vi "BRig_RT_start_v1,14.vi"() -> ()   [LabVIEW 2014]
uses:
  <vilib>/Platform/TimedLoop/XDataNode/XDataNode.xnode
  <vilib>/Platform/TimedLoop/XDataNode/nitl_modes.ctl
  <vilib>/Platform/TimedLoop/XDataNode/XDNodeRunTimeDep.lvlib
  <vilib>/Platform/TimedLoop/XDataNode/wakeup.ctl
  <vilib>/Platform/TimedLoop/XDataNode/timing_clust.ctl
  <vilib>/rvi/interface/nirviReadWriteControl/nirviReadWriteControl.xnode
  <vilib>/rvi/interface/Simulation/niFpgaSimulationCallBeginRW.vi
  <vilib>/rvi/errors/niLvFpgaAdjustHostInterfaceError.vi
  <vilib>/rvi/interface/nirviCloseFPGA/nirviCloseFPGA.xnode
  <vilib>/myRIO/Instrument Drivers/Utilities/Utilities.lvlib
  <vilib>/rvi/interface/nirviOpenFPGA/nirviOpenFPGA.xnode
  myRIO_BRig_RT__Case_Exp_stateList.ctl
  myRIO_BRig_RT__Case_NonExp_stateList.ctl
  NiFpgaLv.dll
  <vilib>/Utility/error.llb/Error Cluster From Error Code.vi
  <vilib>/WebDAVClient/Advanced/SessionHandle.ctl
  <vilib>/WebDAVClient/NI_WebDAV.lvlib
  <vilib>/Utility/file.llb/Read From Spreadsheet File (I64).vi
  <vilib>/Utility/file.llb/Write To Spreadsheet File (DBL).vi
  <vilib>/FPGAPlugInAG/Dynamic/niLvFpga_Close_Dynamic.vi
  BRig_FPGA_v3,94__build.lvbitx
  BRig_FPGA_v3,94.vi
  <vilib>/FPGAPlugInAG/myRIO-1900/niLvFpga_Open_myRIO-1900.vi
  <vilib>/rvi/interface/common/dynamic/niFpgaDynamicAddResources.vi
panel:
  in  "LaserFiber_V_l2":dbl
  in  "LaserFiber_V_l1":dbl
  out "Solenoid R":bool
  out "Solenoid L":bool
  out "Laser2":bool
  out "Laser1":bool
  out "FreeReward_c_R":u16
  out "FreeReward_c_L":u16
  in  "Laser2_LED":bool
  in  "Laser1_LED":bool
  in  "lick_Rising(F)_or_Falling(T)":bool
  out "T_ExpRun_min":dbl
  out "stop_TimedLoop":bool
  out "BTPR_avg_R":dbl
  out "T2R_avg_R":dbl
  out "BTPR_avg_L":dbl
  out "T2R_avg_L":dbl
  out "BTPR_block":u16
  out "T2R_block":u16
  in  "comm_WebDAV_connect":bool
  in  "I_sendData":bool
  in  "comm_TCP_connect":bool
  out "nRewards_total":u16 caption="# Rewards in Current Block"
  out "BUR_target":u16 caption="Target Trials Per Block"
  in  "input_Threshold_reset":bool
  out "nTrial":u16
  out "allReward_R":bool
  out "allReward_L":bool
  out "Threshold":bool
  out "tLoop":dbl format="%#_2g"
  out "L_Power_l2":dbl
  out "comm_TCP":bool
  in  "get_countPerMS":bool
  out "SolenoidReward":bool
  out "L_Power_l1":dbl caption="LaserPower"
  in  "Recording":bool
  out "FPGA_count2ms":dbl=159.0
  out "error out":errorcluster
  out "cSpout":enum16{"Left", "Right"}(ring) caption="Left or Right Spout"
  out "A4":u32 caption="LickCounter_Right"
  out "A2":u32 caption="LickCounter_Left"
  out "nRewards_Right":u16 caption="# Rewards Total (Right)"
  out "nRewards_Left":u16 caption="# Rewards Total (Left)"
  out "nRewards_cur":u16 caption="# Rewards in Current Block"
  out "TpB_target":u16 caption="Target Trials Per Block"
  out "cState_NonExp":T1 caption="WarmUp State"
  out "iBlock":u16 caption="Current Block"
  out "cState":T2 caption="Experimental State"
  out "iTrial":u16 caption="Current Trial"
  in  "Data Set Prefix":string="Exp1_TM2"
  out "comm_WebDAV":bool
  in  "Host Password":string="sabalab"
  in  "Host UserName":string="Test2"
  in  "STOP_abort":bool caption="Stop LabView\n(Stops myRio and FPGA)"
  in  "STOP_endBlock":bool caption="Stop Experiment\n@ End of Block"
  in  "STOP_endTrial":bool caption="Stop Experiment\n@ End of Trial"
  in  "START":bool caption="Start Experiment"
  # "Experimental Run"
  # "Recording Rig"
  # "FPGA Conversion\n[counts per ms]"
  # "RealTime Cycle\nShould be <5ms"
  # "STOP experiment at"
  # "Exp Run Time"
  # "Reset"
  # "min"
  # "Communication with Host"
  # "Lick Counter"
  # "Block Target"
  # "Give Water?\n(Reward)"
  # "# Blocks"
  # "Experimental State"
  # "Left/Right"
  # "# Trials"
  # "# Rewards"
  # "Left           Right"
  # "Bad Trials\nPost Reward"
  # "Trials 2 Reward"
  # "Direction\n(NonSpecific Licking)"
  # "Block"
  # "Laser1"
  # "Laser2"
  # "# Trials"
  # "# Rewards"
  # "Current\nBlock"
  # "L          R"
  # "Power [V]"
  # "avg L"
  # "Toggle\nLED"
  # "Total"
  # "# Rewards"
  # "Laser Trigger"
  # "# Trials"
  # "avg R"
  # "1          2"
  # "Fiber Angle\n[V]"
  # "Left           Right"
  # "FreeRewards"
  # "Solenoid Trigger"
  # "WarmUp State"
  # "Lick Detection\nRising (F) or Falling (T)"
  # "L          R"
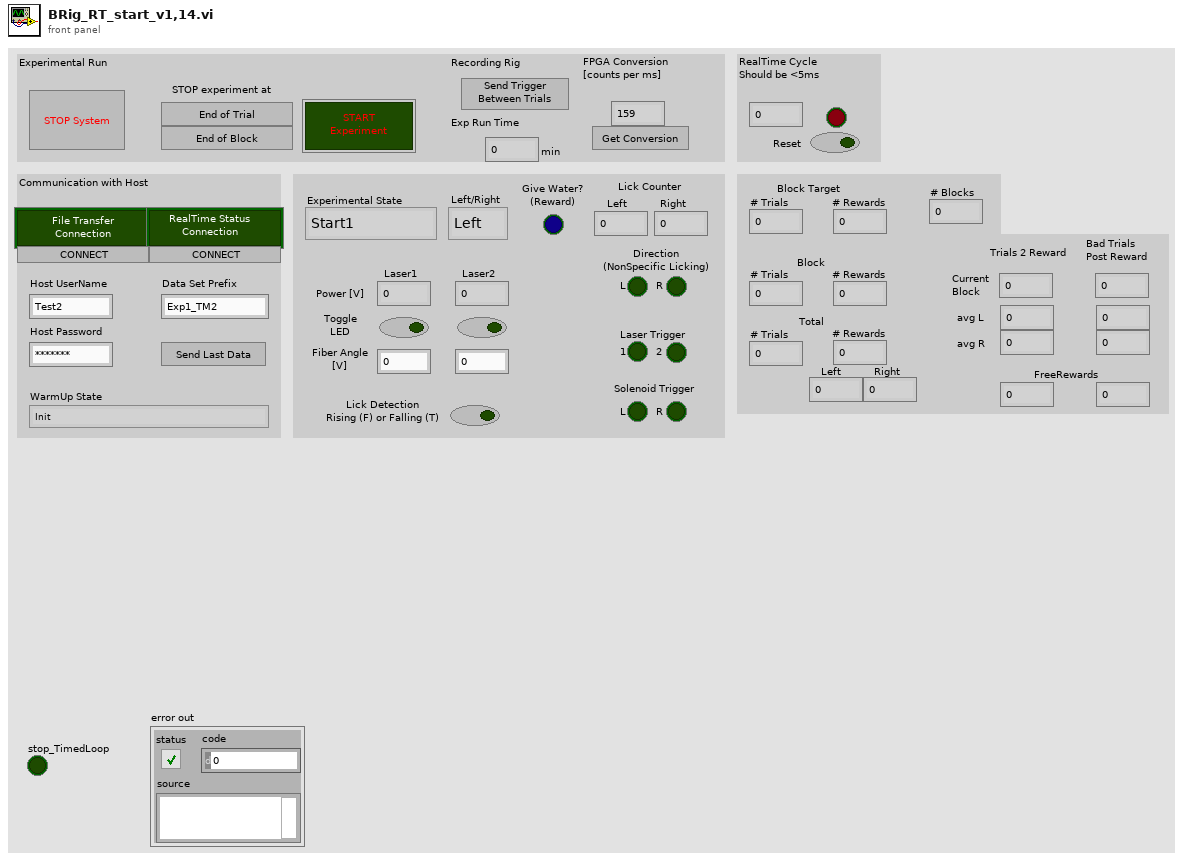
[diagram p1: front panel]
types:
  T1 = typedef "myRIO_BRig_RT__Case_NonExp_stateList.ctl" = enum16{"Init", "UploadSettings_pre", "UploadSettings_Read_dataExp", "UploadSettings_dataExp_1", "UploadSettings_dataExp_2", "UploadSettings_Read_dataLC", "UploadSettings_dataLC_1", "UploadSettings_dataLC_2", "UploadSettings_dataLC_3", "UploadSettings_dataLC_4", "UploadSettings_Read_dataMTrig", "UploadSettings_dataMTrig_1", "UploadSettings_post", "Idle_pre", "IdleEmpty", "IdleEmpty2", "IdleEmpty3", "IdleEmpty4", "Idle", "Idle_2", "Idle_3", "Idle_4", "Idle_5", "Idle_6", "Idle_post", "Cue_pre__pre", "Cue_pre", "Cue", "Cue_LED", "Cue_post", "RewardCalibration_pre", "RewardCalibration", "DispenseWater_pre__pre", "DispenseWater_pre", "DispenseWater", "DispenseWater_post", "TestConnection", "SendData", "Get_FPGA_count_per_ms", "End", "commTCP_connect"}
  T2 = typedef "myRIO_BRig_RT__Case_Exp_stateList.ctl" = enum16{"Start1", "Start2", "Start3", "saveSettings1", "saveSettings2", "saveSettings3", "saveSettings4", "saveSettings_LC_ENL_l1", "saveSettings_LC_ENL_l2", "saveSettings_LC_Cue_l1", "saveSettings_LC_Cue_l2", "saveSettings6_LC_l1_Other", "SaveSettings6_LC_l2_Other", "setSettings_Audio", "setSettings_Laser", "initBlock_pre", "initBlock", "initBlock2", "initBlock_post", "initTrial_pre", "initTrial", "initTrial2", "initTrial3", "initTrial4", "initTrial_LC_ENL1", "initTrial_LC_Cue1", "initTrial_LC_Cue1_2", "initTrial_LC_Sel", "initTrial_post", "ENL1_pre", "ENL1", "ENL1_post", "ENL1Penalty_pre", "ENL1Penalty", "ENL2_pre", "ENL2", "ENL2Penalty_pre", "ENL2Penalty", "Cue1_pre", "Cue1", "Cue1_post", "Cue1Penalty_pre", "Cue1Penalty", "Cue2_pre", "Cue2", "Cue2Penalty_pre", "Cue2Penalty", "Selection_pre", "Selection", "Select_post", "SelectReward_pre", "SelectReward", "SelectRewardPost_pre", "SelectRewardPost", "SelectWrong_pre", "SelectWrong", "SelectWrong_post", "SelectTimeout_pre", "SelectTimeout", "SelectTimeout_post", "endTrial_pre", "endTrial1", "endTrial2", "endTrial3", "endTrial_post", "endBlock_pre", "endBlock", "endBlock_post", "endExp", "commConnect", "commUpload_pre", "commUpload_dataBlock", "commUpload_dataCurrent", "commUpload_dataExp", "commUpload_dataLC", "commUpload_dataTrial", "commUpload_post", "saveData_pre", "saveData_dataBlock", "saveData_dataCurrent", "saveData_dataExp", "saveData_dataLC", "saveData_dataTrial", "saveData_post", "empty_endBlock1", "empty_endBlock2", "empty_endTrial1", "empty_endTrial2", "empty_endTrial3", "empty_endTrial4", "empty_endTrial5", "dummyState", "dummyState_endBlock", "FreeReward_pre", "FreeReward", "FreeRewardPost_pre", "FreeRewardPost"}
  T3 = enum8{"Enabled", "Disabled", "Disabled and Grayed Out"}
  T4 = typedef "NI_WebDAV.lvlib/SessionHandle.ctl" = refnum<k1>
  T5 = typedef "XDNodeRunTimeDep.lvlib/timing_clust.ctl" = cluster{"Expected End [f-1]":u64, "Actual End [f-1]":u64, "Finished Late? [f-1]":bool, "Expected End [i-1]":u64, "Actual End [i-1]":u64, "Finished Late? [i-1]":bool, "Expected Start [i]":u64, "Actual Start [i]":u64, "Expected Start [f]":u64, "Actual Start [f]":u64, "Source Name":string, "Structure Name":string, "Period":i64, "Deadline":i64, "Offset":i64, "Start":i64, "Priority":i32, "Timeout":i32, "Mode":T6, "Wakeup Reason":T7, "Error":errorcluster, "Source Type":string, "Secondary Source Type":string, "Global End Time":u64, "Global Start Time":u64, "Frame Duration":u64, "Iteration Duration":u64, "Assigned CPU":i32, "I/O Scan Engine Mode":u32}
  T6 = typedef "XDNodeRunTimeDep.lvlib/nitl_modes.ctl" = enum32{"No Change", "Process missed periods, maintain original phase", "Discard missed periods, maintain original phase", "Process missed periods, ignore original phase", "Discard missed periods, ignore original phase"}
  T7 = typedef "XDNodeRunTimeDep.lvlib/wakeup.ctl" = enum32{"Normal", "Aborted", "Asynchronous wakeup", "Timing source error", "Timed loop error", "Timeout"}
  T8 = cluster{"read mode":enum16{"polling", "blocking"}, "write mode":enum16{"polling", "blocking"}}
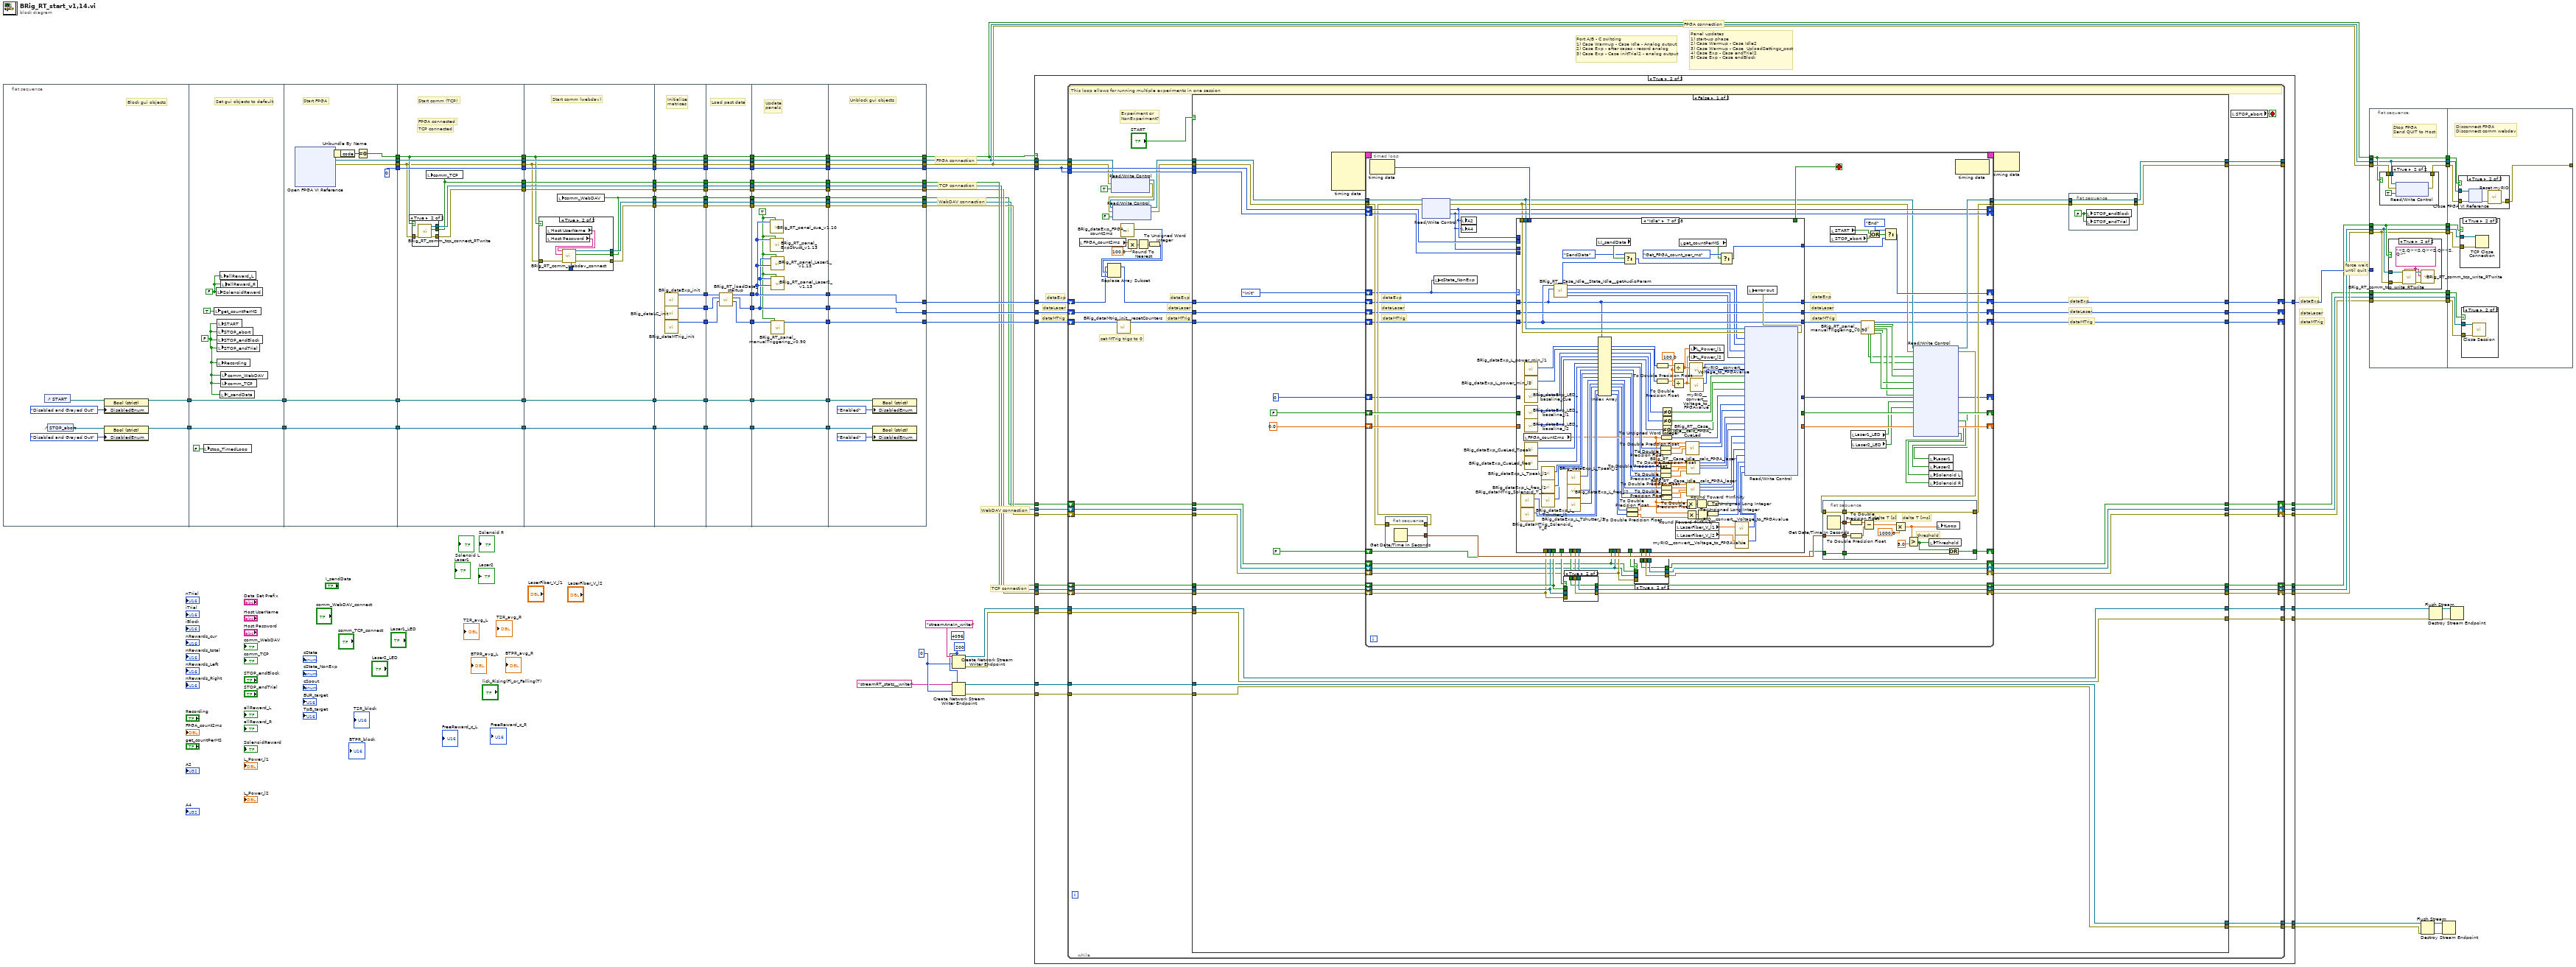
[diagram p0: block diagram]
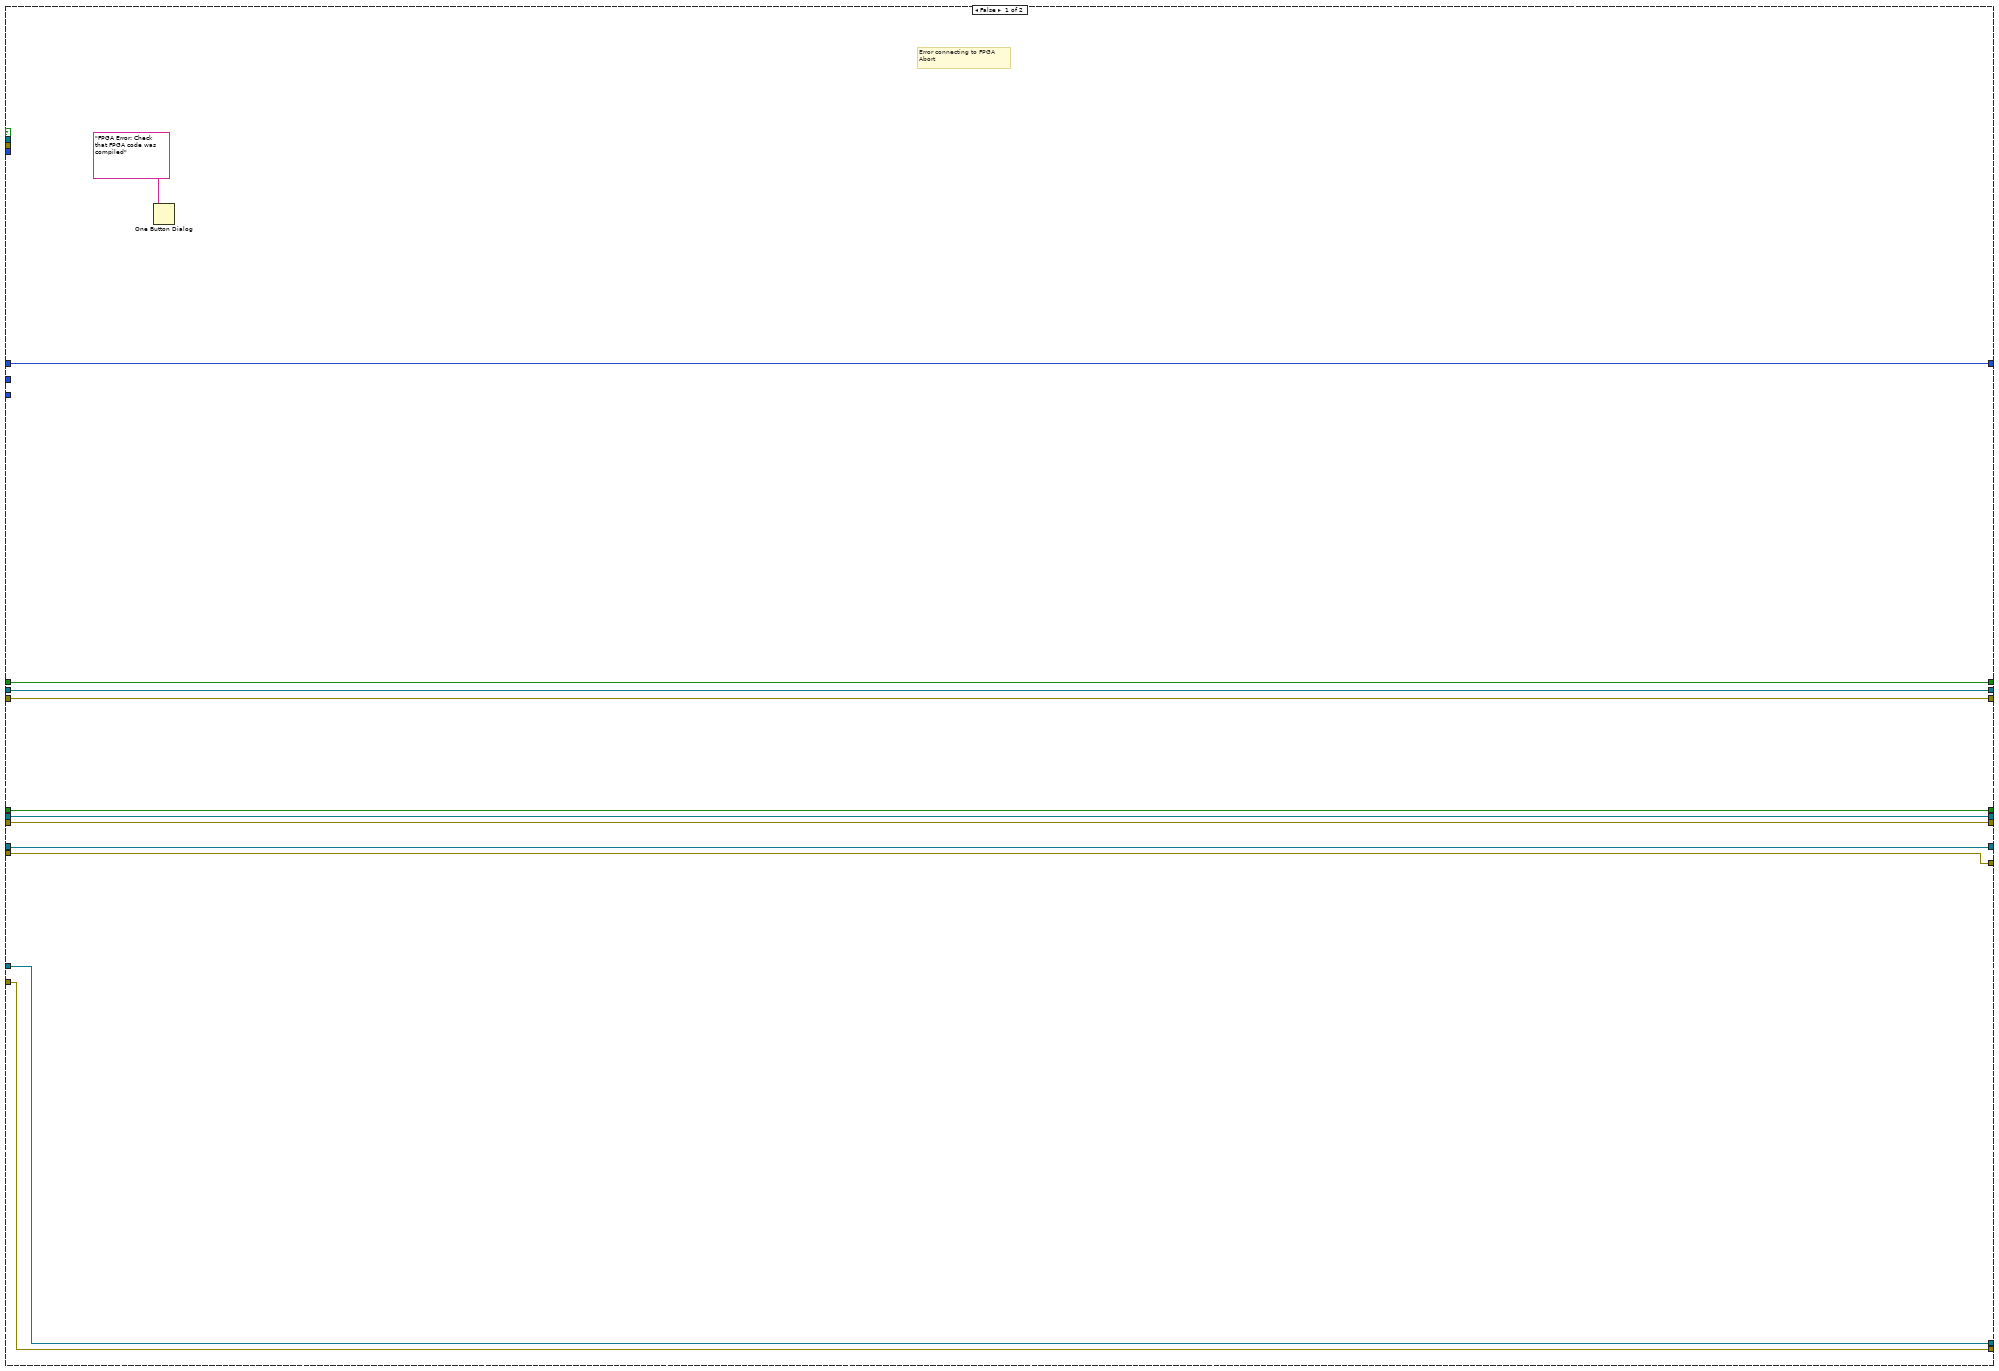
[diagram p2: hidden frame]
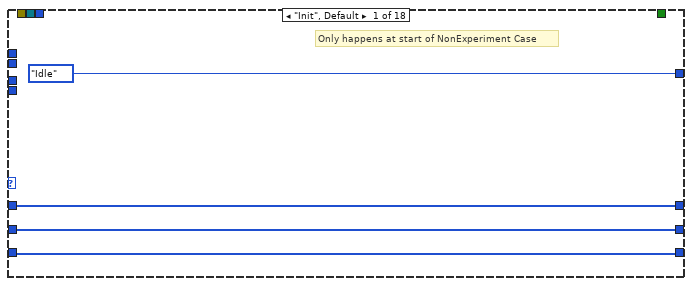
[diagram p5: hidden frame]
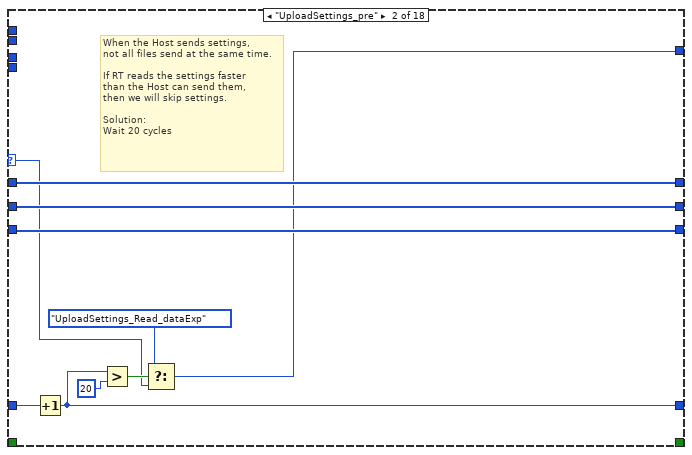
[diagram p6: hidden frame]
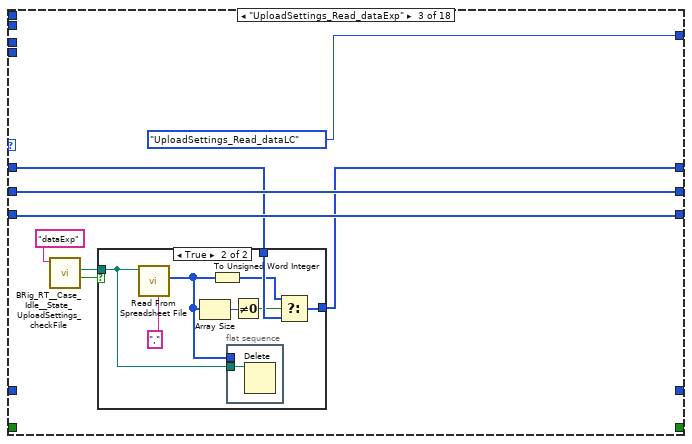
[diagram p7: hidden frame]
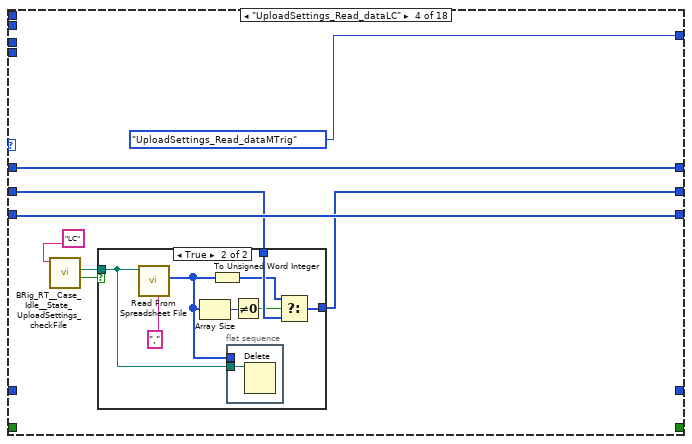
[diagram p9: hidden frame]
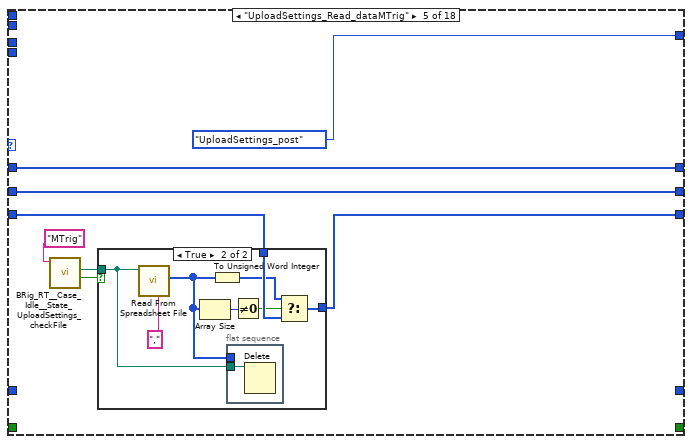
[diagram p11: hidden frame]
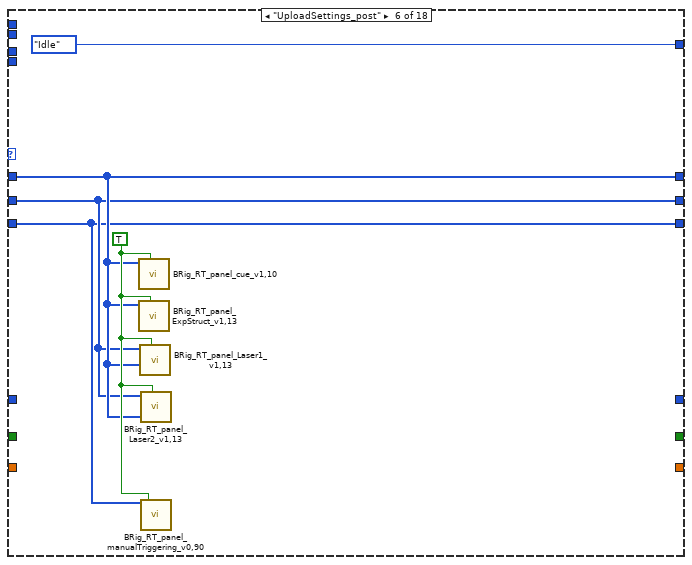
[diagram p13: hidden frame]
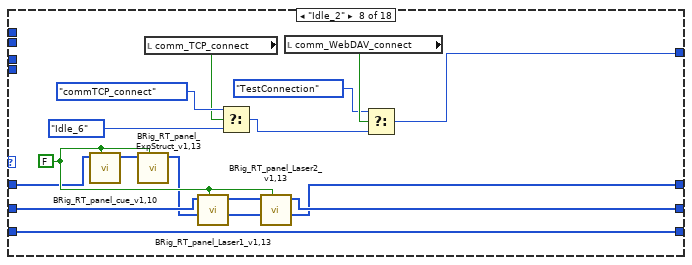
[diagram p14: hidden frame]
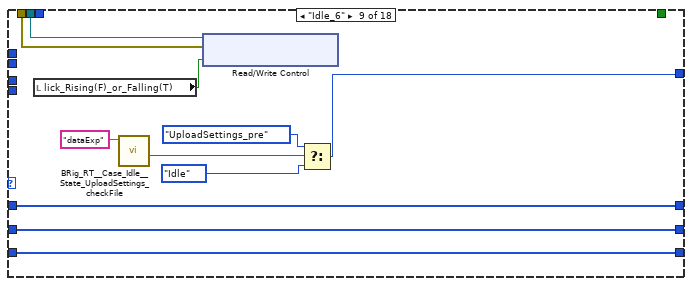
[diagram p15: hidden frame]
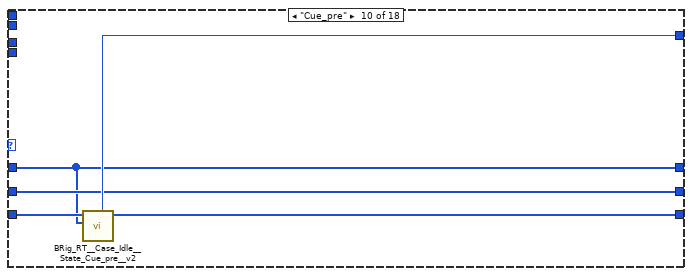
[diagram p16: hidden frame]
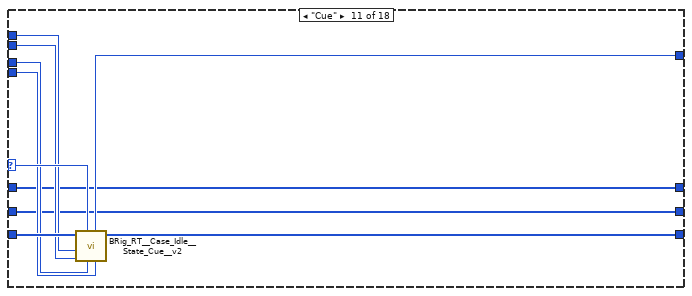
[diagram p17: hidden frame]
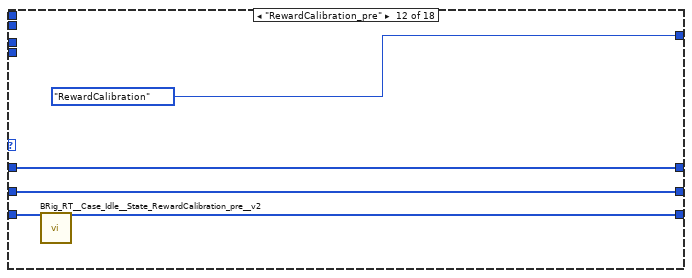
[diagram p18: hidden frame]
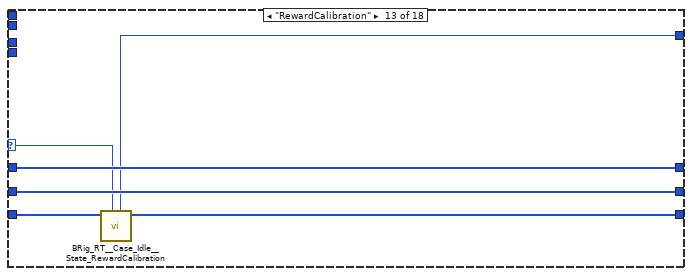
[diagram p19: hidden frame]
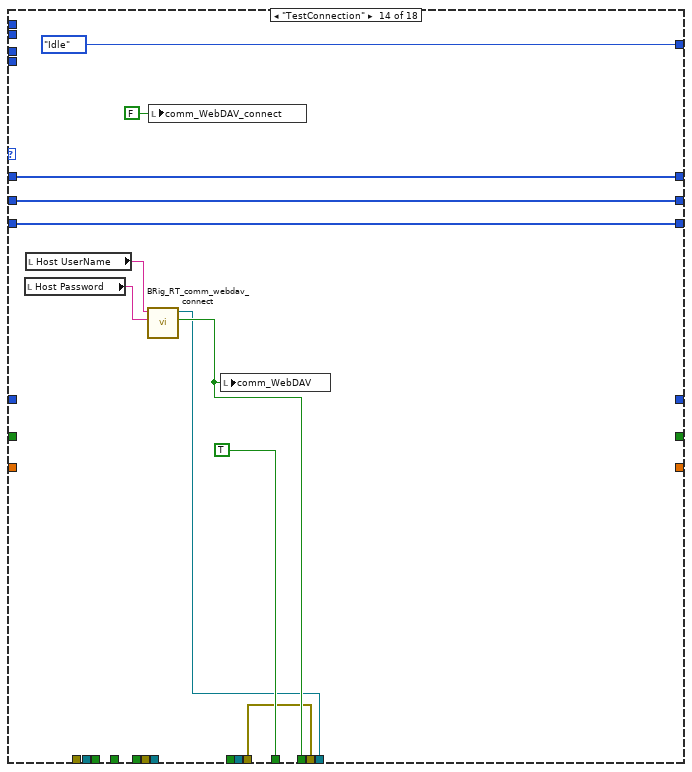
[diagram p20: hidden frame]
diagram:
  w8 = u16 0 ("element")
  (unwired) 4096 ("reader buffer size")
  w9 = 200 ("reader buffer size")
  # "Panel updates\n1) start-up phase\n2) Case Warmup - Case Idle2\n3) Case Warmup - Case  UploadSettings_post\n4) Case Exp - Case endTrial2\n5) Case Exp - Case endBlock"
  # "WebDAV connection"
  # "TCP connection"
  # "WebDAV connection"
  # "TCP connection"
  # "FPGA connection"
  # "FPGA connection"
  # "Port A/B - C switcing\n1) Case Warmup - Case Idle - Analog output\n2) Case Exp - after cases - record analog\n3) Case Exp - Case initTrial2 - analog output"
  # "force wait\nuntil quit"
  # "dataLaser"
  # "dataExp"
  # "dataMTrig"
  n1 = flat-sequence {
    tunnel: [w123] -> w106
    tunnel: [w122] -> w102
    tunnel: [w132] -> w107
    tunnel: w106 -> [w132]
    tunnel: [w131] -> w103
    tunnel: w102 -> [w131]
    tunnel: [w138] -> w120
    tunnel: [w140] -> w119
    tunnel: [u32 0] -> w118
    tunnel: [w136] -> w117
    tunnel: [w135] -> w108
    tunnel: w107 -> [w135]
    tunnel: [w134] -> w104
    tunnel: w103 -> [w134]
    tunnel: w120 -> [w146]
    tunnel: w119 -> [w149]
    tunnel: w118 -> [w148]
    tunnel: w117 -> [w147]
    tunnel: [w146] -> w116
    tunnel: [w149] -> w115
    tunnel: [w148] -> w114
    tunnel: [w147] -> w113
    tunnel: [w141] -> w112
    tunnel: [w145] -> w111
    tunnel: [w144] -> w110
    tunnel: [w143] -> w109
    tunnel: w108 -> [w143]
    tunnel: [w142] -> w105
    tunnel: w104 -> [w142]
    tunnel: w116 -> [w160]
    tunnel: w115 -> [w168]
    tunnel: w114 -> [w167]
    tunnel: w113 -> [w161]
    tunnel: w112 -> [w166]
    tunnel: w111 -> [w165]
    tunnel: w110 -> [w164]
    tunnel: [w160] -> w73
    tunnel: [w168] -> w72
    tunnel: [w167] -> w71
    tunnel: [w161] -> w70
    tunnel: [w166] -> w69
    tunnel: [w165] -> w68
    tunnel: [w164] -> w67
    tunnel: [w163] -> w66
    tunnel: w109 -> [w163]
    tunnel: [w162] -> w65
    tunnel: w105 -> [w162]
    tunnel: [w159] -> w64
    tunnel: [w157] -> w63
    tunnel: [w158] -> w62
    tunnel: w73 -> [w193]
    tunnel: [w193] -> w61
    tunnel: w72 -> [w192]
    tunnel: [w192] -> w60
    tunnel: w71 -> [w191]
    tunnel: [w191] -> w59
    tunnel: w70 -> [w190]
    tunnel: [w190] -> w58
    tunnel: w69 -> [w189]
    tunnel: [w189] -> w57
    tunnel: w68 -> [w188]
    tunnel: [w188] -> w56
    tunnel: w67 -> [w187]
    tunnel: [w187] -> w55
    tunnel: w66 -> [w186]
    tunnel: [w186] -> w54
    tunnel: w65 -> [w185]
    tunnel: [w185] -> w53
    tunnel: w64 -> [w184]
    tunnel: [w184] -> w52
    tunnel: w63 -> [w183]
    tunnel: [w183] -> w51
    tunnel: w62 -> [w182]
    tunnel: [w182] -> w50
    tunnel: [w181] -> w49
    tunnel: [w180] -> w48
    tunnel: [w179] -> w47
    tunnel: w61 -> [w211]
    tunnel: [w211] -> w46
    tunnel: w60 -> [w210]
    tunnel: [w210] -> w44
    tunnel: w59 -> [w209]
    tunnel: [w209] -> w42
    tunnel: w58 -> [w208]
    tunnel: [w208] -> w40
    tunnel: w57 -> [w207]
    tunnel: [w207] -> w38
    tunnel: w56 -> [w206]
    tunnel: [w206] -> w36
    tunnel: w55 -> [w205]
    tunnel: [w205] -> w34
    tunnel: w54 -> [w204]
    tunnel: [w204] -> w32
    tunnel: w53 -> [w203]
    tunnel: [w203] -> w30
    tunnel: w52 -> [w202]
    tunnel: [w202] -> w28
    tunnel: w51 -> [w201]
    tunnel: [w201] -> w26
    tunnel: w50 -> [w200]
    tunnel: [w200] -> w24
    tunnel: w49 -> [w195]
    tunnel: [w194] -> w22
    tunnel: w48 -> [w197]
    tunnel: [w196] -> w20
    tunnel: w47 -> [w199]
    tunnel: [w198] -> w19
    tunnel: w46 -> [w228]
    tunnel: [w228] -> w45
    tunnel: w44 -> [w227]
    tunnel: [w227] -> w43
    tunnel: w42 -> [w226]
    tunnel: [w226] -> w41
    tunnel: w40 -> [w225]
    tunnel: [w225] -> w39
    tunnel: w38 -> [w224]
    tunnel: [w224] -> w37
    tunnel: w36 -> [w223]
    tunnel: [w223] -> w35
    tunnel: w34 -> [w222]
    tunnel: [w222] -> w33
    tunnel: w32 -> [w221]
    tunnel: [w221] -> w31
    tunnel: w30 -> [w220]
    tunnel: [w220] -> w29
    tunnel: w28 -> [w219]
    tunnel: [w219] -> w27
    tunnel: w26 -> [w218]
    tunnel: [w218] -> w25
    tunnel: w24 -> [w217]
    tunnel: [w217] -> w23
    tunnel: w22 -> [w214]
    tunnel: [w213] -> w21
    tunnel: w20 -> [w215]
    tunnel: w19 -> [w216]
    tunnel: [w216] -> w18
    tunnel: [w215] -> w17
    tunnel: [w235] -> w83
    tunnel: [w236] -> w84
    tunnel: [w237] -> w85
    tunnel: [w242] -> w89
    tunnel: [w243] -> w121
    tunnel: [w244] -> w96
    tunnel: [w245] -> w95
    tunnel: w45 -> [w245]
    tunnel: w43 -> [w244]
    tunnel: w41 -> [w243]
    tunnel: w39 -> [w242]
    tunnel: w37 -> [w237]
    tunnel: w35 -> [w236]
    tunnel: w33 -> [w235]
    tunnel: w31 -> [w239]
    tunnel: w29 -> [w238]
    tunnel: w27 -> [w233]
    tunnel: w25 -> [w234]
    tunnel: w23 -> [w232]
    tunnel: [w234] -> w77
    tunnel: [w233] -> w78
    tunnel: [w232] -> w79
    tunnel: [w229] -> w92
    tunnel: [w230] -> w91
    tunnel: [w231] -> w90
    tunnel: w21 -> [w231]
    tunnel: w18 -> [w229]
    tunnel: w17 -> [w230]
    frame #0 {
      # "Block gui objects"
      n2 = control-ref of="START"() -> (w127:refnum<vi>)
      n3 = control-ref of="STOP_abort"() -> (w124:refnum<vi>)
      n4 = property class="Bool (strict)"(reference=w127, "DisabledEnum"=T3."Disabled and Grayed Out" ("Disabled")) -> (reference out=w123:refnum<vi>)  [unwired: 1 in, 1 out]
      n5 = property class="Bool (strict)"(reference=w124, "DisabledEnum"=T3."Disabled and Grayed Out" ("Disabled")) -> (reference out=w122:refnum<vi>)  [unwired: 1 in, 1 out]
    }
    frame #1 {
      w129 = FALSE ("SolenoidReward")
      w130 = FALSE
      # "Set gui objects to default"
      n6 = local write "stop_TimedLoop"(FALSE ("stop_TimedLoop")) -> ()
      n7 = local write "get_countPerMS"(TRUE ("get_countPerMS")) -> ()
      n8 = local write "SolenoidReward"(w129) -> ()
      n9 = local write "START"(w130) -> ()
      n10 = local write "STOP_abort"(w130) -> ()
      n11 = local write "STOP_endBlock"(w130) -> ()
      n12 = local write "STOP_endTrial"(w130) -> ()
      n13 = local write "Recording"(w130) -> ()
      n14 = local write "allReward_L"(w129) -> ()
      n15 = local write "I_sendData"(w130) -> ()
      n16 = local write "comm_WebDAV"(w130) -> ()
      n17 = local write "comm_TCP"(w130) -> ()
      n18 = local write "allReward_R"(w129) -> ()
    }
    frame #2 {
      # "Start FPGA"
      n19 = xnode "Open FPGA VI Reference"() -> ("FPGA VI Reference Out"=w140:refnum<k20>, "error out"=w138:errorcluster)  [unwired: 2 in]
      n20 = Unbundle By Name(w138) -> ("code"=w137:i32)
      n21 = Equal To 0?(x=w137) -> (x = 0?=w136:bool)
    }
    frame #3 {
      # "TCP connected"
      # "Start comm (TCP)"
      # "FPGA connected"
      n22 = case shown="True" w147 {
        selector: w147 -> [w150 _]
        tunnel: w146 -> [w152 w156]
        tunnel: [refnum<k5> refnum ("output_hTCP") w155] -> w145
        tunnel: [w150 w154] -> w141
        tunnel: [w152 w153] -> w144
        frame False {
        }
        frame True {
          n23 = call "BRig_RT_comm_tcp_connect_RTwrite.vi"("input_error"=w156) -> ("output_error"=w153:errorcluster, "output_connected"=w154:bool, "output_hTCP"=w155:refnum<k5>)  [unwired: 8 in]
        }
      }
      n24 = local write "comm_TCP"(w141) -> ()
    }
    frame #4 {
      # "Start comm (webdav)"
      n25 = case shown="True" w161 {
        selector: w161 -> [w170 _]
        tunnel: [w169 w176] -> w159
        tunnel: [w170 w175] -> w157
        tunnel: w160 -> [w171 w174]
        tunnel: [w171 w173] -> w158
        tunnel: [_ w172] -> _
        frame False {
          w169 = T4 refnum items=["Session NI_WebDAV"] ("output_hSession")
        }
        frame True {
          n26 = local read "Host UserName"() -> (w177:string)
          n27 = local read "Host Password"() -> (w178:string)
          n28 = call "BRig_RT_comm_webdav_connect.vi"("input_error"=w174, "input_password"=w178, "input_username"=w177) -> ("output_error"=w173:errorcluster, "output_Iconnected"=w175:bool, "output_hSession"=w176:T4, "output_code"=w172:u8)  [unwired: 5 in]
        }
      }
      n29 = local write "comm_WebDAV"(w157) -> ()
    }
    frame #5 {
      # "Initialize\nmatrices"
      n30 = call "BRig_dataExp_init.vi"() -> ("output_dataExp"=w179:u16[])  [unwired: 11 in]
      n31 = call "BRig_dataLC_init.vi"() -> ("output_dataLC"=w180:u16[])  [unwired: 11 in]
      n32 = call "BRig_dataMTrig_init.vi"() -> ("output_dataMTrig"=w181:u16[])  [unwired: 5 in]
    }
    frame #6 {
      # "Load past data"
      n33 = call "BRig_RT_loadData_startup.vi"("input_dataMTrig"=w195, "input_dataLC"=w197, "input_dataExp"=w199) -> ("output_dataMTrig"=w194:u16[], "output_dataLC"=w196:u16[], "output_dataExp"=w198:u16[])  [unwired: 6 in]
    }
    frame #7 {
      w212 = TRUE ("input_setValues")
      # "Update\npanels"
      n34 = call "BRig_RT_panel_cue_v1,10.vi"("input_setValues"=w212, "input_dataExp"=w216) -> ()  [unwired: 9 in, 1 out]
      n35 = call "BRig_RT_panel_ExpStruct_v1,13.vi"("input_setValues"=w212, "input_dataExp"=w216) -> ()  [unwired: 9 in, 1 out]
      n36 = call "BRig_RT_panel_Laser1_v1,13.vi"("input_setValues"=w212, "input_dataExp"=w216, "input_dataLC"=w215) -> ()  [unwired: 7 in, 2 out]
      n37 = call "BRig_RT_panel_Laser2_v1,13.vi"("input_setValues"=w212, "input_dataExp"=w216, "input_dataLC"=w215) -> ()  [unwired: 7 in, 2 out]
      n38 = call "BRig_RT_panel_manualTriggering_v0,90.vi"("input_dataMTrig"=w214, "input_setValues"=w212) -> ("output_dataMTrig"=w213:u16[])  [unwired: 10 in, 7 out]
    }
    frame #8 {
      # "Unblock gui objects"
      n39 = property class="Bool (strict)"(reference=w239, "DisabledEnum"=T3."Enabled" ("Disabled")) -> ()  [unwired: 1 in, 2 out]
      n40 = property class="Bool (strict)"(reference=w238, "DisabledEnum"=T3."Enabled" ("Disabled")) -> ()  [unwired: 1 in, 2 out]
    }
  }
  n41 = Create Network Stream Writer Endpoint(7:w9, 9:w8, 11:"streamAnaIn_writer" ("reader name")) -> (0:w10:errorcluster, 3:w11:refnum<k21>)  [unwired: 4 in]
  n42 = Create Network Stream Writer Endpoint(7:w9, 9:w8, 11:"streamRT_stats__writer" ("writer name")) -> (0:w5:errorcluster, 3:w6:refnum<k21>)  [unwired: 4 in]
  n43 = case shown="True" w89 {
    tunnel: w121 -> [_ w284]
    tunnel: w96 -> [_ w283]
    tunnel: w95 -> [_ w282]
    tunnel: [w257 w281] -> w93
    tunnel: w92 -> [w257 w280]
    tunnel: w91 -> [_ w279]
    tunnel: w90 -> [_ w278]
    tunnel: w85 -> [w256 w277]
    tunnel: w84 -> [w255 w276]
    tunnel: w83 -> [w254 w275]
    tunnel: [w256 w274] -> w82
    tunnel: [w255 w273] -> w81
    tunnel: [w254 w272] -> w80
    tunnel: w79 -> [w253 w271]
    tunnel: w78 -> [w252 w270]
    tunnel: w77 -> [w251 w269]
    tunnel: [w253 w268] -> w76
    tunnel: [w252 w267] -> w75
    tunnel: [w251 w266] -> w74
    tunnel: [w250 w265] -> w14
    tunnel: [w249 w264] -> w13
    tunnel: w11 -> [w250 w263]
    tunnel: w10 -> [w249 w262]
    tunnel: w6 -> [w247 w261]
    tunnel: w5 -> [w246 w260]
    tunnel: [w247 w259] -> w2
    tunnel: [w246 w258] -> w1
    frame False {
      # "Error connecting to FPGA\nAbort"
      n44 = One Button Dialog(message="FPGA Error: Check that FPGA code was compiled") -> ()  [unwired: 1 in, 1 out]
    }
    frame True {
      # "dataExp"
      # "dataLaser"
      # "dataMTrig"
      n45 = while {
        tunnel: w283 -> [w322]
        tunnel: w282 -> [w327]
        tunnel: w284 -> [w330]
        tunnel: w284 -> [w329]
        tunnel: [w320] -> _
        tunnel: [w319] -> _
        shift-right: [w318] -> _
        shift-left: w278 -> [w315]
        shift-right: [w316] -> _
        shift-left: w279 -> [w317]
        shift-right: [w286] -> w281
        shift-left: w280 -> [w295]
        shift-right: [w310] -> w274
        shift-left: w277 -> [w313]
        shift-right: [w309] -> w273
        shift-left: w276 -> [w312]
        shift-right: [w308] -> w272
        shift-left: w275 -> [w311]
        shift-right: [w304] -> w268
        shift-left: w271 -> [w307]
        shift-right: [w303] -> w267
        shift-left: w270 -> [w306]
        shift-right: [w302] -> w266
        shift-left: w269 -> [w305]
        tunnel: [w294] -> w265
        tunnel: [w293] -> w264
        tunnel: w263 -> [w292]
        tunnel: w262 -> [w291]
        tunnel: w261 -> [w290]
        tunnel: w260 -> [w289]
        tunnel: [w288] -> w259
        tunnel: [w287] -> w258
        stop <- w328 stop-if-true
        # "set MTrig trigs to 0"
        # "dataExp"
        # "dataLaser"
        # "dataMTrig"
        # "Experiment or\nNonExperiment?"
        # "This loop allows for running multiple experiments in one session"
        n46 = local read "FPGA_count2ms"() -> (w299:dbl)
        n47 = xnode "Read/Write Control"("FPGA VI Reference In"=w322, "error in"=w327, "Counts_Reset"=TRUE) -> ("FPGA VI Reference Out"=w324:refnum<k20>, "error out"=w325:errorcluster)
        n48 = xnode "Read/Write Control"("FPGA VI Reference In"=w324, "error in"=w325, "Counts_Reset"=FALSE) -> ("FPGA VI Reference Out"=w321:refnum<k20>, "error out"=w323:errorcluster)
        n49 = call "BRig_dataMtrig_init__resetCounters.vi"("input_dataMTrig"=w315) -> ("output_dataMTrig"=w314:u16[])  [unwired: 10 in]
        n50 = call "BRig_dataExp_FPGA_count2ms.vi"() -> ("output_FPGA_count2ms"=w300:i32)  [unwired: 11 in]
        n51 = Multiply(x=w299, y=100.0) -> (x*y=w297:dbl)
        n52 = Round To Nearest(number=w297) -> (nearest integer value=w296:dbl)
        n53 = To Unsigned Word Integer(number=w296) -> (unsigned 16bit integer=w301:u16)
        n54 = Replace Array Subset(array=w295, new element=w301, index=w300) -> (w285:u16[])
        n55 = case shown="False" "START" {
          tunnel: w330 -> [w366 w945]
          tunnel: w329 -> [w365 w944]
          tunnel: w323 -> [w363 w933]
          tunnel: w321 -> [w364 w934]
          tunnel: [w361 w942] -> w320
          tunnel: [w359 w911] -> w319
          tunnel: w314 -> [w355 w931]
          tunnel: [w354 w917] -> w318
          tunnel: w317 -> [w353 w881]
          tunnel: w285 -> [w333 w834]
          tunnel: [w352 w916] -> w316
          tunnel: [w351 w915] -> w286
          tunnel: w313 -> [w350 w925]
          tunnel: w312 -> [w349 w924]
          tunnel: w311 -> [w348 w923]
          tunnel: [w347 w900] -> w310
          tunnel: [w346 w899] -> w309
          tunnel: [w345 w898] -> w308
          tunnel: w307 -> [w344 w880]
          tunnel: w306 -> [w343 w879]
          tunnel: w305 -> [w342 w878]
          tunnel: [w341 w907] -> w304
          tunnel: [w340 w906] -> w303
          tunnel: [w339 w908] -> w302
          tunnel: w292 -> [w337 w839]
          tunnel: w291 -> [w336 w838]
          tunnel: [w337 w837] -> w294
          tunnel: [w336 w836] -> w293
          tunnel: w290 -> [w335 w830]
          tunnel: w289 -> [w334 w831]
          tunnel: [w335 w825] -> w288
          tunnel: [w334 w824] -> w287
          frame False {
            # "dataExp"
            # "dataLaser"
            # "dataMTrig"
            n56 = node-c288() -> (w369:T5)  [unwired: 4 in]
            n57 = timed-loop {
              timing: w369 -> [_]
              timing-out: [_] -> w368
              shift-right: [w437] -> _
              shift-left: myRIO_BRig_RT__Case_NonExp_stateList."Init" ("Enum") -> [w406]
              shift-right: [w435] -> _
              shift-left: w366 -> [w436]
              shift-right: [w433] -> _
              shift-left: w365 -> [w434]
              tunnel: [w443] -> w362
              tunnel: [w419] -> w360
              tunnel: w363 -> [w426]
              tunnel: w364 -> [w444]
              shift-right: [w429] -> _
              shift-left: FALSE -> [w430]
              shift-right: [w427] -> _
              shift-left: 0.0 -> [w428]
              shift-right: [w416] -> _
              shift-left: FALSE -> [w417]
              shift-right: [w415] -> w354
              shift-left: w355 -> [w407]
              shift-right: [w401] -> w351
              shift-left: w333 -> [w404]
              shift-right: [w402] -> w352
              shift-left: w353 -> [w403]
              shift-right: [w400] -> w347
              shift-left: w350 -> [w396]
              shift-right: [w399] -> w346
              shift-left: w349 -> [w395]
              shift-right: [w398] -> w345
              shift-left: w348 -> [w394]
              shift-right: [w384] -> w341
              shift-left: w344 -> [w390]
              shift-right: [w385] -> w340
              shift-left: w343 -> [w389]
              shift-right: [w386] -> w339
              shift-left: w342 -> [w388]
              shift-right: [w379] -> _
              shift-left: u16 0 ("y") -> [w380]
              stop <- w446 stop-if-true
              # "dataExp"
              # "dataLaser"
              # "dataExp"
              # "dataLaser"
              # "dataMTrig"
              # "dataMTrig"
              n58 = node-c288() -> (w445:i64)  [unwired: 1 in]
              n59 = flat-sequence {
                tunnel: w426 -> [w475]
                tunnel: [w476] -> w418
                tunnel: [w475] -> w425
                frame #0 {
                  n60 = Get Date/Time In Seconds() -> (seconds since 1Jan1904=w476:timestamp)
                }
              }
              n61 = xnode "Read/Write Control"("FPGA VI Reference In"=w444, "error in"=w425) -> ("FPGA VI Reference Out"=w432:refnum<k20>, "error out"=w431:errorcluster, "A2_LickL"=w435:u32, "A4_LickR"=w433:u32)
              n62 = local write "cState_NonExp"(w406) -> ()
              n63 = local write "A2"(w435) -> ()
              n64 = local write "A4"(w433) -> ()
              n65 = case shown="\"Idle\"" w406 {
                selector: w406 -> [_ w483 _ _ _ _ _ _ _ _ w678 _ w686 _ _ w730 w773 w779]
                tunnel: [myRIO_BRig_RT__Case_NonExp_stateList."Idle" ("Enum") w484 myRIO_BRig_RT__Case_NonExp_stateList."UploadSettings_Read_dataLC" ("t") myRIO_BRig_RT__Case_NonExp_stateList."UploadSettings_Read_dataMTrig" ("t") myRIO_BRig_RT__Case_NonExp_stateList."UploadSettings_post" ("t") myRIO_BRig_RT__Case_NonExp_stateList."Idle" ("t") w571 w641 w661 w667 w676 myRIO_BRig_RT__Case_NonExp_stateList."RewardCalibration" ("Enum") w685 myRIO_BRig_RT__Case_NonExp_stateList."Idle" ("Enum") myRIO_BRig_RT__Case_NonExp_stateList."Idle" ("Enum") w729 w773 w780] -> w438
                tunnel: [w479 w490 w498 w516 w530 w545 w583 w653 w659 w668 w677 w680 w687 w701 w713 w739 w771 w788] -> w405
                tunnel: [_ _ _ _ _ _ _ _ _ _ _ _ _ _ _ _ TRUE _] -> w446
                tunnel: w407 -> [w479 w490 w498 w516 w527 w545 w583 w653 w659 w669 w679 w681 w688 w701 w713 w739 w771 w788]
                tunnel: w445 -> [_ _ _ _ _ _ _ _ _ _ _ _ _ _ _ _ _ _]
                tunnel: w436 -> [_ _ _ _ _ _ _ _ _ _ w674 _ _ _ _ _ _ _]
                tunnel: w435 -> [_ _ _ _ _ _ _ _ _ _ w675 _ _ _ _ _ _ _]
                tunnel: w434 -> [_ _ _ _ _ _ _ _ _ _ w672 _ _ _ _ _ _ _]
                tunnel: w433 -> [_ _ _ _ _ _ _ _ _ _ w673 _ _ _ _ _ _ _]
                tunnel: w432 -> [_ _ _ _ _ _ w636 _ w656 _ _ _ _ _ _ w734 _ _]
                tunnel: w431 -> [_ _ _ _ _ _ w635 _ w655 _ _ _ _ _ _ w733 _ _]
                tunnel: w430 -> [_ _ _ _ _ _ _ _ _ _ _ _ _ _ _ w738 _ _]
                tunnel: [_ _ _ _ _ _ _ _ _ _ _ _ _ _ _ TRUE _ _] -> w429
                tunnel: w428 -> [_ _ _ _ _ _ _ _ _ _ _ _ _ _ _ w736 _ _]
                tunnel: [_ _ _ _ _ _ _ _ _ _ _ _ _ _ _ w735 _ _] -> w427
                tunnel: w404 -> [w477 w488 w493 w515 w534 w547 w582 w640 w657 w665 w670 w683 w689 w698 w710 w726 w769 w786]
                tunnel: w403 -> [w478 w489 w497 w509 w531 w546 w584 w652 w658 w666 w671 w682 w690 w699 w711 w727 w770 w787]
                tunnel: [w478 w489 w497 w512 w531 w546 w584 w648 w658 w666 w671 w682 w690 w699 w711 w727 w770 w787] -> w402
                tunnel: [w477 w488 w492 w515 w534 w547 w582 w637 w657 w665 w670 w683 w689 w698 w710 w726 w769 w786] -> w401
                tunnel: [_ _ _ _ _ _ _ _ _ _ _ _ _ _ _ _ _ TRUE] -> w397
                tunnel: w396 -> [_ _ _ _ _ _ _ _ _ _ _ _ _ _ w704 _ _ w785]
                tunnel: w395 -> [_ _ _ _ _ _ _ _ _ _ _ _ _ _ w706 _ _ w781]
                tunnel: w394 -> [_ _ _ _ _ _ _ _ _ _ _ _ _ _ w705 _ _ w784]
                tunnel: [_ _ _ _ _ _ _ _ _ _ _ _ _ _ _ _ _ w783] -> w393
                tunnel: [_ _ _ _ _ _ _ _ _ _ _ _ _ _ _ _ _ w782] -> w392
                tunnel: [_ _ _ _ _ _ _ _ _ _ _ _ _ _ _ _ _ w774] -> w391
                tunnel: w388 -> [_ _ _ _ _ _ _ _ _ _ _ _ _ _ w703 _ _ _]
                tunnel: w389 -> [_ _ _ _ _ _ _ _ _ _ _ _ _ _ w709 _ _ _]
                tunnel: w390 -> [_ _ _ _ _ _ _ _ _ _ _ _ _ w691 w708 _ _ _]
                tunnel: [_ _ _ _ _ _ _ _ _ _ _ _ _ TRUE _ _ _ _] -> w387
                tunnel: [_ _ _ _ _ _ _ _ _ _ _ _ _ w693 _ _ _ _] -> w383
                tunnel: [_ _ _ _ _ _ _ _ _ _ _ _ _ w691 _ _ _ _] -> w382
                tunnel: [_ _ _ _ _ _ _ _ _ _ _ _ _ w692 _ _ _ _] -> w381
                tunnel: w380 -> [_ w482 _ _ _ _ _ _ _ _ _ _ _ _ _ _ _ _]
                tunnel: [_ w481 _ _ _ _ _ _ _ _ _ _ _ _ _ _ _ _] -> w379
                frame "Init", Default {
                  # "Only happens at start of NonExperiment Case"
                }
                frame "UploadSettings_pre" {
                  # "When the Host sends settings,\nnot all files send at the same time.\n\nIf RT reads the settings faster\nthan the Host can send them,\nthen we will skip settings.\n\nSolution:\nWait 20 cycles"
                  n66 = Increment(x=w482) -> (x+1=w481:u16)
                  n67 = Greater?(x=w481, y=u16 20) -> (0:w486:bool)
                  n68 = Select(t=myRIO_BRig_RT__Case_NonExp_stateList."UploadSettings_Read_dataExp", s=w486, f=w483) -> (s? t:f=w484:T1)
                }
                frame "UploadSettings_Read_dataExp" {
                  n69 = call "BRig_RT__Case_Idle__State_UploadSettings_checkFile.vi"("input_dataName"="dataExp") -> ("output_Iexist"=w495:bool, "output_dataPath"=w494:path)  [unwired: 9 in]
                  n70 = case shown="True" w495 {
                    tunnel: w494 -> [_ w501]
                    tunnel: w493 -> [w499 w505]
                    tunnel: [w499 w503] -> w492
                    frame False {
                    }
                    frame True {
                      n71 = call-poly <vilib>:"Read From Spreadsheet File.vi"("delimiter (\\t)"="," ("delimiter (\\t)"), "file path (dialog if empty)"=w501) -> ("first row"=w500:i64[])  [unwired: 5 in, 4 out]
                      n72 = Array Size(array=w500) -> (size(s)=w506:i32)
                      n73 = To Unsigned Word Integer(number=w500) -> (unsigned 16bit integer=w504:u16[])
                      n74 = flat-sequence {
                        tunnel: w501 -> [w508]
                        tunnel: w500 -> [_]
                        frame #0 {
                          n75 = Delete(path (use dialog)=w508) -> ()  [unwired: 4 in, 3 out]
                        }
                      }
                      n76 = Not Equal To 0?(x=w506) -> (x != 0?=w502:bool)
                      n77 = Select(t=w504, s=w502, f=w505) -> (s? t:f=w503:u16[])
                    }
                  }
                }
                frame "UploadSettings_Read_dataLC" {
                  n78 = call "BRig_RT__Case_Idle__State_UploadSettings_checkFile.vi"("input_dataName"="LC") -> ("output_Iexist"=w510:bool, "output_dataPath"=w511:path)  [unwired: 9 in]
                  n79 = case shown="True" w510 {
                    tunnel: w511 -> [_ w519]
                    tunnel: w509 -> [w517 w523]
                    tunnel: [w517 w521] -> w512
                    frame False {
                    }
                    frame True {
                      n80 = call-poly <vilib>:"Read From Spreadsheet File.vi"("delimiter (\\t)"="," ("delimiter (\\t)"), "file path (dialog if empty)"=w519) -> ("first row"=w518:i64[])  [unwired: 5 in, 4 out]
                      n81 = Array Size(array=w518) -> (size(s)=w524:i32)
                      n82 = To Unsigned Word Integer(number=w518) -> (unsigned 16bit integer=w522:u16[])
                      n83 = flat-sequence {
                        tunnel: w519 -> [w526]
                        tunnel: w518 -> [_]
                        frame #0 {
                          n84 = Delete(path (use dialog)=w526) -> ()  [unwired: 4 in, 3 out]
                        }
                      }
                      n85 = Not Equal To 0?(x=w524) -> (x != 0?=w520:bool)
                      n86 = Select(t=w522, s=w520, f=w523) -> (s? t:f=w521:u16[])
                    }
                  }
                }
                frame "UploadSettings_Read_dataMTrig" {
                  n87 = call "BRig_RT__Case_Idle__State_UploadSettings_checkFile.vi"("input_dataName"="MTrig") -> ("output_Iexist"=w528:bool, "output_dataPath"=w529:path)  [unwired: 9 in]
                  n88 = case shown="True" w528 {
                    tunnel: w529 -> [_ w537]
                    tunnel: w527 -> [w535 w541]
                    tunnel: [w535 w539] -> w530
                    frame False {
                    }
                    frame True {
                      n89 = call-poly <vilib>:"Read From Spreadsheet File.vi"("delimiter (\\t)"="," ("delimiter (\\t)"), "file path (dialog if empty)"=w537) -> ("first row"=w536:i64[])  [unwired: 5 in, 4 out]
                      n90 = Array Size(array=w536) -> (size(s)=w542:i32)
                      n91 = To Unsigned Word Integer(number=w536) -> (unsigned 16bit integer=w540:u16[])
                      n92 = flat-sequence {
                        tunnel: w537 -> [w544]
                        tunnel: w536 -> [_]
                        frame #0 {
                          n93 = Delete(path (use dialog)=w544) -> ()  [unwired: 4 in, 3 out]
                        }
                      }
                      n94 = Not Equal To 0?(x=w542) -> (x != 0?=w538:bool)
                      n95 = Select(t=w540, s=w538, f=w541) -> (s? t:f=w539:u16[])
                    }
                  }
                }
                frame "UploadSettings_post" {
                  w548 = TRUE ("input_setValues")
                  n96 = call "BRig_RT_panel_cue_v1,10.vi"("input_setValues"=w548, "input_dataExp"=w547) -> ()  [unwired: 9 in, 1 out]
                  n97 = call "BRig_RT_panel_ExpStruct_v1,13.vi"("input_setValues"=w548, "input_dataExp"=w547) -> ()  [unwired: 9 in, 1 out]
                  n98 = call "BRig_RT_panel_Laser1_v1,13.vi"("input_setValues"=w548, "input_dataExp"=w547, "input_dataLC"=w546) -> ()  [unwired: 7 in, 2 out]
                  n99 = call "BRig_RT_panel_Laser2_v1,13.vi"("input_setValues"=w548, "input_dataExp"=w547, "input_dataLC"=w546) -> ()  [unwired: 7 in, 2 out]
                  n100 = call "BRig_RT_panel_manualTriggering_v0,90.vi"("input_dataMTrig"=w545, "input_setValues"=w548) -> ()  [unwired: 10 in, 8 out]
                }
                frame "Idle" {
                  w628 = 100.0 ("y")
                  n101 = call "BRig_dataMTrig_Solenoid_T_L.vi"() -> ("output_Solenoid_T_L"=w566:i32)  [unwired: 11 in]
                  n102 = call "BRig_dataMTrig_Solenoid_T_R.vi"() -> ("output_Solenoid_T_R"=w565:i32)  [unwired: 11 in]
                  n103 = local read "FPGA_count2ms"() -> (w564:dbl)
                  n104 = call "BRig_dataExp_L_power_min_l1.vi"() -> ("output_L_power_min_l1"=w633:i32)  [unwired: 11 in]
                  n105 = call "BRig_dataExp_L_power_min_l2.vi"() -> ("output_L_power_min_l2"=w632:i32)  [unwired: 11 in]
                  n106 = call "BRig_dataExp_LED_baseline_Cue.vi"() -> ("output_LED_baseline_Cue"=w626:i32)  [unwired: 11 in]
                  n107 = call "BRig_dataExp_LED_baseline_l1.vi"() -> ("output_LED_baseline_l1"=w625:i32)  [unwired: 11 in]
                  n108 = call "BRig_dataExp_LED_baseline_l2.vi"() -> ("output_LED_baseline_l2"=w624:i32)  [unwired: 11 in]
                  n109 = call "BRig_dataExp_CueLed_Tpeak.vi"() -> ("output_CueLed_Tpeak"=w616:i32)  [unwired: 11 in]
                  n110 = call "BRig_dataExp_CueLed_freq.vi"() -> ("output_CueLed_Freq"=w615:i32)  [unwired: 11 in]
                  n111 = call "BRig_dataExp_L_Tpeak_l1.vi"() -> ("output_L_Tpeak_l1"=w608:i32)  [unwired: 11 in]
                  n112 = call "BRig_dataExp_L_freq_l1.vi"() -> ("output_L_freq_l1"=w607:i32)  [unwired: 11 in]
                  n113 = call "BRig_dataExp_L_Tshutter_l1.vi"() -> ("output_L_Tshutter_l1"=w606:i32)  [unwired: 11 in]
                  n114 = call "BRig_RT__Case_Idle__State_Idle__getAudioParam.vi"("input_dataExp"=w582, "input_dataMTrig"=w583) -> ("output_Audio_freq_R"=w578:u8, "output_Audio_amp_R"=w579:u16, "output_Audio_freq_L"=w580:u8, "output_Audio_amp_L"=w581:u16, "output_state"=w577:T1)  [unwired: 5 in]
                  n115 = call "BRig_dataExp_L_Tpeak_l2.vi"() -> ("output_L_Tpeak_l2"=w590:i32)  [unwired: 11 in]
                  n116 = call "BRig_dataExp_L_freq_l2.vi"() -> ("output_L_freq_l2"=w589:i32)  [unwired: 11 in]
                  n117 = call "BRig_dataExp_L_Tshutter_l2.vi"() -> ("output_L_Tshutter_l2"=w588:i32)  [unwired: 11 in]
                  n118 = local read "I_sendData"() -> (w576:bool)
                  n119 = Index Array(array=w582, index #1=w633, index #2=w632, index #3=w626, index #4=w625, index #5=w624, index #6=w616, index #7=w615, index #8=w608, index #9=w607, index #10=w606, index #11=w590, index #12=w589, index #13=w588, index #14=w566, index #15=w565) -> (element #1=w631:u16, element #2=w627:u16, element #3=w623:u16, element #4=w622:u16, element #5=w621:u16, element #6=w612:u16, element #7=w611:u16, element #8=w605:u16, element #9=w604:u16, element #10=w603:u16, element #11=w593:u16, element #12=w592:u16, element #13=w591:u16, element #14=w563:u16, element #15=w562:u16)
                  n120 = Select(t=myRIO_BRig_RT__Case_NonExp_stateList."SendData" ("Enum"), s=w576, f=w577) -> (s? t:f=w573:T1)
                  n121 = To Double Precision Float(number=w563) -> (double precision float=w561:dbl)
                  n122 = To Double Precision Float(number=w562) -> (double precision float=w560:dbl)
                  n123 = To Double Precision Float(number=w631) -> (double precision float=w630:dbl)
                  n124 = To Double Precision Float(number=w627) -> (double precision float=w629:dbl)
                  n125 = To Double Precision Float(number=w612) -> (double precision float=w614:dbl)
                  n126 = To Double Precision Float(number=w611) -> (double precision float=w613:dbl)
                  n127 = To Double Precision Float(number=w605) -> (double precision float=w602:dbl)
                  n128 = To Double Precision Float(number=w604) -> (double precision float=w601:dbl)
                  n129 = To Double Precision Float(number=w603) -> (double precision float=w600:dbl)
                  n130 = To Unsigned Word Integer(number=w564) -> (unsigned 16bit integer=w617:u16)
                  n131 = To Double Precision Float(number=w593) -> (double precision float=w594:dbl)
                  n132 = To Double Precision Float(number=w592) -> (double precision float=w595:dbl)
                  n133 = To Double Precision Float(number=w591) -> (double precision float=w596:dbl)
                  n134 = Not Equal To 0?(x=w621) -> (x != 0?=w618:bool)
                  n135 = Not Equal To 0?(x=w623) -> (x != 0?=w620:bool)
                  n136 = Not Equal To 0?(x=w622) -> (x != 0?=w619:bool)
                  n137 = Divide(x=w630, y=w628) -> (x/y=w557:dbl)
                  n138 = Divide(x=w629, y=w628) -> (x/y=w556:dbl)
                  n139 = local read "LaserFiber_V_l1"() -> (w552:dbl)
                  n140 = local read "LaserFiber_V_l2"() -> (w553:dbl)
                  n141 = local read "get_countPerMS"() -> (w572:bool)
                  n142 = Multiply(x=w564, y=w561) -> (x*y=w570:dbl)
                  n143 = Multiply(x=w564, y=w560) -> (x*y=w568:dbl)
                  n144 = call "BRig_RT__Case_Idle__calc_FPGA_CueLed.vi"("input_FPGA_ms2count"=w564, "input_Tpeak"=w614, "input_Freq"=w613) -> ("output_laser_Npeak"=w610:u32, "output_laser_Nvalley"=w609:u32)  [unwired: 11 in]
                  n145 = call "BRig_RT__Case_Idle__calc_FPGA_laser.vi"("input_FPGA_ms2count"=w564, "input_Tpeak"=w602, "input_Freq"=w601, "input_Tshutter"=w600) -> ("output_laser_Npeak"=w599:u32, "output_laser_Nvalley"=w598:u32, "output_laser_Nshutter"=w597:u32)  [unwired: 9 in]
                  n146 = call "BRig_RT__Case_Idle__calc_FPGA_laser.vi"("input_FPGA_ms2count"=w564, "input_Tpeak"=w594, "input_Freq"=w595, "input_Tshutter"=w596) -> ("output_laser_Npeak"=w587:u32, "output_laser_Nvalley"=w586:u32, "output_laser_Nshutter"=w585:u32)  [unwired: 9 in]
                  n147 = local write "L_Power_l1"(w557) -> ()
                  n148 = local write "L_Power_l2"(w556) -> ()
                  n149 = call "myRIO__convert__Voltage_to_FPGAvalue.vi"("input_voltage"=w557) -> ("output_PortA"=w555:u16)  [unwired: 9 in, 1 out]
                  n150 = call "myRIO__convert__Voltage_to_FPGAvalue.vi"("input_voltage"=w556) -> ("output_PortA"=w554:u16)  [unwired: 9 in, 1 out]
                  n151 = Round Toward +Infinity(x=w570) -> (ceil(x): smallest int >= x=w569:dbl)
                  n152 = Round Toward +Infinity(x=w568) -> (ceil(x): smallest int >= x=w567:dbl)
                  n153 = To Unsigned Long Integer(number=w569) -> (unsigned 32bit integer=w559:u32)
                  n154 = To Unsigned Long Integer(number=w567) -> (unsigned 32bit integer=w558:u32)
                  n155 = Select(t=myRIO_BRig_RT__Case_NonExp_stateList."Get_FPGA_count_per_ms" ("Enum"), s=w572, f=w573) -> (s? t:f=w571:T1)
                  n156 = call "myRIO__convert__Voltage_to_FPGAvalue.vi"("input_voltage"=w552) -> ("output_PortA"=w551:u16)  [unwired: 9 in, 1 out]
                  n157 = call "myRIO__convert__Voltage_to_FPGAvalue.vi"("input_voltage"=w553) -> ("output_PortA"=w550:u16)  [unwired: 9 in, 1 out]
                  n158 = xnode "Read/Write Control"("FPGA VI Reference In"=w636, "error in"=w635, "audioAmp_L"=w581, "audioFreq_L_kHz"=w580, "audioAmp_R"=w579, "audioFreq_R_kHz"=w578, "AnaOut_0"=w555, "AnaOut_1"=w554, "CueLed_Baseline"=w620, "L1Led_Baseline"=w619, "L2Led_Baseline"=w618, "k1__counter_per_ms"=w617, "CueLed_nPeak"=w610, "CueLed_nValley"=w609, "LC_nPeak_l1"=w599, "LC_nValley_l1"=w598, "LC_nShutter_l1"=w597, "LC_nPeak_l2"=w587, "LC_nValley_l2"=w586, "LC_nShutter_l2"=w585, "Solenoid_nTotal_L"=w559, "Solenoid_nTotal_R"=w558, "AnaOut0_Pair"=w551, "AnaOut1_Pair"=w550) -> ("error out"=w634:errorcluster)  [unwired: 1 out]
                  n159 = local write "error out"(w634) -> ()
                }
                frame "Idle_2" {
                  w646 = FALSE
                  n160 = call "BRig_RT_panel_cue_v1,10.vi"("input_setValues"=w646, "input_dataExp"=w640) -> ("output_dataExp"=w639:u16[])  [unwired: 9 in]
                  n161 = call "BRig_RT_panel_ExpStruct_v1,13.vi"("input_setValues"=w646, "input_dataExp"=w639) -> ("output_dataExp"=w638:u16[])  [unwired: 9 in]
                  n162 = local read "comm_TCP_connect"() -> (w645:bool)
                  n163 = call "BRig_RT_panel_Laser1_v1,13.vi"("input_setValues"=w646, "input_dataExp"=w638, "input_dataLC"=w652) -> ("output_dataExp"=w647:u16[], "output_dataLC"=w649:u16[])  [unwired: 7 in]
                  n164 = Select(t=myRIO_BRig_RT__Case_NonExp_stateList."commTCP_connect" ("Enum"), s=w645, f=myRIO_BRig_RT__Case_NonExp_stateList."Idle_6" ("Enum")) -> (s? t:f=w643:T1)
                  n165 = call "BRig_RT_panel_Laser2_v1,13.vi"("input_setValues"=w646, "input_dataExp"=w647, "input_dataLC"=w649) -> ("output_dataExp"=w637:u16[], "output_dataLC"=w648:u16[])  [unwired: 7 in]
                  n166 = local read "comm_WebDAV_connect"() -> (w644:bool)
                  n167 = Select(t=myRIO_BRig_RT__Case_NonExp_stateList."TestConnection" ("Enum"), s=w644, f=w643) -> (s? t:f=w641:T1)
                }
                frame "Idle_6" {
                  n168 = local read "lick_Rising(F)_or_Falling(T)"() -> (w654:bool)
                  n169 = call "BRig_RT__Case_Idle__State_UploadSettings_checkFile.vi"("input_dataName"="dataExp") -> ("output_Iexist"=w663:bool)  [unwired: 9 in, 1 out]
                  n170 = xnode "Read/Write Control"("FPGA VI Reference In"=w656, "error in"=w655, "Rising(F)_or_Falling(T)"=w654) -> ()  [unwired: 2 out]
                  n171 = Select(t=myRIO_BRig_RT__Case_NonExp_stateList."UploadSettings_pre" ("Enum"), s=w663, f=myRIO_BRig_RT__Case_NonExp_stateList."Idle") -> (s? t:f=w661:T1)
                }
                frame "Cue_pre" {
                  n172 = call "BRig_RT__Case_Idle__State_Cue_pre__v2.vi"("input_dataExp"=w665, "input_dataMTrig"=w669) -> ("output_dataMTrig"=w668:u16[], "output_state"=w667:T1)  [unwired: 8 in]
                }
                frame "Cue" {
                  n173 = call "BRig_RT__Case_Idle__State_Cue__v2.vi"("input_cLick_R_prev"=w672, "input_cLick_R"=w673, "input_state"=w678, "input_cLick_L_prev"=w674, "input_cLick_L"=w675, "input_dataMTrig"=w679) -> ("output_dataMTrig"=w677:u16[], "output_state"=w676:T1)  [unwired: 4 in]
                }
                frame "RewardCalibration_pre" {
                  n174 = call "BRig_RT__Case_Idle__State_RewardCalibration_pre__v2.vi"("input_dataMTrig"=w681) -> ("output_dataMTrig"=w680:u16[])  [unwired: 26 in]
                }
                frame "RewardCalibration" {
                  n175 = call "BRig_RT__Case_Idle__State_RewardCalibration.vi"("input_state"=w686, "input_dataMTrig"=w688) -> ("output_dataMtrig"=w687:u16[], "output_state"=w685:T1)  [unwired: 8 in]
                }
                frame "TestConnection" {
                  n176 = local read "Host Password"() -> (w694:string)
                  n177 = local read "Host UserName"() -> (w695:string)
                  n178 = call "BRig_RT_comm_webdav_connect.vi"("input_password"=w694, "input_username"=w695) -> ("output_Iconnected"=w693:bool, "output_hSession"=w692:T4)  [unwired: 6 in, 2 out]
                  n179 = local write "comm_WebDAV_connect"(FALSE ("comm_WebDAV_connect")) -> ()
                  n180 = local write "comm_WebDAV"(w693) -> ()
                }
                frame "SendData" {
                  n181 = And(x=w704, y=w703) -> (x .and. y?=w702:bool)
                  n182 = case shown="True" w702 {
                    tunnel: w703 -> [_ w721]
                    tunnel: w709 -> [_ w720]
                    tunnel: w708 -> [_ w719]
                    tunnel: w706 -> [_ w717]
                    tunnel: w705 -> [_ w716]
                    frame False {
                      n183 = One Button Dialog(message="Unable to send data:\n Missing one or more\n connections") -> ()  [unwired: 1 in, 1 out]
                    }
                    frame True {
                      n184 = local read "Data Set Prefix"() -> (w722:string)
                      n185 = call "BRig_RT_comm_webdav_upload_all__v3.vi"("input_I_connected_webdav"=w721, "input_fileName_prefix"=w722, "input_hSession"=w720, "input_error"=w719, "input_True"=TRUE) -> ("output_nFilenames"=w723:i32, "output_arrFilenames"=w724:string[], "output_uploaded"=w725:bool[], "output_strCmd"=w718:string)  [unwired: 5 in, 2 out]
                      n186 = call "BRig_RT_comm_tcp_write_RTwrite.vi"("input_error"=w716, "input_packet"=w718, "input_hTCP"=w717) -> ()  [unwired: 5 in, 4 out]
                      n187 = call "BRig_RT_comm_webdav_upload_all_warnUser.vi"("input_n"=w723, "input_arrFilenames"=w724, "input_arrUploaded"=w725) -> ()  [unwired: 9 in]
                    }
                  }
                  n188 = local write "I_sendData"(FALSE ("I_sendData")) -> ()
                }
                frame "Get_FPGA_count_per_ms" {
                  # "Used to automatically determine how many FPGA cycles in 1 ms"
                  n189 = case shown="True" w738 {
                    selector: w738 -> [w740 _]
                    tunnel: w736 -> [_ w753]
                    tunnel: [w744 w753] -> w735
                    tunnel: w734 -> [w743 w751]
                    tunnel: w733 -> [w742 w750]
                    tunnel: [w741 w748] -> w728
                    tunnel: [w740 w747] -> w732
                    frame False {
                      n190 = Get Date/Time In Seconds() -> (seconds since 1Jan1904=w745:timestamp)
                      n191 = To Double Precision Float(number=w745) -> (double precision float=w744:dbl)
                      n192 = xnode "Read/Write Control"("FPGA VI Reference In"=w743, "error in"=w742, "timeTrial_trig"=TRUE ("timeTrial")) -> ("error out"=w741:errorcluster)  [unwired: 1 out]
                      n193 = local write "get_countPerMS"(w740) -> ()
                    }
                    frame True {
                      w749 = 1.0
                      n194 = Get Date/Time In Seconds() -> (seconds since 1Jan1904=w754:timestamp)
                      n195 = To Double Precision Float(number=w754) -> (double precision float=w755:dbl)
                      n196 = Subtract(x=w755, y=w753) -> (x-y=w752:dbl)
                      n197 = Less Or Equal?(x=w749, y=w752) -> (x <= y?=w747:bool)
                      n198 = case shown="True" w747 {
                        tunnel: w751 -> [_ w768]
                        tunnel: w750 -> [w756 w767]
                        tunnel: w749 -> [_ w758]
                        tunnel: [w756 w757] -> w748
                        frame False {
                        }
                        frame True {
                          n199 = xnode "Read/Write Control"("FPGA VI Reference In"=w768, "error in"=w767) -> ("FPGA VI Reference Out"=w765:refnum<k20>, "error out"=w764:errorcluster, "timeTrial_count"=w759:u32)
                          n200 = Multiply(x=w758, y=1000.0) -> (x*y=w762:dbl)
                          n201 = To Double Precision Float(number=w759) -> (double precision float=w761:dbl)
                          n202 = Divide(x=w761, y=w762) -> (x/y=w763:dbl)
                          n203 = local write "FPGA_count2ms"(w763) -> ()
                          n204 = xnode "Read/Write Control"("FPGA VI Reference In"=w765, "error in"=w764, "timeTrial_trig"=FALSE ("timeTrial")) -> ("error out"=w757:errorcluster)  [unwired: 1 out]
                        }
                      }
                    }
                  }
                  n205 = Select(t=myRIO_BRig_RT__Case_NonExp_stateList."Idle" ("Enum"), s=w732, f=w730) -> (s? t:f=w729:T1)
                  n206 = local write "error out"(w728) -> ()
                }
                frame "End" {
                }
                frame "commTCP_connect" {
                  n207 = local read "comm_TCP_connect"() -> (w778:bool)
                  n208 = case shown="True" w785 {
                    tunnel: w784 -> [w795 w804]
                    tunnel: [w794 w800] -> w782
                    tunnel: [w793 w797] -> w774
                    tunnel: [w792 w798] -> w783
                    tunnel: w781 -> [_ w805]
                    frame False {
                      n209 = call "BRig_RT_comm_tcp_connect_RTwrite.vi"("input_error"=w795) -> ("output_error"=w792:errorcluster, "output_connected"=w793:bool, "output_hTCP"=w794:refnum<k5>)  [unwired: 8 in]
                    }
                    frame True {
                      n210 = call "BRig_RT_comm_tcp_write_RTwrite.vi"("input_error"=w804, "input_packet"="<test>", "input_hTCP"=w805) -> ("output_error"=w799:errorcluster, "output_I_NotDisconnected"=w796:bool, "output_I_write"=w802:bool, "output_hTCP"=w801:refnum<k5>)  [unwired: 5 in]
                      n211 = case shown="False" w802 {
                        selector: w802 -> [_ w816]
                        tunnel: w801 -> [w811 w818]
                        tunnel: [w806 w818] -> w800
                        tunnel: w799 -> [w810 w817]
                        tunnel: [w808 w817] -> w798
                        tunnel: [w807 w816] -> w797
                        tunnel: w796 -> [w812 _]
                        frame False {
                          n212 = case shown="True" w812 {
                            tunnel: w811 -> [_ w815]
                            tunnel: w810 -> [w813 w814]
                            tunnel: [w813 w814] -> w809
                            frame False {
                            }
                            frame True {
                              n213 = TCP Close Connection(connection ID=w815, error in (no error)=w814) -> ()  [unwired: 1 in, 2 out]
                            }
                          }
                          n214 = call "BRig_RT_comm_tcp_connect_RTwrite.vi"("input_error"=w809) -> ("output_error"=w808:errorcluster, "output_connected"=w807:bool, "output_hTCP"=w806:refnum<k5>)  [unwired: 8 in]
                        }
                        frame True {
                        }
                      }
                    }
                  }
                  n215 = Not(x=w778) -> (.not. x?=w777:bool)
                  n216 = Or(x=w777, y=w774) -> (x .or. y?=w776:bool)
                  n217 = case shown="True" w776 {
                    tunnel: [w789 myRIO_BRig_RT__Case_NonExp_stateList."Idle" ("Enum")] -> w780
                    tunnel: w779 -> [w789 _]
                    frame False {
                    }
                    frame True {
                      n218 = local write "comm_TCP_connect"(FALSE) -> ()
                    }
                  }
                  n219 = local write "comm_TCP"(w774) -> ()
                }
              }
              n220 = case shown="True" w397 {
                tunnel: [w455 w456] -> w400
                tunnel: [w454 w457] -> w399
                tunnel: [w453 w458] -> w398
                tunnel: w396 -> [w455 _]
                tunnel: w395 -> [w454 _]
                tunnel: w394 -> [w453 _]
                tunnel: w393 -> [_ w458]
                tunnel: w392 -> [_ w457]
                tunnel: w391 -> [_ w456]
                frame False {
                }
                frame True {
                }
              }
              n221 = case shown="True" w387 {
                tunnel: [w449 w450] -> w386
                tunnel: [w448 w451] -> w385
                tunnel: [w447 w452] -> w384
                tunnel: w388 -> [w449 _]
                tunnel: w389 -> [w448 _]
                tunnel: w390 -> [w447 _]
                tunnel: w382 -> [_ w452]
                tunnel: w381 -> [_ w451]
                tunnel: w383 -> [_ w450]
                frame False {
                }
                frame True {
                }
              }
              n222 = flat-sequence {
                tunnel: w420 -> [w462]
                tunnel: w418 -> [w460]
                tunnel: [w462] -> w424
                tunnel: [w461] -> w423
                tunnel: [w460] -> w422
                tunnel: [w459] -> w421
                tunnel: w417 -> [w459]
                tunnel: [w474] -> w419
                tunnel: w424 -> [w474]
                tunnel: w423 -> [w473]
                tunnel: w422 -> [w471]
                tunnel: w421 -> [w466]
                tunnel: [w465] -> w416
                frame #0 {
                  n223 = Get Date/Time In Seconds() -> (seconds since 1Jan1904=w461:timestamp)
                }
                frame #1 {
                  # "threshold"
                  # "delta T [ms]"
                  # "delta T [s]"
                  n224 = To Double Precision Float(number=w473) -> (double precision float=w472:dbl)
                  n225 = To Double Precision Float(number=w471) -> (double precision float=w470:dbl)
                  n226 = Subtract(x=w472, y=w470) -> (x-y=w469:dbl)
                  n227 = Multiply(x=w469, y=1000.0) -> (x*y=w464:dbl)
                  n228 = Greater?(x=w464, y=5.0) -> (0:w463:bool)
                  n229 = local write "Threshold"(w463) -> ()
                  n230 = local write "tLoop"(w464) -> ()
                  n231 = Or(x=w463, y=w466) -> (x .or. y?=w465:bool)
                }
              }
              n232 = local read "START"() -> (w441:bool)
              n233 = local read "STOP_abort"() -> (w440:bool)
              n234 = local read "Laser1_LED"() -> (w378:bool)
              n235 = local read "Laser2_LED"() -> (w377:bool)
              n236 = call "BRig_RT_panel_manualTriggering_v0,90.vi"("input_dataMTrig"=w405) -> ("output_Solenoid_R"=w408:bool, "output_Solenoid_L"=w409:bool, "output_dataMTrig"=w415:u16[], "output_Audio_L"=w410:bool, "output_Audio_R"=w411:bool, "output_CueLed"=w412:bool, "output_Laser_l1"=w413:bool, "output_Laser_l2"=w414:bool)  [unwired: 11 in]
              n237 = Or(x=w441, y=w440) -> (x .or. y?=w439:bool)
              n238 = Select(t=myRIO_BRig_RT__Case_NonExp_stateList."End" ("Enum"), s=w439, f=w438) -> (s? t:f=w437:T1)
              n239 = xnode "Read/Write Control"("FPGA VI Reference In"=w432, "error in"=w431, "A1_SR"=w408, "A3_SL"=w409, "audioTrigger_L"=w410, "audioTrigger_R"=w411, "LC_Laser_l1"=w413, "LC_Laser_l2"=w414, "CueLed_Event"=w412, "L1Led_ON"=w378, "L2Led_ON"=w377) -> ("FPGA VI Reference Out"=w443:refnum<k20>, "error out"=w420:errorcluster, "fpga_laser1"=w373:bool, "fpga_laser2"=w374:bool, "fpga_solenoid_L"=w375:bool, "fpga_solenoid_R"=w376:bool)
              n240 = local write "Laser1"(w373) -> ()
              n241 = local write "Laser2"(w374) -> ()
              n242 = local write "Solenoid L"(w375) -> ()
              n243 = local write "Solenoid R"(w376) -> ()
              n244 = node-c288() -> ()  [unwired: 1 in, 1 out]
            }
            n245 = node-c288(w368) -> ()  [unwired: 1 out]
            n246 = flat-sequence {
              tunnel: w362 -> [w372]
              tunnel: [w372] -> w361
              tunnel: w360 -> [w371]
              tunnel: [w371] -> w359
              frame #0 {
                w370 = FALSE
                n247 = local write "STOP_endBlock"(w370) -> ()
                n248 = local write "STOP_endTrial"(w370) -> ()
              }
            }
          }
          frame True {
            w888 = ".csv" ("string")
            w918 = ""
            w927 = u8 0
            w928 = u16 0 ("AudioLeft_phase_inc")
            w929 = FALSE
            # "buffer_dataRT_stats"
            # "Clear local files"
            # "empty array"
            # "buffer_dataBlock"
            # "buffer_dataTrial"
            # "nColumns dataBlock"
            # "nColumns dataTrial"
            # "buffer_dataBlock"
            # "buffer_dataTrial"
            # "nColumns\ndataBlock"
            # "nColumns\ndataTrial"
            # "original dataExp and dataLC"
            # "dataLick"
            # "dataTrial"
            # "dataBlock"
            # "dataCurrent"
            # "arrTrig"
            # "time stamp"
            # "dummyState counter"
            # "dataTrial"
            # "dataLick"
            # "dataLC"
            # "dataLC"
            # "dataBlock"
            # "dataMTrig"
            # "dataMTrig"
            # "dataExp"
            # "dataExp"
            # "dataCurrent"
            # "state"
            n249 = flat-sequence {
              tunnel: [w1025] -> w858
              tunnel: [w1024] -> w862
              tunnel: [w1033] -> w876
              tunnel: [w1032] -> w875
              tunnel: [myRIO_BRig_RT__Case_Exp_stateList."Start1" ("Enum")] -> w874
              tunnel: [w1030] -> w873
              tunnel: [u16 0] -> w872
              tunnel: [w1028] -> w871
              tunnel: [w1027] -> w870
              tunnel: [w1026] -> w869
              tunnel: [w1035] -> w884
              tunnel: [w1036] -> w885
              tunnel: [w1037] -> w935
              tunnel: [w1038] -> w937
              tunnel: [w1039] -> w938
              tunnel: [w1040] -> w939
              tunnel: [w1041] -> w940
              tunnel: [w1042] -> w941
              tunnel: w876 -> [w1042]
              tunnel: w875 -> [w1041]
              tunnel: w874 -> [w1040]
              tunnel: w873 -> [w1039]
              tunnel: w872 -> [w1038]
              tunnel: w871 -> [w1037]
              tunnel: w870 -> [w1036]
              tunnel: w869 -> [w1035]
              tunnel: [w1034] -> w867
              frame #0 {
                n250 = call "BRig_dataBlock_init.vi"() -> ("output_nCol"=w1024:i32, "output_dataBlock"=w1026:u16[][])  [unwired: 10 in]
                n251 = call "BRig_dataCurrent_init.vi"() -> ("output_dataCurrent"=w1033:u16[])  [unwired: 11 in]
                n252 = call "BRig_dataLick_init.vi"() -> ("output_dataLick"=w1032:u16[][])  [unwired: 11 in]
                n253 = call "BRig_dataTrial_init.vi"() -> ("output_nCol"=w1025:i32, "output_dataTrial"=w1027:u16[][])  [unwired: 10 in]
                n254 = Get Date/Time In Seconds() -> (seconds since 1Jan1904=w1023:timestamp)
                n255 = To Double Precision Float(number=w1023) -> (double precision float=w1030:dbl)
                n256 = call "BRig_arrTrig_init.vi"() -> ("output_arrTrig"=w1028:bool[])  [unwired: 11 in]
              }
              frame #1 {
                w1034 = u32 2 ("milliseconds to wait")
                n257 = Wait (ms)(milliseconds to wait=w1034) -> ()  [unwired: 1 out]
              }
            }
            n258 = flat-sequence {
              tunnel: w864 -> [w1004]
              tunnel: [w1004] -> w863
              tunnel: w863 -> [w1013]
              tunnel: [w1011] -> w846
              tunnel: [w1010] -> w833
              tunnel: [w1007] -> w861
              tunnel: w862 -> [w1006]
              tunnel: w858 -> [w1005]
              tunnel: [w1013] -> w860
              tunnel: w860 -> [w1015]
              tunnel: [w1015] -> w859
              tunnel: w859 -> [w1021]
              tunnel: w858 -> [w1020]
              tunnel: [w1018] -> w853
              tunnel: [w1016] -> w856
              tunnel: [w1021] -> w857
              tunnel: [w1022] -> _
              tunnel: w857 -> [w1022]
              frame #0 {
                n259 = Wait (ms)(milliseconds to wait=w1004) -> ()  [unwired: 1 out]
              }
              frame #1 {
                w1008 = u16 0 ("element")
                n260 = Initialize Array(w1008, 8 ("dimension size")) -> (w1011:u16[])
                n261 = Initialize Array(w1008, 100 ("dimension size"), w1005) -> (w1010:u16[][])
                n262 = Initialize Array(w1008, 10 ("dimension size"), w1006) -> (w1007:u16[][])
              }
              frame #2 {
                n263 = Wait (ms)(milliseconds to wait=w1015) -> ()  [unwired: 1 out]
              }
              frame #3 {
                n264 = Increment(x=w1020) -> (x+1=w1017:i32)
                n265 = To Unsigned Long Integer(number=w1017) -> (unsigned 32bit integer=w1016:u32)
                n266 = Initialize Array(u16 0 ("element"), w1017) -> (w1018:u16[])
              }
              frame #4 {
                n267 = Wait (ms)(milliseconds to wait=w1022) -> ()  [unwired: 1 out]
              }
            }
            n268 = call "BRig_comm_webdav_myrioFolder.vi"() -> ("output_myrioFolder"=w889:string)  [unwired: 11 in]
            n269 = local write "stop_TimedLoop"(FALSE ("stop_TimedLoop")) -> ()
            n270 = RT FIFO Create(0:"dataTrialOrBlock" ("name (unnamed)"), 1:w853, 4:u32 40 ("size (10)"), 6:w856, 7:T8 {"read mode"=enum."blocking", "write mode"=enum."blocking"} ("r/w modes (polling,polling)")) -> (8:w855:refnum<k33>, 11:w854:errorcluster)  [unwired: 3 in, 1 out]
            n271 = RT FIFO Create(0:"dataAnalog" ("name (unnamed)"), 1:u16 0 ("element"), 4:u32 1000 ("size (10)")) -> (8:w841:refnum<k33>, 11:w840:errorcluster)  [unwired: 5 in, 1 out]
            n272 = Concatenate Strings(w889, "dataTrial" ("input_filename"), w888) -> (w890:string)
            n273 = Concatenate Strings(w889, "dataBlock" ("input_filename"), w888) -> (w891:string)
            n274 = String To Path(string=w890) -> (path=w894:path)
            n275 = String To Path(string=w891) -> (path=w886:path)
            n276 = flat-sequence {
              tunnel: [w1043] -> w868
              tunnel: w867 -> [w1043]
              tunnel: w868 -> [w1044]
              tunnel: [w1044] -> w865
              tunnel: w881 -> [w1047]
              tunnel: w834 -> [w1046]
              tunnel: [w1045] -> w866
              tunnel: w865 -> [w1045]
              tunnel: [w1051] -> _
              tunnel: w880 -> [w1051]
              tunnel: w879 -> [w1050]
              tunnel: w878 -> [w1049]
              tunnel: [w1048] -> w864
              tunnel: w866 -> [w1048]
              frame #0 {
                n277 = call "BRig_RT__Case_Exp__clearLocalFolder.vi"() -> ()  [unwired: 12 in]
              }
              frame #1 {
                n278 = Wait (ms)(milliseconds to wait=w1044) -> ()  [unwired: 1 out]
              }
              frame #2 {
                n279 = call "BRig_RT__Case_Exp__State_start__sendExpData_saveData.vi"("input_dataLC"=w1047, "input_dataExp"=w1046) -> ()  [unwired: 10 in]
              }
              frame #3 {
                n280 = call "BRig_RT__Case_Exp__State_start__sendExpData_uploadData__v2.vi"("input_error"=w1051, "input_hSession"=w1050, "input_connected"=w1049) -> ()  [unwired: 8 in, 1 out]
              }
            }
            n281 = call "BRig_RT__Case_Exp__comm_tcp__data_other.vi"("input_strState"=w918, "input_strAccum"=w918, "input_error"=w923, "input_hTCP"=w924, "input_I_connected_TCP"=w925) -> ("output_strAccum"=w919:string, "output_error"=w920:errorcluster, "output_hTCP"=w921:refnum<k5>, "output_I_connect_TCP"=w922:bool)  [unwired: 3 in]
            n282 = Initialize Array(u16 0 ("element"), 60 ("dimension size")) -> (w828:u16[])
            n283 = node-c288() -> (w947:T5)  [unwired: 4 in]
            n284 = timed-loop {
              timing: w947 -> [_]
              timing-out: [_] -> w946
              shift-right: [w1337] -> _
              shift-left: w939 -> [w1292]
              tunnel: w934 -> [w1381]
              tunnel: w933 -> [w1361]
              shift-right: [w1325] -> _
              shift-left: w945 -> [w1380]
              shift-right: [w1324] -> _
              shift-left: w944 -> [w1379]
              tunnel: [w1372] -> w926
              tunnel: [w1373] -> w943
              shift-right: [w1335] -> w914
              shift-left: w941 -> [w1309]
              shift-right: [w1378] -> w915
              shift-left: w834 -> [w1311]
              shift-right: [w1355] -> w917
              shift-left: w931 -> [w1312]
              shift-right: [w1376] -> _
              shift-left: w884 -> [w1377]
              shift-right: [w1374] -> w916
              shift-left: w881 -> [w1375]
              shift-right: [w1331] -> w913
              shift-left: w940 -> [w1338]
              shift-right: [w1371] -> _
              shift-left: w885 -> [w1310]
              tunnel: w938 -> [w1370]
              shift-right: [w1344] -> _
              shift-left: u16 0 -> [w1343]
              shift-right: [w1364] -> _
              shift-left: w937 -> [w1365]
              shift-right: [w1362] -> _
              shift-left: w935 -> [w1363]
              shift-right: [w1356] -> _
              shift-left: FALSE -> [w1358]
              shift-right: [w1300] -> w905
              shift-left: w922 -> [w1319]
              shift-right: [w1299] -> w904
              shift-left: w921 -> [w1318]
              shift-right: [w1297] -> w903
              shift-left: w920 -> [w1317]
              shift-right: [w1298] -> _
              shift-left: w919 -> [w1316]
              shift-right: [w1306] -> w910
              shift-left: w880 -> [w1306]
              shift-right: [w1308] -> w908
              shift-left: w878 -> [w1308]
              shift-right: [w1307] -> w909
              shift-left: w879 -> [w1307]
              shift-right: [w1305] -> _
              shift-left: _ -> [w1303]
              shift-right: [w1304] -> _
              shift-left: _ -> [w1302]
              tunnel: [w1301] -> w897
              tunnel: w855 -> [w1295]
              tunnel: w854 -> [w1294]
              tunnel: w853 -> [w1293]
              tunnel: w841 -> [w1291]
              tunnel: w840 -> [w1290]
              tunnel: w834 -> [w1289]
              stop <- w1301 stop-if-true
              # "iOccurrence"
              # "index"
              # "resetOccurrence?\ndataAnalog"
              # "dataLick"
              # "dataLick"
              # "dummyState counter"
              # "dummyState counter"
              # "iOccurrence"
              # "arrTrig"
              # "arrTrig"
              # "CueLed"
              # "LC_Laser_l2"
              # "LC_Event_l2"
              # "LC_Laser_l1"
              # "LC_Event_l1"
              # "iState"
              # "dataAnalog"
              # "index"
              # "manual triggering"
              # "dataTrial"
              # "dataBlock"
              # "dataExp"
              # "dataCurrent"
              # "time stamp"
              # "audio__L\naudio__R"
              # "dataLC"
              # "solenoid__R"
              # "solenoid__L"
              # "Did a lick occur?"
              # "Update lick counter"
              # "state"
              # "state"
              n285 = node-c288() -> ()  [unwired: 1 in, 1 out]
              n286 = local write "cState"(w1292) -> ()
              n287 = flat-sequence {
                tunnel: w1361 -> [w1382]
                tunnel: [w1383] -> w1359
                tunnel: [w1382] -> w1360
                frame #0 {
                  n288 = Get Date/Time In Seconds() -> (seconds since 1Jan1904=w1383:timestamp)
                }
              }
              n289 = xnode "Read/Write Control"("FPGA VI Reference In"=w1381, "error in"=w1360) -> ("FPGA VI Reference Out"=w1367:refnum<k20>, "error out"=w1366:errorcluster, "A2_LickL"=w1325:u32, "A4_LickR"=w1324:u32)
              n290 = local write "A2"(w1325) -> ()
              n291 = local write "A4"(w1324) -> ()
              n292 = Greater?(x=w1325, y=w1380) -> (0:w1333:bool)
              n293 = Greater?(x=w1324, y=w1379) -> (0:w1332:bool)
              n294 = Or(x=w1333, y=w1332) -> (x .or. y?=w1334:bool)
              n295 = case shown="\"setSettings_Laser\"" w1292 {
                selector: w1292 -> [_ _ _ _ _ _ _ _ _ _ _ _ _ _ w1691 w1707 _ w1736 _ _ w1783 w1810 _ w1836 _ w1880 _ w1962 _ w1982 _ _ w2134 w2144 _ _ _ _ w2262 _ w2286 w2317 w2338 w2363 _ w2428 w2438 _]
                tunnel: [myRIO_BRig_RT__Case_Exp_stateList."Start2" ("Enum") myRIO_BRig_RT__Case_Exp_stateList."Start3" ("Enum") myRIO_BRig_RT__Case_Exp_stateList."saveSettings1" ("Enum") myRIO_BRig_RT__Case_Exp_stateList."initBlock" ("Enum") myRIO_BRig_RT__Case_Exp_stateList."initTrial_LC_ENL1" ("Enum") myRIO_BRig_RT__Case_Exp_stateList."initTrial" ("Enum") myRIO_BRig_RT__Case_Exp_stateList."initTrial2" ("Enum") myRIO_BRig_RT__Case_Exp_stateList."setSettings_Laser" ("Enum") myRIO_BRig_RT__Case_Exp_stateList."ENL1_pre" ("Enum") myRIO_BRig_RT__Case_Exp_stateList."initTrial_LC_Cue1" ("Enum") myRIO_BRig_RT__Case_Exp_stateList."initTrial_LC_Sel" ("Enum") myRIO_BRig_RT__Case_Exp_stateList."initTrial4" ("Enum") w1669 w1681 w1689 w1705 myRIO_BRig_RT__Case_Exp_stateList."ENL1Penalty" ("Enum") w1734 w1749 w1761 w1782 w1809 myRIO_BRig_RT__Case_Exp_stateList."Cue1Penalty" ("Enum") w1837 w1853 w1875 myRIO_BRig_RT__Case_Exp_stateList."SelectReward" ("Enum") w1961 myRIO_BRig_RT__Case_Exp_stateList."SelectRewardPost" ("Enum") w1981 myRIO_BRig_RT__Case_Exp_stateList."SelectWrong" ("Enum") myRIO_BRig_RT__Case_Exp_stateList."SelectTimeout" ("Enum") w2133 w2143 myRIO_BRig_RT__Case_Exp_stateList."saveData_dataTrial" ("Enum") w2178 w2213 w2251 w2262 myRIO_BRig_RT__Case_Exp_stateList."initBlock" ("Enum") w2284 w2318 w2337 w2362 myRIO_BRig_RT__Case_Exp_stateList."FreeReward" ("Enum") w2426 w2436 myRIO_BRig_RT__Case_Exp_stateList."FreeRewardPost" ("Enum")] -> w1337
                tunnel: w1334 -> [_ _ _ _ _ _ _ _ _ _ _ _ w1670 w1682 w1690 w1706 _ _ w1750 w1762 w1784 w1811 _ _ _ _ _ _ _ _ _ _ _ _ _ _ _ _ _ _ _ _ _ _ _ _ _ _]
                tunnel: w1333 -> [_ _ _ _ _ _ _ _ _ _ _ _ _ _ _ _ _ _ _ _ _ _ _ _ w1846 w1876 _ _ _ _ _ _ _ _ _ _ _ _ _ _ _ _ _ _ _ _ _ _]
                tunnel: w1332 -> [_ _ _ _ _ _ _ _ _ _ _ _ _ _ _ _ _ _ _ _ _ _ _ _ w1845 w1877 _ _ _ _ _ _ _ _ _ _ _ _ _ _ _ _ _ _ _ _ _ _]
                tunnel: w1309 -> [w1393 w1399 w1441 w1468 w1493 w1547 w1561 w1576 w1604 w1629 w1639 w1656 w1668 w1680 w1698 w1714 w1725 w1733 w1751 w1763 w1785 w1812 w1829 w1835 w1856 w1873 w1915 w1958 w1972 w1980 w2010 w2081 w2132 w2142 w2158 w2184 w2222 w2241 w2261 w2268 w2287 w2320 w2336 w2353 w2398 w2424 w2435 w2446]
                tunnel: w1311 -> [w1384 w1398 w1431 w1466 w1481 w1546 w1549 w1575 w1598 w1628 w1638 w1648 w1662 w1676 w1701 w1717 w1724 w1741 w1748 w1760 w1788 w1815 w1822 w1843 w1844 w1872 w1897 w1960 w1970 w1987 w1993 w2064 w2139 w2149 w2150 w2176 w2220 w2224 w2252 w2265 w2289 w2322 w2348 w2368 w2381 w2429 w2439 w2445]
                tunnel: [w1393 w1399 w1441 w1468 w1493 w1545 w1560 w1578 w1604 w1632 w1646 w1655 w1671 w1683 w1697 w1713 w1726 w1732 w1745 w1757 w1768 w1795 w1828 w1834 w1852 w1874 w1912 w1963 w1971 w1978 w2004 w2075 w2130 w2141 w2160 w2184 w2222 w2241 w2261 w2268 w2287 w2320 w2336 w2353 w2404 w2425 w2434 w2444] -> w1336
                tunnel: [w1384 w1398 w1430 w1466 w1481 w1546 w1549 w1575 w1598 w1628 w1638 w1648 w1662 w1676 w1701 w1717 w1724 w1741 w1748 w1760 w1788 w1815 w1822 w1843 w1844 w1872 w1897 w1960 w1970 w1987 w1993 w2064 w2139 w2149 w2150 w2173 w2220 w2227 w2252 w2265 w2289 w2322 w2348 w2368 w2382 w2429 w2439 w2445] -> w1378
                tunnel: [_ _ _ _ _ _ _ _ _ _ _ _ _ _ _ _ _ _ _ _ _ _ _ _ _ _ _ w1952 _ _ _ _ _ _ _ _ _ _ _ _ _ _ _ _ _ w2418 _ _] -> w1321
                tunnel: [_ _ _ _ _ _ _ _ _ _ _ _ _ _ _ _ _ _ _ _ _ _ _ _ _ _ _ w1951 _ _ _ _ _ _ _ _ _ _ _ _ _ _ _ _ _ w2419 _ _] -> w1320
                tunnel: w1377 -> [w1392 w1396 w1439 w1470 w1506 w1543 w1565 w1590 w1615 w1634 w1645 w1653 w1673 w1685 w1700 w1716 w1721 w1739 w1753 w1765 w1787 w1814 w1827 w1840 w1862 w1884 w1914 w1965 w1976 w1985 w2008 w2079 w2137 w2148 w2154 w2185 w2211 w2243 w2259 w2267 w2269 w2323 w2346 w2366 w2407 w2431 w2441 w2453]
                tunnel: [w1392 w1396 w1439 w1470 w1506 w1542 w1564 w1590 w1615 w1634 w1645 w1653 w1673 w1685 w1700 w1716 w1721 w1739 w1753 w1765 w1787 w1814 w1827 w1840 w1862 w1884 w1913 w1965 w1976 w1985 w2007 w2078 w2137 w2148 w2154 w2185 w2211 w2243 w2259 w2267 w2269 w2323 w2346 w2366 w2407 w2431 w2441 w2453] -> w1376
                tunnel: w1375 -> [w1385 w1397 w1440 w1469 w1501 w1548 w1572 w1591 w1616 w1633 w1640 w1654 w1672 w1684 w1699 w1715 w1722 w1740 w1752 w1764 w1786 w1813 w1826 w1842 w1861 w1885 w1886 w1964 w1967 w1986 w1988 w2059 w2138 w2147 w2167 w2175 w2223 w2245 w2260 w2264 w2288 w2321 w2347 w2367 w2408 w2432 w2442 w2454]
                tunnel: [w1385 w1397 w1440 w1469 w1501 w1548 w1572 w1591 w1616 w1633 w1640 w1654 w1672 w1684 w1699 w1715 w1722 w1740 w1752 w1764 w1786 w1813 w1826 w1842 w1861 w1885 w1886 w1964 w1967 w1986 w1988 w2059 w2138 w2147 w2167 w2174 w2223 w2245 w2260 w2264 w2288 w2321 w2347 w2367 w2408 w2432 w2442 w2454] -> w1374
                tunnel: [_ _ _ _ _ _ _ _ _ _ _ _ _ _ _ _ _ _ _ _ _ _ _ _ _ _ _ _ _ _ _ _ _ _ _ _ _ _ TRUE _ _ _ _ _ _ _ _ _] -> w1339
                tunnel: [_ _ _ _ _ _ _ _ _ _ _ _ _ _ _ _ _ _ _ _ w1770 w1797 _ _ _ _ _ _ _ _ _ _ _ _ _ _ _ _ _ _ _ _ _ _ _ _ _ _] -> w1369
                tunnel: [_ _ _ _ _ _ _ _ _ _ _ _ _ _ _ _ _ _ _ _ w1769 w1796 _ _ _ _ _ _ _ _ _ _ _ _ _ _ _ _ _ _ _ _ _ _ _ _ _ _] -> w1368
                tunnel: w1310 -> [w1390 w1395 w1437 w1467 w1505 w1541 w1568 w1592 w1608 w1635 w1644 w1652 w1667 w1679 w1688 w1704 w1718 w1738 w1747 w1759 w1773 w1800 w1824 w1839 w1860 w1864 w1909 w1959 w1966 w1984 w2006 w2077 w2136 w2146 w2166 w2183 w2221 w2242 w2257 w2266 w2273 w2300 w2345 w2365 w2402 w2430 w2440 w2452]
                tunnel: [w1390 w1395 w1437 w1467 w1505 w1540 w1563 w1577 w1602 w1631 w1643 w1651 w1666 w1678 w1687 w1703 w1718 w1738 w1746 w1758 w1772 w1799 w1824 w1839 w1860 w1863 w1908 w1959 w1966 w1984 w2003 w2074 w2136 w2146 w2165 w2183 w2221 w2242 w2257 w2266 w2273 w2300 w2345 w2365 w2402 w2430 w2440 w2452] -> w1371
                tunnel: w1370 -> [_ _ _ _ _ _ _ _ _ _ _ _ _ _ _ _ _ _ _ _ _ _ _ _ _ _ _ _ _ _ _ _ _ _ w2159 _ _ _ _ _ _ _ _ _ _ _ _ _]
                tunnel: w1367 -> [w1389 _ _ _ w1502 w1535 w1571 w1596 w1613 _ _ w1659 _ _ _ _ _ _ _ _ w1774 w1801 _ _ w1858 w1883 w1907 _ _ _ _ _ _ _ w2162 _ _ _ w2255 _ _ _ _ _ w2388 _ _ _]
                tunnel: w1366 -> [w1388 _ _ _ w1503 w1534 w1562 w1595 w1612 _ _ w1658 _ _ _ _ _ _ _ _ w1775 w1802 _ _ w1859 w1882 w1906 _ _ _ _ _ _ _ w2161 _ _ _ w2254 _ _ _ _ _ w2387 _ _ _]
                tunnel: [_ _ _ _ _ _ _ _ _ _ _ _ _ _ w1696 w1712 _ _ _ _ w1780 w1807 _ _ w1851 w1870 _ _ _ _ _ _ _ _ _ _ _ _ _ _ _ _ _ _ _ _ _ _] -> w1345
                tunnel: [_ _ _ _ _ _ _ _ _ _ _ _ _ _ w1695 w1711 _ _ _ _ w1779 w1806 _ _ w1850 w1869 _ _ _ _ _ _ _ _ _ _ _ _ _ _ _ _ _ _ _ _ _ _] -> w1326
                tunnel: [_ _ _ _ _ _ _ _ TRUE ("Recording") _ _ _ _ _ _ _ _ _ _ _ _ _ _ _ _ _ _ _ _ _ _ _ _ _ _ _ _ _ _ _ _ _ _ _ _ _ _ _] -> w1342
                tunnel: w1365 -> [_ _ _ _ _ _ _ _ _ _ _ _ _ _ _ _ _ _ _ _ _ _ _ _ _ _ _ _ _ _ _ _ _ _ _ _ _ _ _ _ w2285 w2316 w2343 w2350 _ _ _ _]
                tunnel: [_ _ _ _ _ _ _ _ _ _ _ _ _ _ _ _ _ _ _ _ _ _ _ _ _ _ _ _ _ _ _ _ _ _ _ _ _ _ _ _ w2283 w2315 w2341 w2351 _ _ _ _] -> w1364
                tunnel: w1363 -> [_ _ _ _ w1475 _ _ _ w1609 w1636 w1642 w1650 w1664 w1675 w1692 w1708 w1719 w1737 w1744 w1756 w1781 w1808 w1823 w1838 w1847 w1871 _ _ _ _ _ _ _ _ _ _ _ _ _ _ _ _ _ _ _ _ _ _]
                tunnel: [_ _ _ _ w1475 _ _ w1579 w1609 w1630 w1641 w1649 w1663 w1674 w1692 w1708 w1719 w1737 w1743 w1755 w1781 w1808 w1823 w1838 w1847 w1871 _ _ _ _ _ _ _ _ _ _ _ _ _ _ _ _ _ _ _ _ _ _] -> w1362
                tunnel: [_ _ _ _ _ _ _ _ _ _ _ _ _ _ w1694 w1710 _ _ _ _ w1778 w1805 _ _ w1849 w1868 _ _ _ _ _ _ _ _ _ _ _ _ _ _ _ _ _ _ _ _ _ _] -> w1349
                tunnel: [_ _ _ _ _ _ _ _ _ _ _ _ _ _ w1693 w1709 _ _ _ _ w1777 w1804 _ _ w1848 w1867 _ _ _ _ _ _ _ _ _ _ _ _ _ _ _ _ _ _ _ _ _ _] -> w1350
                tunnel: [_ _ _ _ _ _ _ _ _ _ _ _ _ _ _ _ _ _ _ _ w1771 w1798 _ _ _ _ _ _ _ _ _ _ _ _ _ _ _ _ _ _ _ _ _ _ _ _ _ _] -> w1352
                tunnel: [_ _ "<S,S>" ("string") _ _ _ _ _ w1603 _ _ _ _ _ _ _ _ _ _ _ _ _ _ _ _ _ w1910 _ _ _ w1995 w2066 _ _ w2157 _ _ w2237 _ _ _ _ _ _ _ _ _ _] -> w1315
                tunnel: w1312 -> [_ _ _ _ _ _ _ _ _ _ _ _ _ _ _ _ _ _ _ _ _ _ _ _ _ _ _ _ _ _ _ _ _ _ _ _ _ _ _ _ _ _ _ _ w2393 _ _ _]
                tunnel: w1308 -> [_ _ _ _ _ _ _ _ _ _ _ _ _ _ _ _ _ _ _ _ _ _ _ _ _ _ _ _ _ _ _ _ _ _ _ _ _ w2236 _ _ _ _ _ _ _ _ _ _]
                tunnel: w1307 -> [_ _ _ _ _ _ _ _ _ _ _ _ _ _ _ _ _ _ _ _ _ _ _ _ _ _ _ _ _ _ _ _ _ _ _ _ _ _ _ _ _ _ _ _ _ _ _ _]
                tunnel: w1306 -> [_ _ _ _ _ _ _ _ _ _ _ _ _ _ _ _ _ _ _ _ _ _ _ _ _ _ _ _ _ _ _ _ _ _ _ _ _ _ _ _ _ _ _ _ _ _ _ _]
                tunnel: [_ _ _ _ _ _ _ _ _ _ _ _ _ _ _ _ _ _ _ _ _ _ _ _ _ _ _ _ _ _ _ _ _ _ _ w2177 _ _ _ _ _ _ _ _ _ _ _ _] -> w1305
                tunnel: [_ _ _ _ _ _ _ _ _ _ _ _ _ _ _ _ _ _ _ _ _ _ _ _ _ _ _ _ _ _ _ _ _ _ _ w2182 _ _ _ _ _ _ _ _ _ _ _ _] -> w1304
                tunnel: w1303 -> [_ _ _ _ _ _ _ _ _ _ _ _ _ _ _ _ _ _ _ _ _ _ _ _ _ _ _ _ _ _ _ _ _ _ _ w2181 _ _ _ _ _ _ _ _ _ _ _ _]
                tunnel: w1302 -> [_ _ _ _ _ _ _ _ _ _ _ _ _ _ _ _ _ _ _ _ _ _ _ _ _ _ _ _ _ _ _ _ _ _ _ w2172 _ _ _ _ _ _ _ _ _ _ _ _]
                tunnel: w1295 -> [_ _ w1414 w1452 _ w1524 w1556 _ _ _ _ _ _ _ _ _ _ _ _ _ _ _ _ _ _ _ w1895 _ _ _ w1998 w2069 _ _ _ _ _ _ _ _ w2280 w2303 _ _ w2373 _ _ _]
                tunnel: w1294 -> [_ _ w1413 w1451 _ w1525 w1555 _ _ _ _ _ _ _ _ _ _ _ _ _ _ _ _ _ _ _ w1894 _ _ _ w1996 w2067 _ _ _ _ _ _ _ _ w2279 w2302 _ _ w2372 _ _ _]
                tunnel: w1293 -> [_ _ _ _ _ _ _ _ _ _ _ _ _ _ _ _ _ _ _ _ _ _ _ _ _ _ _ _ _ _ _ _ _ _ _ _ _ _ _ _ w2277 w2301 _ _ _ _ _ _]
                tunnel: w1289 -> [_ _ _ _ _ _ _ _ _ _ _ _ _ _ _ _ _ _ _ _ w1767 w1794 _ _ _ _ _ _ _ _ _ _ _ _ _ _ _ _ _ _ _ _ _ _ _ _ _ _]
                frame "Start1", Default {
                  w1387 = FALSE ("SelectionState")
                  n296 = xnode "Read/Write Control"("FPGA VI Reference In"=w1389, "error in"=w1388, "SelectionState"=w1387, "LR_reward_Laser_l1"=w1387, "LR_wrong_Laser_l1"=w1387, "LR_reward_Event_l1"=w1387, "LR_wrong_Event_l1"=w1387, "Left(F)_or_Right(T)"=w1387, "SelectionState"=w1387, "LR_reward_Laser_l2"=w1387, "LR_wrong_laser_l2"=w1387, "LR_reward_Event_l2"=w1387, "LR_wrong_Event_l2"=w1387, "LC_Event_l1"=w1387, "LC_Laser_l1"=w1387, "LC_Laser_l2"=w1387, "LC_Event_l2"=w1387, "CueLed_Event"=w1387) -> ("error out"=w1386:errorcluster)  [unwired: 1 out]
                  n297 = local write "error out"(w1386) -> ()
                }
                frame "Start2" {
                }
                frame "Start3" {
                  w1402 = u16 3 ("element")
                  w1400 = u16 0 ("element")
                  w1427 = u16 0 ("new element/subarray")
                  w1432 = 0.0 ("BTPR_avg_L")
                  w1435 = FALSE ("SolenoidReward")
                  w1433 = u16 0 ("BTPR_block")
                  w1436 = u16 0 ("nRewards_cur")
                  # "Goal:\nPrepare dataCurrent"
                  n298 = call "BRig_dataExp_FreeReward_c_L.vi"() -> ("output_FreeReward_c_L"=w1429:i32)  [unwired: 11 in]
                  n299 = call "BRig_dataExp_FreeReward_c_R.vi"() -> ("output_FreeReward_c_R"=w1428:i32)  [unwired: 11 in]
                  n300 = local write "nRewards_cur"(w1436) -> ()
                  n301 = local write "nRewards_total"(w1436) -> ()
                  n302 = local write "nRewards_Left"(w1436) -> ()
                  n303 = local write "nRewards_Right"(w1436) -> ()
                  n304 = local write "BUR_target"(w1436) -> ()
                  n305 = local write "TpB_target"(w1436) -> ()
                  n306 = local write "iBlock"(w1436) -> ()
                  n307 = local write "iTrial"(w1436) -> ()
                  n308 = local write "nTrial"(w1436) -> ()
                  n309 = local write "SolenoidReward"(w1435) -> ()
                  n310 = local write "allReward_L"(w1435) -> ()
                  n311 = local write "allReward_R"(w1435) -> ()
                  n312 = local write "BTPR_avg_L"(w1432) -> ()
                  n313 = local write "BTPR_avg_R"(w1432) -> ()
                  n314 = local write "T2R_avg_L"(w1432) -> ()
                  n315 = local write "T2R_avg_R"(w1432) -> ()
                  n316 = Replace Array Subset(array=w1431, new element #1=w1427, index #1=w1429, new element #2=w1427, index #2=w1428) -> (w1430:u16[])
                  n317 = call "BRig_dataRT_stats__T2R_cur.vi"() -> ("output_T2R_cur"=w1426:i32)  [unwired: 11 in]
                  n318 = call "BRig_dataRT_stats__BTPR_cur.vi"() -> ("output_BTPR_cur"=w1425:i32)  [unwired: 11 in]
                  n319 = call "BRig_dataRT_stats__T2R_avg_L.vi"() -> ("output_T2R_avg_L__x100"=w1420:i32)  [unwired: 11 in]
                  n320 = call "BRig_dataRT_stats__T2R_avg_R.vi"() -> ("output_T2R_avg_R__x100"=w1419:i32)  [unwired: 11 in]
                  n321 = call "BRig_dataRT_stats__BTPR_avg_L.vi"() -> ("output_BTPR_avg_L__x100"=w1424:i32)  [unwired: 11 in]
                  n322 = call "BRig_dataRT_stats__BTPR_avg_R.vi"() -> ("output_BTPR_avg_R__x100"=w1416:i32)  [unwired: 11 in]
                  n323 = call "BRig_dataRT_stats__nReward.vi"() -> ("output_nReward"=w1411:i32)  [unwired: 11 in]
                  n324 = call "BRig_dataRT_stats__nReward_left.vi"() -> ("output_nReward_left"=w1410:i32)  [unwired: 11 in]
                  n325 = call "BRig_dataRT_stats__nReward_right.vi"() -> ("output_nReward_right"=w1409:i32)  [unwired: 11 in]
                  n326 = local write "FreeReward_c_L"(w1427) -> ()
                  n327 = local write "FreeReward_c_R"(w1427) -> ()
                  n328 = local write "BTPR_block"(w1433) -> ()
                  n329 = local write "T2R_block"(w1433) -> ()
                  n330 = call "BRig_dataRT_stats__FreeReward_c_L.vi"() -> ("output_FreeReward_c_L"=w1405:i32)  [unwired: 11 in]
                  n331 = call "BRig_dataRT_stats__FreeReward_c_R.vi"() -> ("output_FreeReward_c_R"=w1404:i32)  [unwired: 11 in]
                  n332 = To Unsigned Word Integer(number=w1420) -> (unsigned 16bit integer=w1421:u16)
                  n333 = To Unsigned Word Integer(number=w1426) -> (unsigned 16bit integer=w1423:u16)
                  n334 = To Unsigned Word Integer(number=w1419) -> (unsigned 16bit integer=w1418:u16)
                  n335 = To Unsigned Word Integer(number=w1425) -> (unsigned 16bit integer=w1422:u16)
                  n336 = To Unsigned Word Integer(number=w1424) -> (unsigned 16bit integer=w1417:u16)
                  n337 = To Unsigned Word Integer(number=w1416) -> (unsigned 16bit integer=w1415:u16)
                  n338 = To Unsigned Word Integer(number=w1411) -> (unsigned 16bit integer=w1408:u16)
                  n339 = To Unsigned Word Integer(number=w1410) -> (unsigned 16bit integer=w1407:u16)
                  n340 = To Unsigned Word Integer(number=w1409) -> (unsigned 16bit integer=w1406:u16)
                  n341 = To Unsigned Word Integer(number=w1405) -> (unsigned 16bit integer=w1403:u16)
                  n342 = To Unsigned Word Integer(number=w1404) -> (unsigned 16bit integer=w1401:u16)
                  n343 = Build Array(w1402, w1423, w1400, w1402, w1422, w1400, w1402, w1421, w1400, w1402, w1418, w1400, w1402, w1417, w1400, w1402, w1415, w1400, w1402, w1408, w1400, w1402, w1407, w1400, w1402, w1406, w1400, w1402, w1403, w1400, w1402, w1401, w1400) -> (w1412:u16[])
                  n344 = RT FIFO Write(0:w1414, 1:w1412, 3:w1413) -> ()  [unwired: 2 in, 4 out]
                }
                frame "saveSettings1" {
                  w1454 = u16 3 ("element")
                  w1453 = u16 0 ("element")
                  n345 = call "BRig_dataRT_stats__nTrial.vi"() -> ("output_nTrial"=w1450:i32)  [unwired: 11 in]
                  n346 = call "BRig_dataRT_stats__iTrial.vi"() -> ("output_iTrial"=w1449:i32)  [unwired: 11 in]
                  n347 = call "BRig_dataRT_stats__iBlock.vi"() -> ("output_iBlock"=w1448:i32)  [unwired: 11 in]
                  n348 = call "BRig_dataRT_stats__nReward_cur.vi"() -> ("output_nReward_cur"=w1447:i32)  [unwired: 11 in]
                  n349 = call "BRig_dataRT_stats__TpB_target.vi"() -> ("output_TpB_target"=w1446:i32)  [unwired: 11 in]
                  n350 = call "BRig_dataRT_stats__BUR_target.vi"() -> ("output_BUR_target"=w1445:i32)  [unwired: 11 in]
                  n351 = call "BRig_dataRT_stats__DAB_nReward_HighProb.vi"() -> ("output_DAB_nReward_HighProb"=w1444:i32)  [unwired: 11 in]
                  n352 = call "BRig_dataRT_stats__DAB_nReward_LowProb.vi"() -> ("output_DAB_nReward_LowProb"=w1443:i32)  [unwired: 11 in]
                  n353 = call "BRig_dataRT_stats__DAB_nTimeout.vi"() -> ("output_DAB_nTimeout"=w1442:i32)  [unwired: 11 in]
                  n354 = To Unsigned Word Integer(number=w1448) -> (unsigned 16bit integer=w1462:u16)
                  n355 = To Unsigned Word Integer(number=w1450) -> (unsigned 16bit integer=w1464:u16)
                  n356 = To Unsigned Word Integer(number=w1447) -> (unsigned 16bit integer=w1461:u16)
                  n357 = To Unsigned Word Integer(number=w1449) -> (unsigned 16bit integer=w1463:u16)
                  n358 = To Unsigned Word Integer(number=w1446) -> (unsigned 16bit integer=w1460:u16)
                  n359 = To Unsigned Word Integer(number=w1445) -> (unsigned 16bit integer=w1459:u16)
                  n360 = To Unsigned Word Integer(number=w1444) -> (unsigned 16bit integer=w1457:u16)
                  n361 = To Unsigned Word Integer(number=w1443) -> (unsigned 16bit integer=w1456:u16)
                  n362 = To Unsigned Word Integer(number=w1442) -> (unsigned 16bit integer=w1455:u16)
                  n363 = Build Array(w1454, w1464, w1453, w1454, w1463, w1453, w1454, w1462, w1453, w1454, w1461, w1453, w1454, w1460, w1453, w1454, w1459, w1453, w1454, w1457, w1453, w1454, w1456, w1453, w1454, w1455, w1453) -> (w1458:u16[])
                  n364 = RT FIFO Write(0:w1452, 1:w1458, 3:w1451) -> ()  [unwired: 2 in, 4 out]
                }
                frame "setSettings_Laser" {
                  n365 = call "BRig_dataExp_LED_baseline_Cue.vi"() -> ("output_LED_baseline_Cue"=w1490:i32)  [unwired: 11 in]
                  n366 = call "BRig_dataExp_LED_baseline_l1.vi"() -> ("output_LED_baseline_l1"=w1491:i32)  [unwired: 11 in]
                  n367 = call "BRig_dataExp_LED_baseline_l2.vi"() -> ("output_LED_baseline_l2"=w1489:i32)  [unwired: 11 in]
                  n368 = call "BRig_dataExp_I_anySelect.vi"() -> ("output_I_anySelect"=w1483:i32)  [unwired: 11 in]
                  n369 = call "BRig_dataExp_I_trialUntilReward.vi"() -> ("output_I_trialUntilReward"=w1482:i32)  [unwired: 11 in]
                  n370 = local read "FPGA_count2ms"() -> (w1500:dbl)
                  n371 = call "BRig_RT__Case_Exp__State_setLaserSettings.vi"("input_FPGA_count2ms"=w1500, "input_dataExp"=w1481, "input_dataLC"=w1501) -> ("output_LR_nTotal_l1"=w1499:u32, "output_LR_nTotal_l2"=w1498:u32, "output_LR_reward_nDelay_l1"=w1497:u32, "output_LR_wrong_nDelay_l1"=w1496:u32, "output_LR_reward_nDelay_l2"=w1495:u32, "output_LR_wrong_nDelay_l2"=w1494:u32)  [unwired: 11 in]
                  n372 = Index Array(array=w1481, index #1=w1490, index #2=w1491, index #3=w1489, index #4=w1483, index #5=w1482) -> (element #1=w1488:u16, element #2=w1487:u16, element #3=w1486:u16, element #4=w1485:u16, element #5=w1484:u16)
                  n373 = Not Equal To 0?(x=w1487) -> (x != 0?=w1479:bool)
                  n374 = Not Equal To 0?(x=w1485) -> (x != 0?=w1477:bool)
                  n375 = Not Equal To 0?(x=w1488) -> (x != 0?=w1480:bool)
                  n376 = Not Equal To 0?(x=w1486) -> (x != 0?=w1478:bool)
                  n377 = Not Equal To 0?(x=w1484) -> (x != 0?=w1476:bool)
                  n378 = local read "LaserFiber_V_l1"() -> (w1474:dbl)
                  n379 = local read "LaserFiber_V_l2"() -> (w1472:dbl)
                  n380 = call "myRIO__convert__Voltage_to_FPGAvalue.vi"("input_voltage"=w1474) -> ("output_PortA"=w1473:u16)  [unwired: 9 in, 1 out]
                  n381 = call "myRIO__convert__Voltage_to_FPGAvalue.vi"("input_voltage"=w1472) -> ("output_PortA"=w1471:u16)  [unwired: 9 in, 1 out]
                  n382 = xnode "Read/Write Control"("FPGA VI Reference In"=w1502, "error in"=w1503, "LR_reward_nTotal_l1"=w1499, "LR_wrong_nTotal_l1"=w1499, "LR_reward_nTotal_l2"=w1498, "LR_wrong_nTotal_l2"=w1498, "LR_reward_nDelay_l1"=w1497, "LR_wrong_nDelay_l1"=w1496, "LR_reward_nDelay_l2"=w1495, "LR_wrong_nDelay_l2"=w1494, "CueLed_Baseline"=w1480, "L1Led_Baseline"=w1479, "L2Led_Baseline"=w1478, "I_allReward"=w1477, "ignoreWrong"=w1476, "AnaOut0_Pair"=w1473, "AnaOut1_Pair"=w1471) -> ("error out"=→"error out":errorcluster)  [unwired: 1 out]
                }
                frame "initBlock" {
                  w1507 = u16 0 ("element")
                  w1510 = u16 3
                  w1527 = u16 0 ("BTPR_block")
                  n383 = local write "nRewards_cur"(u16 0 ("nRewards_cur")) -> ()
                  n384 = local write "BTPR_block"(w1527) -> ()
                  n385 = local write "T2R_block"(w1527) -> ()
                  n386 = call "BRig_RT__Case_Exp__State_initBlock__v10.vi"("input_dataCurrent"=w1547, "input_dataExp"=w1546, "input_dataBlock"=w1543, "input_dataTrial"=w1541) -> ("output_iSpout"=w1532:u16, "output_speaker_amp_R"=w1536:u16, "output_iBlock"=w1516:u16, "output_speaker_freq_R"=w1537:u8, "output_BUR_target"=w1517:u16, "output_speaker_amp_L"=w1538:u16, "output_TpB_target"=w1518:u16, "output_speaker_freq_L"=w1539:u8, "output_dataCurrent"=w1545:u16[], "output_dataBlock"=w1542:u16[][], "output_dataTrial"=w1540:u16[][])  [unwired: 5 in]
                  n387 = Type Cast(type=enum16{"Left", "Right"}."Left", x=w1532) -> (*(type *) &x=w1529:enum16{"Left", "Right"})
                  n388 = Not Equal To 0?(x=w1532) -> (x != 0?=w1528:bool)
                  n389 = call "BRig_dataRT_stats__TpB_target.vi"() -> ("output_TpB_target"=w1519:i32)  [unwired: 11 in]
                  n390 = call "BRig_dataRT_stats__BUR_target.vi"() -> ("output_BUR_target"=w1520:i32)  [unwired: 11 in]
                  n391 = call "BRig_dataRT_stats__iBlock.vi"() -> ("output_iBlock"=w1521:i32)  [unwired: 11 in]
                  n392 = call "BRig_dataRT_stats__T2R_cur.vi"() -> ("output_T2R_cur"=w1514:i32)  [unwired: 11 in]
                  n393 = call "BRig_dataRT_stats__BTPR_cur.vi"() -> ("output_BTPR_cur"=w1513:i32)  [unwired: 11 in]
                  n394 = call "BRig_dataRT_stats__nReward_cur.vi"() -> ("output_nReward_cur"=w1509:i32)  [unwired: 11 in]
                  n395 = local write "cSpout"(w1529) -> ()
                  n396 = xnode "Read/Write Control"("FPGA VI Reference In"=w1535, "error in"=w1534, "Left(F)_or_Right(T)"=w1528, "audioFreq_L_kHz"=w1539, "audioAmp_L"=w1538, "audioFreq_R_kHz"=w1537, "audioAmp_R"=w1536) -> ("error out"=w1533:errorcluster)  [unwired: 1 out]
                  n397 = To Unsigned Word Integer(number=w1514) -> (unsigned 16bit integer=w1512:u16)
                  n398 = To Unsigned Word Integer(number=w1509) -> (unsigned 16bit integer=w1508:u16)
                  n399 = To Unsigned Word Integer(number=w1519) -> (unsigned 16bit integer=w1526:u16)
                  n400 = To Unsigned Word Integer(number=w1520) -> (unsigned 16bit integer=w1523:u16)
                  n401 = To Unsigned Word Integer(number=w1521) -> (unsigned 16bit integer=w1522:u16)
                  n402 = To Unsigned Word Integer(number=w1513) -> (unsigned 16bit integer=w1511:u16)
                  n403 = local write "error out"(w1533) -> ()
                  n404 = local write "iBlock"(w1516) -> ()
                  n405 = local write "BUR_target"(w1517) -> ()
                  n406 = local write "TpB_target"(w1518) -> ()
                  n407 = Build Array(w1510, w1526, w1518, w1510, w1523, w1517, w1510, w1522, w1516, w1510, w1512, w1507, w1510, w1511, w1507, w1510, w1508, w1507) -> (w1515:u16[])
                  n408 = RT FIFO Write(0:w1524, 1:w1515, 3:w1525) -> ()  [unwired: 2 in, 4 out]
                }
                frame "initTrial" {
                  w1552 = u16 3
                  n409 = xnode "Read/Write Control"("FPGA VI Reference In"=w1571, "error in"=w1562, "SelectionState"=FALSE) -> ("error out"=w1570:errorcluster)  [unwired: 1 out]
                  n410 = call "BRig_RT__Case_Exp__State_initTrial__v10.vi"("input_dataCurrent"=w1561, "input_dataBlock"=w1565, "input_dataTrial"=w1568, "input_dataExp"=w1549) -> ("output_iTrial"=w1550:u16, "output_nTrial"=w1551:u16, "output_SolenoidReward"=w1567:bool, "output_dataCurrent"=w1560:u16[], "output_dataBlock"=w1564:u16[][], "output_dataTrial"=w1563:u16[][])  [unwired: 6 in]
                  n411 = call "BRig_dataRT_stats__nTrial.vi"() -> ("output_nTrial"=w1554:i32)  [unwired: 11 in]
                  n412 = call "BRig_dataRT_stats__iTrial.vi"() -> ("output_iTrial"=w1553:i32)  [unwired: 11 in]
                  n413 = local write "iTrial"(w1550) -> ()
                  n414 = local write "nTrial"(w1551) -> ()
                  n415 = local write "SolenoidReward"(w1567) -> ()
                  n416 = To Unsigned Word Integer(number=w1554) -> (unsigned 16bit integer=w1559:u16)
                  n417 = To Unsigned Word Integer(number=w1553) -> (unsigned 16bit integer=w1557:u16)
                  n418 = local write "error out"(w1570) -> ()
                  n419 = Build Array(w1552, w1559, w1551, w1552, w1557, w1550) -> (w1558:u16[])
                  n420 = RT FIFO Write(0:w1556, 1:w1558, 3:w1555) -> ()  [unwired: 2 in, 4 out]
                }
                frame "initTrial2" {
                  n421 = call "BRig_RT__Case_Exp__State_initTrial2__v11.vi"("input_dataCurrent"=w1576, "input_dataTrial"=w1592, "input_dataExp"=w1575, "input_dataBlock"=w1590, "input_dataLC"=w1591) -> ("output_L_Wrong_Laser_l2"=w1582:bool, "output_L_Wrong_Event_l2"=w1583:bool, "output_L_Power_l1"=w1581:dbl, "output_L_Reward_Laser_l2"=w1584:bool, "output_L_Power_l2"=w1580:dbl, "output_L_Reward_Event_l2"=w1585:bool, "output_dataCurrent"=w1578:u16[], "output_dataTrial"=w1577:u16[][], "output_L_Reward_Event_l1"=w1589:bool, "output_L_Reward_Laser_l1"=w1588:bool, "output_L_Wrong_Event_l1"=w1587:bool, "output_L_Wrong_Laser_l1"=w1586:bool)  [unwired: 3 in]
                  n422 = local write "L_Power_l1"(w1581) -> ()
                  n423 = call "myRIO__convert__Voltage_to_FPGAvalue.vi"("input_voltage"=w1581) -> ("output_PortA"=w1573:u16)  [unwired: 9 in, 1 out]
                  n424 = local write "L_Power_l2"(w1580) -> ()
                  n425 = call "myRIO__convert__Voltage_to_FPGAvalue.vi"("input_voltage"=w1580) -> ("output_PortA"=w1574:u16)  [unwired: 9 in, 1 out]
                  n426 = xnode "Read/Write Control"("FPGA VI Reference In"=w1596, "error in"=w1595, "AnaOut_0"=w1573, "AnaOut_1"=w1574, "LR_reward_Event_l1"=w1589, "LR_reward_Laser_l1"=w1588, "LR_wrong_Event_l1"=w1587, "LR_wrong_Laser_l1"=w1586, "LR_reward_Event_l2"=w1585, "LR_reward_Laser_l2"=w1584, "LR_wrong_Event_l2"=w1583, "LR_wrong_laser_l2"=w1582) -> ("error out"=w1593:errorcluster)  [unwired: 1 out]
                  n427 = local write "error out"(w1593) -> ()
                  n428 = call "BRig_arrTrig_init.vi"() -> ("output_arrTrig"=w1579:bool[])  [unwired: 11 in]
                }
                frame "initTrial4" {
                  # "Dual Armed Bandit?"
                  # "resetOccurrence?\ndataAnalog"
                  n429 = local read "FPGA_count2ms"() -> (w1605:dbl)
                  n430 = local read "lick_Rising(F)_or_Falling(T)"() -> (w1601:bool)
                  n431 = call "BRig_dataExp_I_anySelect.vi"() -> ("output_I_anySelect"=w1600:i32)  [unwired: 11 in]
                  n432 = Index Array(array=w1598, index=w1600) -> (element=w1599:u16)
                  n433 = local read "Recording"() -> (w1607:bool)
                  n434 = call "BRig_RT_comm_tcp_write_RTwrite__RunState_Trial_start.vi"("input_dataCurrent"=w1604) -> ("output_strCmd"=w1603:string)  [unwired: 10 in]
                  n435 = Not Equal To 0?(x=w1599) -> (x != 0?=w1597:bool)
                  n436 = call "BRig_RT__Case_Exp__State_initTrial4.vi"("input_Recording"=w1607, "input_FPGA_count2ms"=w1605, "input_dataTrial"=w1608) -> ("output_Solenoid_nTotal"=w1606:u32, "output_dataTrial"=w1602:u16[][])  [unwired: 7 in]
                  n437 = case shown="False" w1597 {
                    tunnel: w1613 -> [w1622 w1627]
                    tunnel: w1612 -> [w1621 w1626]
                    tunnel: [w1620 w1625] -> w1611
                    tunnel: w1607 -> [w1619 w1624]
                    tunnel: w1606 -> [w1618 _]
                    tunnel: w1601 -> [w1617 w1623]
                    frame False {
                      n438 = xnode "Read/Write Control"("FPGA VI Reference In"=w1622, "error in"=w1621, "Solenoid_nTotal_L"=w1618, "Solenoid_nTotal_R"=w1618, "A6_Act"=w1619, "Rising(F)_or_Falling(T)"=w1617) -> ("error out"=w1620:errorcluster)  [unwired: 1 out]
                    }
                    frame True {
                      n439 = xnode "Read/Write Control"("FPGA VI Reference In"=w1627, "error in"=w1626, "A6_Act"=w1624, "Rising(F)_or_Falling(T)"=w1623) -> ("error out"=w1625:errorcluster)  [unwired: 1 out]
                    }
                  }
                  n440 = local write "error out"(w1611) -> ()
                }
                frame "initTrial_LC_ENL1" {
                  n441 = call "BRig_RT__Case_Exp__State_initTrial__LC_ENL__v10.vi"("input_arrTrig"=w1636, "input_dataTrial"=w1635, "input_dataExp"=w1628, "input_dataLC"=w1633, "input_dataCurrent"=w1629) -> ("output_dataTrial"=w1631:u16[][], "output_dataCurrent"=w1632:u16[], "output_arrTrig"=w1630:bool[])  [unwired: 4 in]
                }
                frame "initTrial_LC_Cue1" {
                  n442 = call "BRig_RT__Case_Exp__State_initTrial__LC_Cue__v10.vi"("input_arrTrig"=w1642, "input_dataTrial"=w1644, "input_dataExp"=w1638, "input_dataLC"=w1640, "input_dataCurrent"=w1639) -> ("output_dataTrial"=w1643:u16[][], "output_dataCurrent"=w1646:u16[], "output_arrTrig"=w1641:bool[])  [unwired: 4 in]
                }
                frame "initTrial_LC_Sel" {
                  n443 = call "BRig_RT__Case_Exp__State_initTrial__LC_Select__v10.vi"("input_arrTrig"=w1650, "input_dataTrial"=w1652, "input_dataExp"=w1648, "input_dataLC"=w1654, "input_dataCurrent"=w1656) -> ("output_dataTrial"=w1651:u16[][], "output_dataCurrent"=w1655:u16[], "output_arrTrig"=w1649:bool[])  [unwired: 4 in]
                  n444 = xnode "Read/Write Control"("FPGA VI Reference In"=w1659, "error in"=w1658, "A6_Act"=FALSE) -> ("error out"=w1660:errorcluster)  [unwired: 1 out]
                  n445 = local write "error out"(w1660) -> ()
                }
                frame "ENL1_pre" {
                  n446 = call "BRig_RT__Case_Exp__State_ENLPre__v4.vi"("input_arrTrig"=w1664, "input_ENL2"=FALSE, "input_I_lick"=w1670, "input_dataExp"=w1662, "input_dataTrial"=w1667, "input_dataCurrent"=w1668) -> ("output_arrTrig"=w1663:bool[], "output_dataTrial"=w1666:u16[][], "output_dataCurrent"=w1671:u16[], "output_state"=w1669:T2)  [unwired: 2 in]
                }
                frame "ENL2_pre" {
                  n447 = call "BRig_RT__Case_Exp__State_ENLPre__v4.vi"("input_arrTrig"=w1675, "input_ENL2"=TRUE, "input_I_lick"=w1682, "input_dataExp"=w1676, "input_dataTrial"=w1679, "input_dataCurrent"=w1680) -> ("output_arrTrig"=w1674:bool[], "output_dataTrial"=w1678:u16[][], "output_dataCurrent"=w1683:u16[], "output_state"=w1681:T2)  [unwired: 2 in]
                }
                frame "ENL1" {
                  n448 = call "BRig_RT__Case_Exp__State_ENL__v3.vi"("input_dataCurrent"=w1698, "input_dataTrial"=w1688, "input_ENL2"=FALSE, "input_arrTrig"=w1692, "input_state"=w1691, "I_lick"=w1690) -> ("output_l2_laserOn"=w1693:bool, "output_l2_laserEvent"=w1694:bool, "output_l1_laserOn"=w1695:bool, "output_state"=w1689:T2, "output_l1_laserEvent"=w1696:bool, "output_dataCurrent"=w1697:u16[], "output_dataTrial"=w1687:u16[][])  [unwired: 7 in]
                }
                frame "ENL2" {
                  n449 = call "BRig_RT__Case_Exp__State_ENL__v3.vi"("input_dataCurrent"=w1714, "input_dataTrial"=w1704, "input_ENL2"=TRUE, "input_arrTrig"=w1708, "input_state"=w1707, "I_lick"=w1706) -> ("output_l2_laserOn"=w1709:bool, "output_l2_laserEvent"=w1710:bool, "output_l1_laserOn"=w1711:bool, "output_state"=w1705:T2, "output_l1_laserEvent"=w1712:bool, "output_dataCurrent"=w1713:u16[], "output_dataTrial"=w1703:u16[][])  [unwired: 7 in]
                }
                frame "ENL1Penalty_pre" {
                  n450 = call "BRig_dataCurrent_c_generic.vi"() -> ("output_count_generic"=w1730:i32)  [unwired: 11 in]
                  n451 = call "BRig_dataCurrent_T_generic.vi"() -> ("output_T_generic"=w1728:i32)  [unwired: 11 in]
                  n452 = call "BRig_dataExp_T_ENLPenalty.vi"() -> ("output_ENL_penalty"=w1723:i32)  [unwired: 11 in]
                  n453 = Index Array(array=w1724, index=w1723) -> (element=w1727:u16)
                  n454 = Replace Array Subset(array=w1725, new element #1=u16 0 ("new element/subarray"), index #1=w1730, new element #2=w1727, index #2=w1728) -> (w1726:u16[])
                }
                frame "ENL1Penalty" {
                  n455 = call "BRig_RT__Case_Exp__generic__incrementCountTilThreshold.vi"("input_dataCurrent"=w1733) -> ("output_dataCurrent"=w1732:u16[], "output_underThreshold"=w1731:bool)  [unwired: 9 in]
                  n456 = Select(t=w1736, s=w1731, f=myRIO_BRig_RT__Case_Exp_stateList."ENL1_pre" ("Enum")) -> (s? t:f=w1734:T2)
                }
                frame "Cue1_pre" {
                  n457 = call "BRig_RT__Case_Exp__State_CuePre__v3.vi"("input_dataCurrent"=w1751, "input_dataTrial"=w1747, "input_Cue2"=FALSE ("input_ENL2"), "input_I_lick"=w1750, "input_dataExp"=w1748, "input_arrTrig"=w1744) -> ("output_state"=w1749:T2, "output_arrTrig"=w1743:bool[], "output_dataCurrent"=w1745:u16[], "output_dataTrial"=w1746:u16[][])  [unwired: 10 in]
                }
                frame "Cue2_pre" {
                  n458 = call "BRig_RT__Case_Exp__State_CuePre__v3.vi"("input_dataCurrent"=w1763, "input_dataTrial"=w1759, "input_Cue2"=TRUE ("input_ENL2"), "input_I_lick"=w1762, "input_dataExp"=w1760, "input_arrTrig"=w1756) -> ("output_state"=w1761:T2, "output_arrTrig"=w1755:bool[], "output_dataCurrent"=w1757:u16[], "output_dataTrial"=w1758:u16[][])  [unwired: 10 in]
                }
                frame "Cue1" {
                  n459 = call "BRig_RT__Case_Exp__State_Cue__v3.vi"("input_dataCurrent"=w1785, "input_dataTrial"=w1773, "input_dataExp"=w1767, "input_Cue2"=FALSE, "input_arrTrig"=w1781, "input_state"=w1783, "I_lick"=w1784) -> ("output_l2_laserOn"=w1777:bool, "output_l2_laserEvent"=w1778:bool, "output_SelectionState"=w1776:bool, "output_l1_laserOn"=w1779:bool, "output_state"=w1782:T2, "output_l1_laserEvent"=w1780:bool, "output_dataCurrent"=w1768:u16[], "output_dataTrial"=w1772:u16[][], "output_CueLed"=w1771:bool, "output_Audio_L"=w1770:bool, "output_Audio_R"=w1769:bool)  [unwired: 2 in]
                  n460 = case shown="True" w1776 {
                    selector: w1776 -> [_ w1791]
                    tunnel: w1775 -> [_ w1790]
                    tunnel: w1774 -> [_ w1789]
                    frame False {
                    }
                    frame True {
                      n461 = xnode "Read/Write Control"("FPGA VI Reference In"=w1789, "error in"=w1790, "SelectionState"=w1791) -> ("error out"=w1792:errorcluster)  [unwired: 1 out]
                      n462 = local write "error out"(w1792) -> ()
                    }
                  }
                }
                frame "Cue2" {
                  n463 = call "BRig_RT__Case_Exp__State_Cue__v3.vi"("input_dataCurrent"=w1812, "input_dataTrial"=w1800, "input_dataExp"=w1794, "input_Cue2"=TRUE, "input_arrTrig"=w1808, "input_state"=w1810, "I_lick"=w1811) -> ("output_l2_laserOn"=w1804:bool, "output_l2_laserEvent"=w1805:bool, "output_SelectionState"=w1803:bool, "output_l1_laserOn"=w1806:bool, "output_state"=w1809:T2, "output_l1_laserEvent"=w1807:bool, "output_dataCurrent"=w1795:u16[], "output_dataTrial"=w1799:u16[][], "output_CueLed"=w1798:bool, "output_Audio_L"=w1797:bool, "output_Audio_R"=w1796:bool)  [unwired: 2 in]
                  n464 = case shown="True" w1803 {
                    selector: w1803 -> [_ w1818]
                    tunnel: w1802 -> [_ w1817]
                    tunnel: w1801 -> [_ w1816]
                    frame False {
                    }
                    frame True {
                      n465 = xnode "Read/Write Control"("FPGA VI Reference In"=w1816, "error in"=w1817, "SelectionState"=w1818) -> ("error out"=w1819:errorcluster)  [unwired: 1 out]
                      n466 = local write "error out"(w1819) -> ()
                    }
                  }
                }
                frame "Cue1Penalty_pre" {
                  n467 = call "BRig_dataCurrent_c_generic.vi"() -> ("output_count_generic"=w1832:i32)  [unwired: 11 in]
                  n468 = call "BRig_dataCurrent_T_generic.vi"() -> ("output_T_generic"=w1830:i32)  [unwired: 11 in]
                  n469 = call "BRig_dataExp_T_CuePenalty.vi"() -> ("output_T_CuePenalty"=w1821:i32)  [unwired: 11 in]
                  n470 = Index Array(array=w1822, index=w1821) -> (element=w1820:u16)
                  n471 = Replace Array Subset(array=w1829, new element #1=u16 0 ("new element/subarray"), index #1=w1832, new element #2=w1820, index #2=w1830) -> (w1828:u16[])
                }
                frame "Cue1Penalty" {
                  n472 = call "BRig_RT__Case_Exp__generic__incrementCountTilThreshold.vi"("input_dataCurrent"=w1835) -> ("output_dataCurrent"=w1834:u16[], "output_underThreshold"=w1833:bool)  [unwired: 9 in]
                  n473 = Select(t=w1836, s=w1833, f=myRIO_BRig_RT__Case_Exp_stateList."ENL1_pre" ("Enum")) -> (s? t:f=w1837:T2)
                }
                frame "Selection_pre" {
                  n474 = xnode "Read/Write Control"("FPGA VI Reference In"=w1858, "error in"=w1859) -> ("error out"=w1857:errorcluster, "SelectReward"=w1854:bool, "SelectWrong"=w1855:bool)  [unwired: 1 out]
                  n475 = call "BRig_RT__Case_Exp__State_SelectPre.vi"("input_dataCurrent"=w1856, "input_SelectWrong"=w1855, "input_SelectReward"=w1854, "input_dataExp"=w1844, "input_LickL"=w1846, "input_LickR"=w1845, "input_arrTrig"=w1847) -> ("output_state"=w1853:T2, "output_dataCurrent"=w1852:u16[], "output_l1_laserEvent"=w1851:bool, "output_l1_laserOn"=w1850:bool, "output_l2_laserOn"=w1848:bool, "output_l2_laserEvent"=w1849:bool)  [unwired: 3 in]
                  n476 = local write "error out"(w1857) -> ()
                }
                frame "Selection" {
                  n477 = xnode "Read/Write Control"("FPGA VI Reference In"=w1883, "error in"=w1882) -> ("error out"=w1881:errorcluster, "SelectReward"=w1878:bool, "SelectWrong"=w1879:bool)  [unwired: 1 out]
                  n478 = call "BRig_RT__Case_Exp__State_Selection.vi"("input_state"=w1880, "input_dataCurrent"=w1873, "input_dataTrial"=w1864, "input_dataExp"=w1872, "input_arrTrig"=w1871, "input_FPGA_SelectWrong"=w1879, "input_FPGA_SelectReward"=w1878, "input_LickR"=w1877, "input_LickL"=w1876) -> ("output_LC_Laser_l2"=w1867:bool, "output_LC_Event_l2"=w1868:bool, "output_LC_Laser_l1"=w1869:bool, "output_LC_Event_l1"=w1870:bool, "output_state"=w1875:T2, "output_dataCurrent"=w1874:u16[], "output_dataTrial"=w1863:u16[][], "output_anySelect_L"=w1865:bool, "output_anySelect_R"=w1866:bool)  [unwired: 2 in]
                  n479 = local write "allReward_L"(w1865) -> ()
                  n480 = local write "allReward_R"(w1866) -> ()
                  n481 = local write "error out"(w1881) -> ()
                }
                frame "SelectReward_pre" {
                  # "Dual Armed\nBandit?"
                  n482 = call "BRig_dataExp_I_anySelect.vi"() -> ("output_I_anySelect"=w1899:i32)  [unwired: 11 in]
                  n483 = Index Array(array=w1897, index=w1899) -> (element=w1898:u16)
                  n484 = call "BRig_RT__Case_Exp__State_RewardPre__v11.vi"("input_dataCurrent"=w1915, "input_dataExp"=w1897, "input_dataBlock"=w1914, "input_dataTrial"=w1909, "input_dataLC"=w1886) -> ("output_T_Reward"=w1905:u16, "output_c_nReward_total_R"=w1890:u16, "output_c_nReward_total_L"=w1889:u16, "output_dataCurrent"=w1912:u16[], "output_DAB_L=L"=w1887:bool, "output_DAB_R=HighPorb"=w1888:bool, "output_dataBlock"=w1913:u16[][], "output_c_nReward_total"=w1892:u16, "output_nReward"=w1891:u16, "output_dataTrial"=w1908:u16[][])  [unwired: 1 in]
                  n485 = local read "FPGA_count2ms"() -> (w1904:dbl)
                  n486 = Not Equal To 0?(x=w1898) -> (x != 0?=w1896:bool)
                  n487 = case shown="True" w1896 {
                    tunnel: [w1921 w1943] -> w1893
                    tunnel: w1892 -> [w1920 w1940]
                    tunnel: w1891 -> [w1919 w1939]
                    tunnel: w1890 -> [w1918 w1942]
                    tunnel: w1889 -> [w1917 w1941]
                    tunnel: w1888 -> [_ w1933]
                    tunnel: w1887 -> [_ w1934]
                    frame False {
                      w1925 = u16 3
                      n488 = call "BRig_dataRT_stats__nReward_left.vi"() -> ("output_nReward_left"=w1922:i32)  [unwired: 11 in]
                      n489 = call "BRig_dataRT_stats__nReward_right.vi"() -> ("output_nReward_right"=w1923:i32)  [unwired: 11 in]
                      n490 = call "BRig_dataRT_stats__nReward_cur.vi"() -> ("output_nReward_cur"=w1924:i32)  [unwired: 11 in]
                      n491 = call "BRig_dataRT_stats__nReward.vi"() -> ("output_nReward"=w1927:i32)  [unwired: 11 in]
                      n492 = To Unsigned Word Integer(number=w1922) -> (unsigned 16bit integer=w1930:u16)
                      n493 = To Unsigned Word Integer(number=w1923) -> (unsigned 16bit integer=w1929:u16)
                      n494 = To Unsigned Word Integer(number=w1924) -> (unsigned 16bit integer=w1928:u16)
                      n495 = To Unsigned Word Integer(number=w1927) -> (unsigned 16bit integer=w1926:u16)
                      n496 = local write "nRewards_Right"(w1918) -> ()
                      n497 = local write "nRewards_Left"(w1917) -> ()
                      n498 = local write "nRewards_cur"(w1919) -> ()
                      n499 = local write "nRewards_total"(w1920) -> ()
                      n500 = Build Array(w1925, w1930, w1917, w1925, w1929, w1918, w1925, w1928, w1919, w1925, w1926, w1920) -> (w1921:u16[])
                    }
                    frame True {
                      w1945 = u16 3
                      n501 = call "BRig_dataRT_stats__nReward_left.vi"() -> ("output_nReward_left"=w1938:i32)  [unwired: 11 in]
                      n502 = call "BRig_dataRT_stats__nReward_right.vi"() -> ("output_nReward_right"=w1937:i32)  [unwired: 11 in]
                      n503 = call "BRig_dataRT_stats__DAB_nReward_HighProb.vi"() -> ("output_DAB_nReward_HighProb"=w1936:i32)  [unwired: 11 in]
                      n504 = call "BRig_dataRT_stats__DAB_nReward_LowProb.vi"() -> ("output_DAB_nReward_LowProb"=w1935:i32)  [unwired: 11 in]
                      n505 = call "BRig_dataRT_stats__nReward_cur.vi"() -> ("output_nReward_cur"=w1944:i32)  [unwired: 11 in]
                      n506 = call "BRig_dataRT_stats__nReward.vi"() -> ("output_nReward"=w1947:i32)  [unwired: 11 in]
                      n507 = Select(t=w1938, s=w1934, f=w1937) -> (s? t:f=w1931:i32)
                      n508 = Select(t=w1936, s=w1933, f=w1935) -> (s? t:f=w1932:i32)
                      n509 = To Unsigned Word Integer(number=w1931) -> (unsigned 16bit integer=w1950:u16)
                      n510 = To Unsigned Word Integer(number=w1932) -> (unsigned 16bit integer=w1949:u16)
                      n511 = To Unsigned Word Integer(number=w1944) -> (unsigned 16bit integer=w1948:u16)
                      n512 = To Unsigned Word Integer(number=w1947) -> (unsigned 16bit integer=w1946:u16)
                      n513 = local write "nRewards_cur"(w1939) -> ()
                      n514 = local write "nRewards_total"(w1940) -> ()
                      n515 = Build Array(w1945, w1950, w1941, w1945, w1949, w1942, w1945, w1948, w1939, w1945, w1946, w1940) -> (w1943:u16[])
                    }
                  }
                  n516 = To Double Precision Float(number=w1905) -> (double precision float=w1903:dbl)
                  n517 = Multiply(x=w1904, y=w1903) -> (x*y=w1901:dbl)
                  n518 = Round Toward +Infinity(x=w1901) -> (ceil(x): smallest int >= x=w1902:dbl)
                  n519 = To Unsigned Long Integer(number=w1902) -> (unsigned 32bit integer=w1900:u32)
                  n520 = RT FIFO Write(0:w1895, 1:w1893, 3:w1894) -> ()  [unwired: 2 in, 4 out]
                  n521 = call "BRig_RT_comm_tcp_write_RTwrite__RunState_Trial_selResult__v2.vi"("input_dataTrial"=w1908, "iReward_or_iError"=TRUE, "input_dataCurrent"=w1912) -> ("output_strCmd"=w1910:string)  [unwired: 8 in]
                  n522 = xnode "Read/Write Control"("FPGA VI Reference In"=w1907, "error in"=w1906, "Solenoid_nTotal_L"=w1900, "Solenoid_nTotal_R"=w1900) -> ()  [unwired: 2 out]
                }
                frame "SelectReward" {
                  n523 = call "BRig_dataCurrent_c_generic.vi"() -> ("output_count_generic"=w1957:i32)  [unwired: 11 in]
                  n524 = call "BRig_RT__Case_Exp__State_Reward.vi"("input_dataCurrent"=w1958, "input_state"=w1962, "input_dataExp"=w1960) -> ("output_state"=w1961:T2, "output_dataCurrent"=w1963:u16[], "output__L"=w1955:bool, "output__R"=w1954:bool)  [unwired: 5 in, 4 out]
                  n525 = Index Array(array=w1958, index=w1957) -> (element=w1956:u16)
                  n526 = Equal To 0?(x=w1956) -> (x = 0?=w1953:bool)
                  n527 = And(x=w1955, y=w1953) -> (x .and. y?=w1952:bool)
                  n528 = And(x=w1954, y=w1953) -> (x .and. y?=w1951:bool)
                }
                frame "SelectRewardPost_pre" {
                  n529 = call "BRig_dataExp_T_RewardPost.vi"() -> ("output_T_RewardPost"=w1969:i32)  [unwired: 11 in]
                  n530 = call "BRig_dataCurrent_c_generic.vi"() -> ("output_count_generic"=w1975:i32)  [unwired: 11 in]
                  n531 = call "BRig_dataCurrent_T_generic.vi"() -> ("output_T_generic"=w1974:i32)  [unwired: 11 in]
                  n532 = Index Array(array=w1970, index=w1969) -> (element=w1968:u16)
                  n533 = Replace Array Subset(array=w1972, new element #1=u16 0 ("new element/subarray"), index #1=w1975, new element #2=w1968, index #2=w1974) -> (w1971:u16[])
                }
                frame "SelectRewardPost" {
                  n534 = call "BRig_RT__Case_Exp__generic__incrementCountTilThreshold.vi"("input_dataCurrent"=w1980) -> ("output_dataCurrent"=w1978:u16[], "output_underThreshold"=w1979:bool)  [unwired: 9 in]
                  n535 = Select(t=w1982, s=w1979, f=myRIO_BRig_RT__Case_Exp_stateList."endTrial1" ("Enum")) -> (s? t:f=w1981:T2)
                }
                frame "SelectWrong_pre" {
                  # "Dual Armed\nBandit?"
                  n536 = call "BRig_dataExp_I_anySelect.vi"() -> ("output_I_anySelect"=w1992:i32)  [unwired: 11 in]
                  n537 = Index Array(array=w1993, index=w1992) -> (element=w1994:u16)
                  n538 = call "BRig_RT__Case_Exp__State_WrongOrTimeout_Pre__v11.vi"("input_dataCurrent"=w2010, "input_WorTO"=FALSE, "input_dataLC"=w1988, "input_dataBlock"=w2008, "input_dataTrial"=w2006, "input_dataExp"=w1993) -> ("output_T2R"=w1989:bool, "output_T2R_or_BTPR"=w1990:u16, "output_dataCurrent"=w2004:u16[], "output_dataBlock"=w2007:u16[][], "output_dataTrial"=w2003:u16[][], "output_BTPRavg"=w1999:dbl, "output_T2Ravg"=w2000:dbl, "output_R(F)_or_L(T)"=w2001:bool, "output_haveNewAvg"=w2002:bool)  [unwired: 1 out]
                  n539 = Not Equal To 0?(x=w1994) -> (x != 0?=w1991:bool)
                  n540 = case shown="False" w1991 {
                    tunnel: w2002 -> [_ w2026]
                    tunnel: w2001 -> [_ w2025]
                    tunnel: w2000 -> [_ w2024]
                    tunnel: w1999 -> [_ w2023]
                    tunnel: [w2015 w2021] -> w1997
                    tunnel: w1990 -> [w2013 w2017]
                    tunnel: w1989 -> [_ w2019]
                    frame True {
                      n541 = call "BRig_dataRT_stats__DAB_nTimeout.vi"() -> ("output_DAB_nTimeout"=w2012:i32)  [unwired: 11 in]
                      n542 = To Unsigned Word Integer(number=w2012) -> (unsigned 16bit integer=w2014:u16)
                      n543 = Build Array(u16 3, w2014, w2013) -> (w2015:u16[])
                    }
                    frame False {
                      n544 = case shown="False" w2019 {
                        tunnel: w2017 -> [w2028 w2030]
                        tunnel: [w2027 w2029] -> w2020
                        frame False {
                          n545 = call "BRig_dataRT_stats__BTPR_cur.vi"() -> ("output_BTPR_cur"=w2027:i32)  [unwired: 11 in]
                          n546 = local write "BTPR_block"(w2028) -> ()
                        }
                        frame True {
                          n547 = call "BRig_dataRT_stats__T2R_cur.vi"() -> ("output_T2R_cur"=w2029:i32)  [unwired: 11 in]
                          n548 = local write "T2R_block"(w2030) -> ()
                        }
                      }
                      n549 = To Unsigned Word Integer(number=w2020) -> (unsigned 16bit integer=w2018:u16)
                      n550 = case shown="True" w2026 {
                        tunnel: w2025 -> [_ w2050]
                        tunnel: w2024 -> [_ w2040]
                        tunnel: w2023 -> [_ w2036]
                        tunnel: u16 3 -> [w2034 w2043]
                        tunnel: w2018 -> [w2033 w2039]
                        tunnel: w2017 -> [w2032 w2042]
                        tunnel: [w2031 w2041] -> w2021
                        frame False {
                          n551 = Build Array(w2034, w2033, w2032) -> (w2031:u16[])
                        }
                        frame True {
                          w2035 = 100.0 ("y")
                          n552 = case shown="False" w2050 {
                            tunnel: w2040 -> [w2053 w2058]
                            tunnel: w2036 -> [w2054 w2057]
                            tunnel: [w2051 w2056] -> w2049
                            tunnel: [w2052 w2055] -> w2048
                            frame False {
                              n553 = local write "BTPR_avg_R"(w2054) -> ()
                              n554 = call "BRig_dataRT_stats__BTPR_avg_R.vi"() -> ("output_BTPR_avg_R__x100"=w2052:i32)  [unwired: 11 in]
                              n555 = local write "T2R_avg_R"(w2053) -> ()
                              n556 = call "BRig_dataRT_stats__T2R_avg_R.vi"() -> ("output_T2R_avg_R__x100"=w2051:i32)  [unwired: 11 in]
                            }
                            frame True {
                              n557 = call "BRig_dataRT_stats__BTPR_avg_L.vi"() -> ("output_BTPR_avg_L__x100"=w2055:i32)  [unwired: 11 in]
                              n558 = local write "BTPR_avg_L"(w2057) -> ()
                              n559 = local write "T2R_avg_L"(w2058) -> ()
                              n560 = call "BRig_dataRT_stats__T2R_avg_L.vi"() -> ("output_T2R_avg_L__x100"=w2056:i32)  [unwired: 11 in]
                            }
                          }
                          n561 = Multiply(x=w2040, y=w2035) -> (x*y=w2037:dbl)
                          n562 = Multiply(x=w2036, y=w2035) -> (x*y=w2038:dbl)
                          n563 = To Unsigned Word Integer(number=w2037) -> (unsigned 16bit integer=w2044:u16)
                          n564 = To Unsigned Word Integer(number=w2038) -> (unsigned 16bit integer=w2045:u16)
                          n565 = To Unsigned Word Integer(number=w2048) -> (unsigned 16bit integer=w2046:u16)
                          n566 = To Unsigned Word Integer(number=w2049) -> (unsigned 16bit integer=w2047:u16)
                          n567 = Build Array(w2043, w2047, w2044, w2043, w2046, w2045, w2043, w2039, w2042) -> (w2041:u16[])
                        }
                      }
                    }
                  }
                  n568 = RT FIFO Write(0:w1998, 1:w1997, 3:w1996) -> ()  [unwired: 2 in, 4 out]
                  n569 = call "BRig_RT_comm_tcp_write_RTwrite__RunState_Trial_selResult__v2.vi"("input_dataTrial"=w2003, "iReward_or_iError"=FALSE, "input_dataCurrent"=w2004) -> ("output_strCmd"=w1995:string)  [unwired: 8 in]
                }
                frame "SelectTimeout_pre" {
                  # "Dual Armed\nBandit?"
                  n570 = call "BRig_dataExp_I_anySelect.vi"() -> ("output_I_anySelect"=w2063:i32)  [unwired: 11 in]
                  n571 = Index Array(array=w2064, index=w2063) -> (element=w2065:u16)
                  n572 = call "BRig_RT__Case_Exp__State_WrongOrTimeout_Pre__v11.vi"("input_dataCurrent"=w2081, "input_WorTO"=TRUE, "input_dataLC"=w2059, "input_dataBlock"=w2079, "input_dataTrial"=w2077, "input_dataExp"=w2064) -> ("output_T2R"=w2060:bool, "output_T2R_or_BTPR"=w2061:u16, "output_dataCurrent"=w2075:u16[], "output_dataBlock"=w2078:u16[][], "output_dataTrial"=w2074:u16[][], "output_BTPRavg"=w2070:dbl, "output_T2Ravg"=w2071:dbl, "output_R(F)_or_L(T)"=w2072:bool, "output_haveNewAvg"=w2073:bool)  [unwired: 1 out]
                  n573 = Not Equal To 0?(x=w2065) -> (x != 0?=w2062:bool)
                  n574 = case shown="False" w2062 {
                    tunnel: w2073 -> [_ w2097]
                    tunnel: w2072 -> [_ w2096]
                    tunnel: w2071 -> [_ w2095]
                    tunnel: w2070 -> [_ w2094]
                    tunnel: [w2086 w2092] -> w2068
                    tunnel: w2061 -> [w2084 w2088]
                    tunnel: w2060 -> [_ w2090]
                    frame True {
                      n575 = call "BRig_dataRT_stats__DAB_nTimeout.vi"() -> ("output_DAB_nTimeout"=w2083:i32)  [unwired: 11 in]
                      n576 = To Unsigned Word Integer(number=w2083) -> (unsigned 16bit integer=w2085:u16)
                      n577 = Build Array(u16 3, w2085, w2084) -> (w2086:u16[])
                    }
                    frame False {
                      n578 = case shown="False" w2090 {
                        tunnel: w2088 -> [w2099 w2101]
                        tunnel: [w2098 w2100] -> w2091
                        frame False {
                          n579 = call "BRig_dataRT_stats__BTPR_cur.vi"() -> ("output_BTPR_cur"=w2098:i32)  [unwired: 11 in]
                          n580 = local write "BTPR_block"(w2099) -> ()
                        }
                        frame True {
                          n581 = call "BRig_dataRT_stats__T2R_cur.vi"() -> ("output_T2R_cur"=w2100:i32)  [unwired: 11 in]
                          n582 = local write "T2R_block"(w2101) -> ()
                        }
                      }
                      n583 = To Unsigned Word Integer(number=w2091) -> (unsigned 16bit integer=w2089:u16)
                      n584 = case shown="True" w2097 {
                        tunnel: w2096 -> [_ w2121]
                        tunnel: w2095 -> [_ w2111]
                        tunnel: w2094 -> [_ w2107]
                        tunnel: u16 3 -> [w2105 w2114]
                        tunnel: w2089 -> [w2104 w2110]
                        tunnel: w2088 -> [w2103 w2113]
                        tunnel: [w2102 w2112] -> w2092
                        frame False {
                          n585 = Build Array(w2105, w2104, w2103) -> (w2102:u16[])
                        }
                        frame True {
                          w2106 = 100.0 ("y")
                          n586 = case shown="False" w2121 {
                            tunnel: w2111 -> [w2124 w2129]
                            tunnel: w2107 -> [w2125 w2128]
                            tunnel: [w2122 w2127] -> w2120
                            tunnel: [w2123 w2126] -> w2119
                            frame False {
                              n587 = local write "BTPR_avg_R"(w2125) -> ()
                              n588 = call "BRig_dataRT_stats__BTPR_avg_R.vi"() -> ("output_BTPR_avg_R__x100"=w2123:i32)  [unwired: 11 in]
                              n589 = local write "T2R_avg_R"(w2124) -> ()
                              n590 = call "BRig_dataRT_stats__T2R_avg_R.vi"() -> ("output_T2R_avg_R__x100"=w2122:i32)  [unwired: 11 in]
                            }
                            frame True {
                              n591 = call "BRig_dataRT_stats__BTPR_avg_L.vi"() -> ("output_BTPR_avg_L__x100"=w2126:i32)  [unwired: 11 in]
                              n592 = local write "BTPR_avg_L"(w2128) -> ()
                              n593 = local write "T2R_avg_L"(w2129) -> ()
                              n594 = call "BRig_dataRT_stats__T2R_avg_L.vi"() -> ("output_T2R_avg_L__x100"=w2127:i32)  [unwired: 11 in]
                            }
                          }
                          n595 = Multiply(x=w2111, y=w2106) -> (x*y=w2108:dbl)
                          n596 = Multiply(x=w2107, y=w2106) -> (x*y=w2109:dbl)
                          n597 = To Unsigned Word Integer(number=w2108) -> (unsigned 16bit integer=w2115:u16)
                          n598 = To Unsigned Word Integer(number=w2109) -> (unsigned 16bit integer=w2116:u16)
                          n599 = To Unsigned Word Integer(number=w2119) -> (unsigned 16bit integer=w2117:u16)
                          n600 = To Unsigned Word Integer(number=w2120) -> (unsigned 16bit integer=w2118:u16)
                          n601 = Build Array(w2114, w2118, w2115, w2114, w2117, w2116, w2114, w2110, w2113) -> (w2112:u16[])
                        }
                      }
                    }
                  }
                  n602 = RT FIFO Write(0:w2069, 1:w2068, 3:w2067) -> ()  [unwired: 2 in, 4 out]
                  n603 = call "BRig_RT_comm_tcp_write_RTwrite__RunState_Trial_selResult__v2.vi"("input_dataTrial"=w2074, "iReward_or_iError"=FALSE, "input_dataCurrent"=w2075) -> ("output_strCmd"=w2066:string)  [unwired: 8 in]
                }
                frame "SelectWrong" {
                  n604 = call "BRig_RT__Case_Exp__generic__incrementCountTilThreshold.vi"("input_dataCurrent"=w2132) -> ("output_dataCurrent"=w2130:u16[], "output_underThreshold"=w2131:bool)  [unwired: 9 in]
                  n605 = Select(t=w2134, s=w2131, f=myRIO_BRig_RT__Case_Exp_stateList."endTrial1" ("Enum")) -> (s? t:f=w2133:T2)
                }
                frame "SelectTimeout" {
                  n606 = call "BRig_RT__Case_Exp__generic__incrementCountTilThreshold.vi"("input_dataCurrent"=w2142) -> ("output_dataCurrent"=w2141:u16[], "output_underThreshold"=w2140:bool)  [unwired: 9 in]
                  n607 = Select(t=w2144, s=w2140, f=myRIO_BRig_RT__Case_Exp_stateList."endTrial1" ("Enum")) -> (s? t:f=w2143:T2)
                }
                frame "endTrial1" {
                  n608 = call "BRig_RT_comm_tcp_write_RTwrite__RunState_Trial_end.vi"("input_dataCurrent"=w2158) -> ("output_strCmd"=w2157:string)  [unwired: 10 in]
                  n609 = call "BRig_RT__Case_Exp__State_endTrial__v10.vi"("input_dataBlock"=w2154, "input_timeStamp_start"=w2159, "input_dataTrial"=w2166, "input_dataCurrent"=w2158) -> ("output_BTPRavg"=w2151:dbl, "output_T2Ravg"=w2152:dbl, "output_dataTrial"=w2165:u16[][], "output_dataCurrent"=w2160:u16[], "output_R(F)_or_L(T)"=w2153:bool, "output_runTime"=→"T_ExpRun_min":dbl)  [unwired: 2 in]
                  n610 = xnode "Read/Write Control"("FPGA VI Reference In"=w2162, "error in"=w2161, "SelectionState"=FALSE) -> ("error out"=w2163:errorcluster)  [unwired: 1 out]
                  n611 = case shown="False" w2153 {
                    tunnel: w2152 -> [w2168 w2171]
                    tunnel: w2151 -> [w2169 w2170]
                    frame False {
                      n612 = local write "BTPR_avg_R"(w2169) -> ()
                      n613 = local write "T2R_avg_R"(w2168) -> ()
                    }
                    frame True {
                      n614 = local write "BTPR_avg_L"(w2170) -> ()
                      n615 = local write "T2R_avg_L"(w2171) -> ()
                    }
                  }
                  n616 = local write "error out"(w2163) -> ()
                }
                frame "endTrial2" {
                  n617 = case shown="True" w2181 {
                    tunnel: [w2189 _] -> w2182
                    tunnel: [w2188 w2191] -> w2177
                    tunnel: w2176 -> [w2186 w2199]
                    tunnel: w2175 -> [w2187 w2197]
                    tunnel: [w2187 w2196] -> w2174
                    tunnel: [w2186 w2198] -> w2173
                    tunnel: w2172 -> [_ w2190]
                    frame False {
                      # "Receive commands"
                      n618 = call "BRig_RT__Case_Exp__UploadClosedLoop__v3.vi"() -> ("all rows"=w2189:i64[][], "output_haveCmd"=w2188:bool)  [unwired: 10 in]
                    }
                    frame True {
                      # "Parse commands and update"
                      n619 = Array Size(array=w2190) -> (size(s)=w2195:i32[])
                      n620 = Index Array(array=w2195, index=0) -> (element=w2193:i32)
                      n621 = Not Equal To 0?(x=w2193) -> (x != 0?=w2192:bool)
                      n622 = case shown="False" w2192 {
                        selector: w2192 -> [w2203 w2205]
                        tunnel: w2199 -> [w2201 w2209]
                        tunnel: [w2201 w2208] -> w2198
                        tunnel: w2197 -> [w2200 w2207]
                        tunnel: [w2200 w2206] -> w2196
                        tunnel: [w2203 w2205] -> w2191
                        tunnel: w2190 -> [_ w2204]
                        frame False {
                          w2202 = TRUE ("input_setValues")
                          # "Update"
                          n623 = call "BRig_RT_panel_cue_v1,10.vi"("input_setValues"=w2202, "input_dataExp"=w2201) -> ()  [unwired: 9 in, 1 out]
                          n624 = call "BRig_RT_panel_ExpStruct_v1,13.vi"("input_setValues"=w2202, "input_dataExp"=w2201) -> ()  [unwired: 9 in, 1 out]
                          n625 = call "BRig_RT_panel_Laser1_v1,13.vi"("input_setValues"=w2202, "input_dataExp"=w2201, "input_dataLC"=w2200) -> ()  [unwired: 7 in, 2 out]
                          n626 = call "BRig_RT_panel_Laser2_v1,13.vi"("input_setValues"=w2202, "input_dataExp"=w2201, "input_dataLC"=w2200) -> ()  [unwired: 7 in, 2 out]
                        }
                        frame True {
                          # "Parse"
                          n627 = call "BRig_RT__Case_Exp__UploadClosedLoop__updateSettings.vi"("input_newSettings"=w2204, "input_dataLC"=w2207, "input_dataExp"=w2209) -> ("output_dataLC"=w2206:u16[], "output_dataExp"=w2208:u16[])  [unwired: 7 in]
                        }
                      }
                    }
                  }
                  n628 = Select(t=myRIO_BRig_RT__Case_Exp_stateList."endTrial2", s=w2177, f=myRIO_BRig_RT__Case_Exp_stateList."endTrial3" ("Enum")) -> (s? t:f=w2178:T2)
                }
                frame "endTrial3" {
                  n629 = call "BRig_RT__Case_Exp__endTrial_checkFreeReward__v10.vi"("input_dataBlock"=w2211, "input_dataExp"=w2220, "input_dataTrial"=w2221, "input_dataCurrent"=w2222) -> ("output_state"=w2212:T2, "output_endBlock"=w2210:bool)  [unwired: 6 in]
                  n630 = local read "STOP_endTrial"() -> (w2219:bool)
                  n631 = local read "STOP_abort"() -> (w2218:bool)
                  n632 = local read "START"() -> (w2216:bool)
                  n633 = Not(x=w2216) -> (.not. x?=w2217:bool)
                  n634 = Compound Arithmetic op=OR(w2219, w2217, w2218, w2210) -> (w2215:bool)
                  n635 = Select(t=myRIO_BRig_RT__Case_Exp_stateList."saveData_dataBlock" ("Enum"), s=w2215, f=w2212) -> (s? t:f=w2213:T2)
                }
                frame "endBlock" {
                  # "Get latest\nlaserSwitch"
                  n636 = call "BRig_dataExp_Loop_c_ExpStruct.vi"() -> ("output_Loop_c_ExpStruct"=w2231:i32)  [unwired: 11 in]
                  n637 = call "BRig_dataExp_LaserSwitch.vi"() -> ("output_LaserSwitch"=w2226:i32)  [unwired: 11 in]
                  n638 = local read "START"() -> (w2250:bool)
                  n639 = local read "STOP_endBlock"() -> (w2246:bool)
                  n640 = local read "STOP_endTrial"() -> (w2248:bool)
                  n641 = local read "STOP_abort"() -> (w2247:bool)
                  n642 = Replace Array Subset(array=w2224, new element=u16 2 ("new element/subarray"), index=w2231) -> (w2229:u16[])
                  n643 = call "BRig_RT_panel_ExpStruct_v1,13.vi"("input_setValues"=FALSE, "input_dataExp"=w2229) -> ("output_dataExp"=w2228:u16[])  [unwired: 9 in]
                  n644 = Index Array(array=w2228, index=w2226) -> (element=w2225:u16)
                  n645 = Not(x=w2250) -> (.not. x?=w2249:bool)
                  n646 = Select(t=myRIO_BRig_RT__Case_Exp_stateList."commUpload_dataTrial" ("Enum"), s=w2236, f=myRIO_BRig_RT__Case_Exp_stateList."initBlock" ("Enum")) -> (s? t:f=w2233:T2)
                  n647 = Replace Array Subset(array=w2224, new element=w2225, index=w2226) -> (w2227:u16[])
                  n648 = Compound Arithmetic op=OR(w2249, w2246, w2248, w2247) -> (w2240:bool)
                  n649 = Select(t=myRIO_BRig_RT__Case_Exp_stateList."endExp" ("Enum"), s=w2240, f=w2233) -> (s? t:f=w2251:T2)
                  n650 = Select(t="<S,E>" ("string"), s=w2240, f="") -> (s? t:f=w2237:string)
                }
                frame "endExp" {
                  n651 = xnode "Read/Write Control"("FPGA VI Reference In"=w2255, "error in"=w2254, "A6_Act"=FALSE) -> ("error out"=w2256:errorcluster)  [unwired: 1 out]
                  n652 = local write "error out"(w2256) -> ()
                }
                frame "commUpload_dataTrial" {
                }
                frame "saveData_dataBlock" {
                  n653 = Increment(x=w2285) -> (x+1=w2283:u16)
                  n654 = Replace Array Subset(array=w2277, new element=u16 2 ("new element/subarray"), index=0) -> (w2271:u16[])
                  n655 = Index Array(array=w2269, index (row)=0) -> (element=w2272:u16[])  [unwired: 1 in]
                  n656 = for {
                    tunnel: w2272 -> [w2295] mode=indexing
                    shift-right: [w2294] -> w2270
                    shift-left: w2271 -> [w2298]
                    i -> [w2297]
                    n657 = Increment(x=w2297) -> (x+1=w2296:i32)
                    n658 = Replace Array Subset(array=w2298, new element=w2295, index=w2296) -> (w2294:u16[])
                  }
                  n659 = RT FIFO Write(0:w2280, 1:w2270, 3:w2279) -> (11:w2282:errorcluster)  [unwired: 2 in, 3 out]
                  n660 = Unbundle By Name(w2282) -> ("code"=w2281:i32)
                  n661 = Greater?(x=w2283, y=u16 3) -> (0:w2291:bool)
                  n662 = Equal To 0?(x=w2281) -> (x = 0?=w2278:bool)
                  n663 = Or(x=w2291, y=w2278) -> (x .or. y?=w2290:bool)
                  n664 = Select(t=myRIO_BRig_RT__Case_Exp_stateList."endBlock" ("Enum"), s=w2290, f=w2286) -> (s? t:f=w2284:T2)
                }
                frame "saveData_dataTrial" {
                  n665 = Increment(x=w2316) -> (x+1=w2315:u16)
                  n666 = Replace Array Subset(array=w2301, new element=u16 1 ("new element/subarray"), index=0) -> (w2305:u16[])
                  n667 = Index Array(array=w2300, index (row)=0) -> (element=w2306:u16[])  [unwired: 1 in]
                  n668 = for {
                    tunnel: w2306 -> [w2325] mode=indexing
                    shift-right: [w2324] -> w2304
                    shift-left: w2305 -> [w2328]
                    i -> [w2327]
                    n669 = Increment(x=w2327) -> (x+1=w2326:i32)
                    n670 = Replace Array Subset(array=w2328, new element=w2325, index=w2326) -> (w2324:u16[])
                  }
                  n671 = RT FIFO Write(0:w2303, 1:w2304, 3:w2302) -> (11:w2311:errorcluster)  [unwired: 2 in, 3 out]
                  n672 = Unbundle By Name(w2311) -> ("code"=w2310:i32)
                  n673 = Equal To 0?(x=w2310) -> (x = 0?=w2299:bool)
                  n674 = Greater?(x=w2315, y=u16 3) -> (0:w2313:bool)
                  n675 = Or(x=w2313, y=w2299) -> (x .or. y?=w2312:bool)
                  n676 = Select(t=myRIO_BRig_RT__Case_Exp_stateList."endTrial2" ("Enum"), s=w2312, f=w2317) -> (s? t:f=w2318:T2)
                }
                frame "dummyState" {
                  n677 = call "BRig_dataCurrent_iTrial.vi"() -> ("output_iTrial"=w2335:i32)  [unwired: 11 in]
                  n678 = Index Array(array=w2336, index=w2335) -> (element=w2334:u16)
                  n679 = Equal?(x=w2334, y=u16 1) -> (x = y?=w2332:bool)
                  n680 = Equal To 0?(x=w2343) -> (x = 0?=w2344:bool)
                  n681 = Select(t=u16 13, s=w2332, f=u16 15) -> (s? t:f=w2329:u16)
                  n682 = Select(t=w2329, s=w2344, f=w2343) -> (s? t:f=w2342:u16)
                  n683 = Decrement(x=w2342) -> (x-1=w2341:u16)
                  n684 = Equal To 0?(x=w2341) -> (x = 0?=w2340:bool)
                  n685 = Select(t=myRIO_BRig_RT__Case_Exp_stateList."initTrial" ("Enum"), s=w2340, f=w2338) -> (s? t:f=w2337:T2)
                }
                frame "dummyState_endBlock" {
                  n686 = call "BRig_dataCurrent_iTrial.vi"() -> ("output_iTrial"=w2359:i32)  [unwired: 11 in]
                  n687 = Index Array(array=w2353, index=w2359) -> (element=w2349:u16)
                  n688 = Equal?(x=w2349, y=u16 1) -> (x = y?=w2357:bool)
                  n689 = Equal To 0?(x=w2350) -> (x = 0?=w2361:bool)
                  n690 = Select(t=u16 1, s=w2357, f=u16 3) -> (s? t:f=w2354:u16)
                  n691 = Select(t=w2354, s=w2361, f=w2350) -> (s? t:f=w2360:u16)
                  n692 = Decrement(x=w2360) -> (x-1=w2351:u16)
                  n693 = Equal To 0?(x=w2351) -> (x = 0?=w2352:bool)
                  n694 = Select(t=myRIO_BRig_RT__Case_Exp_stateList."initBlock" ("Enum"), s=w2352, f=w2363) -> (s? t:f=w2362:T2)
                }
                frame "FreeReward_pre" {
                  w2399 = u16 0 ("new element/subarray")
                  # "Duration = MTrig duration"
                  # "Duration = Reward Time"
                  n695 = call "BRig_dataCurrent_FreeReward_c.vi"() -> ("output_FreeReward_c"=w2400:i32)  [unwired: 11 in]
                  n696 = call "BRig_dataCurrent_iSpout.vi"() -> ("output_iSpout"=w2397:i32)  [unwired: 11 in]
                  n697 = call "BRig_dataCurrent_c_generic.vi"() -> ("output_count_generic"=w2406:i32)  [unwired: 11 in]
                  n698 = call "BRig_dataCurrent_T_generic.vi"() -> ("output_T_generic"=w2405:i32)  [unwired: 11 in]
                  n699 = Index Array(array=w2398, index=w2397) -> (element=w2396:u16)
                  n700 = call "BRig_dataMTrig_Solenoid_T_L.vi"() -> ("output_Solenoid_T_L"=w2395:i32)  [unwired: 11 in]
                  n701 = call "BRig_dataMTrig_Solenoid_T_R.vi"() -> ("output_Solenoid_T_R"=w2394:i32)  [unwired: 11 in]
                  n702 = local read "FPGA_count2ms"() -> (w2376:dbl)
                  n703 = call "BRig_dataTrial_T_Reward.vi"() -> ("output_T_Reward"=w2401:i32)  [unwired: 11 in]
                  n704 = Equal To 0?(x=w2396) -> (x = 0?=w2378:bool)
                  n705 = Select(t=w2395, s=w2378, f=w2394) -> (s? t:f=w2392:i32)
                  n706 = Index Array(array=w2402, index (row)=0 ("disabled index (row)"), index (col)=w2401) -> ()  [unwired: 1 out]
                  n707 = Index Array(array=w2393, index=w2392) -> (element=w2389:u16)
                  n708 = Replace Array Subset(array=w2398, new element #1=w2399, index #1=w2400, new element #2=w2399, index #2=w2406, new element #3=w2389, index #3=w2405) -> (w2404:u16[])
                  n709 = To Double Precision Float(number=w2389) -> (double precision float=w2377:dbl)
                  n710 = Multiply(x=w2377, y=w2376) -> (x*y=w2390:dbl)
                  n711 = call "BRig_dataExp_FreeReward_c_L.vi"() -> ("output_FreeReward_c_L"=w2383:i32)  [unwired: 11 in]
                  n712 = call "BRig_dataExp_FreeReward_c_R.vi"() -> ("output_FreeReward_c_R"=w2384:i32)  [unwired: 11 in]
                  n713 = Round Toward +Infinity(x=w2390) -> (ceil(x): smallest int >= x=w2391:dbl)
                  n714 = Select(t=w2383, s=w2378, f=w2384) -> (s? t:f=w2380:i32)
                  n715 = To Unsigned Long Integer(number=w2391) -> (unsigned 32bit integer=w2386:u32)
                  n716 = xnode "Read/Write Control"("FPGA VI Reference In"=w2388, "error in"=w2387, "Solenoid_nTotal_L"=w2386, "Solenoid_nTotal_R"=w2386) -> ()  [unwired: 2 out]
                  n717 = Index Array(array=w2381, index=w2380) -> (element=w2379:u16)
                  n718 = Increment(x=w2379) -> (x+1=w2369:u16)
                  n719 = case shown="True" w2378 {
                    tunnel: w2369 -> [w2410 w2412]
                    tunnel: [w2409 w2411] -> w2371
                    frame True {
                      n720 = local write "FreeReward_c_L"(w2410) -> ()
                      n721 = call "BRig_dataRT_stats__FreeReward_c_L.vi"() -> ("output_FreeReward_c_L"=w2409:i32)  [unwired: 11 in]
                    }
                    frame False {
                      n722 = local write "FreeReward_c_R"(w2412) -> ()
                      n723 = call "BRig_dataRT_stats__FreeReward_c_R.vi"() -> ("output_FreeReward_c_R"=w2411:i32)  [unwired: 11 in]
                    }
                  }
                  n724 = To Unsigned Word Integer(number=w2371) -> (unsigned 16bit integer=w2370:u16)
                  n725 = Build Array(u16 3, w2370, w2369) -> (w2375:u16[])
                  n726 = Replace Array Subset(array=w2381, new element=w2369, index=w2380) -> (w2382:u16[])
                  n727 = RT FIFO Write(0:w2373, 1:w2375, 3:w2372) -> ()  [unwired: 2 in, 4 out]
                }
                frame "FreeReward" {
                  n728 = call "BRig_dataCurrent_iSpout.vi"() -> ("output_iSpout"=w2423:i32)  [unwired: 11 in]
                  n729 = call "BRig_dataCurrent_c_generic.vi"() -> ("output_count_generic"=w2417:i32)  [unwired: 11 in]
                  n730 = Index Array(array=w2424, index #1=w2423, index #2=w2417) -> (element #1=w2422:u16, element #2=w2416:u16)
                  n731 = Equal To 0?(x=w2422) -> (x = 0?=w2420:bool)
                  n732 = Equal To 0?(x=w2416) -> (x = 0?=w2415:bool)
                  n733 = Not(x=w2420) -> (.not. x?=w2421:bool)
                  n734 = call "BRig_RT__Case_Exp__generic__incrementCountTilThreshold.vi"("input_dataCurrent"=w2424) -> ("output_dataCurrent"=w2425:u16[], "output_underThreshold"=w2414:bool)  [unwired: 9 in]
                  n735 = Select(t=w2428, s=w2414, f=myRIO_BRig_RT__Case_Exp_stateList."FreeRewardPost_pre" ("Enum")) -> (s? t:f=w2426:T2)
                  n736 = And(x=w2414, y=w2415) -> (x .and. y?=w2413:bool)
                  n737 = And(x=w2413, y=w2420) -> (x .and. y?=w2418:bool)
                  n738 = And(x=w2413, y=w2421) -> (x .and. y?=w2419:bool)
                }
                frame "FreeRewardPost" {
                  n739 = call "BRig_RT__Case_Exp__generic__incrementCountTilThreshold.vi"("input_dataCurrent"=w2435) -> ("output_dataCurrent"=w2434:u16[], "output_underThreshold"=w2433:bool)  [unwired: 9 in]
                  n740 = Select(t=w2438, s=w2433, f=myRIO_BRig_RT__Case_Exp_stateList."initTrial" ("Enum")) -> (s? t:f=w2436:T2)
                }
                frame "FreeRewardPost_pre" {
                  n741 = call "BRig_dataExp_T_RewardPost.vi"() -> ("output_T_RewardPost"=w2448:i32)  [unwired: 11 in]
                  n742 = call "BRig_dataCurrent_c_generic.vi"() -> ("output_count_generic"=w2451:i32)  [unwired: 11 in]
                  n743 = call "BRig_dataCurrent_T_generic.vi"() -> ("output_T_generic"=w2450:i32)  [unwired: 11 in]
                  n744 = Index Array(array=w2445, index=w2448) -> (element=w2447:u16)
                  n745 = Replace Array Subset(array=w2446, new element #1=u16 0 ("new element/subarray"), index #1=w2451, new element #2=w2447, index #2=w2450) -> (w2444:u16[])
                }
              }
              n746 = call "BRig_RT_panel_manualTriggering_v0,90.vi"("input_dataMTrig"=w1312) -> ("output_Solenoid_R"=w1323:bool, "output_Solenoid_L"=w1322:bool, "output_dataMTrig"=w1355:u16[], "output_Audio_L"=w1354:bool, "output_Audio_R"=w1353:bool, "output_CueLed"=w1351:bool, "output_Laser_l1"=w1327:bool, "output_Laser_l2"=w1347:bool)  [unwired: 11 in]
              n747 = call "BRig_RT__Case_Exp__comm_tcp__data_other.vi"("input_strState"=w1315, "input_strAccum"=w1316, "input_error"=w1317, "input_hTCP"=w1318, "input_I_connected_TCP"=w1319) -> ("output_strAccum"=w1298:string, "output_error"=w1297:errorcluster, "output_hTCP"=w1299:refnum<k5>, "output_I_connect_TCP"=w1300:bool)  [unwired: 3 in]
              n748 = Or(x="STOP_abort", y=w1339) -> (x .or. y?=w1301:bool)
              n749 = Or(x=w1352, y=w1351) -> (x .or. y?=w1330:bool)
              n750 = local read "Laser1_LED"() -> (w1288:bool)
              n751 = local read "Laser2_LED"() -> (w1287:bool)
              n752 = Or(x=w1354, y=w1369) -> (x .or. y?=w1329:bool)
              n753 = Or(x=w1368, y=w1353) -> (x .or. y?=w1328:bool)
              n754 = Or(x=w1326, y=w1327) -> (x .or. y?=w1346:bool)
              n755 = Or(x=w1350, y=w1347) -> (x .or. y?=w1348:bool)
              n756 = call "BRig_RT__Case_Exp__recordLick.vi"("input_dataLick"=w1338, "input_lick__R"=w1332, "input_lick__L"=w1333, "input_lick"=w1334, "intput_state__trialStart"=w1292, "intput_state__trialEnd"=w1337, "input_dataCurrent"=w1336) -> ("output_dataLick"=w1331:u16[][], "output_dataCurrent"=w1335:u16[])  [unwired: 7 in]
              n757 = xnode "Read/Write Control"("FPGA VI Reference In"=w1367, "error in"=w1366, "L1Led_ON"=w1288, "L2Led_ON"=w1287, "Solenoid_trig_L"=w1321, "Solenoid_trig_R"=w1320, "A3_SL"=w1322, "A1_SR"=w1323, "LC_Event_l1"=w1345, "LC_Laser_l1"=w1346, "LC_Event_l2"=w1349, "LC_Laser_l2"=w1348, "CueLed_Event"=w1330, "audioTrigger_L"=w1329, "audioTrigger_R"=w1328) -> ("FPGA VI Reference Out"=w1373:refnum<k20>, "error out"=w1372:errorcluster, "fpga_laser1"=w1286:bool, "fpga_laser2"=w1285:bool, "fpga_solenoid_L"=w1284:bool, "fpga_solenoid_R"=w1283:bool, "AnaIn_0"=w1313:u16, "AnaIn_1"=w1314:u16)
              n758 = local write "Laser1"(w1286) -> ()
              n759 = local write "Laser2"(w1285) -> ()
              n760 = local write "Solenoid L"(w1284) -> ()
              n761 = local write "Solenoid R"(w1283) -> ()
              n762 = call "BRig_RT__Case_Exp__recordAnalogInput__PortA__fifo__1value.vi"("input_iOccurence"=w1343, "resetOccurrence"=w1342, "input_dataCurrent"=w1336, "input_iState_start"=w1292, "rt fifo"=w1291, "input_iState_end"=w1337, "input_fifo_error"=w1290, "input_AI1"=w1314, "input_AI0"=w1313) -> ("output_fifo_error"=w1296:errorcluster, "output_iOccurrence"=w1344:u16)  [unwired: 8 in, 1 out]
              n763 = call "BRig_RT_timeLoop_Exp__noStateLimit.vi"("input_error"=w1296, "input_Threshold_reset"="input_Threshold_reset", "input_Threshold"=w1358, "input_timestamp"=w1359, "input_state"=w1292) -> ("output_Threshold"=w1356:bool, "output_duration"=→"tLoop":dbl)  [unwired: 4 in, 1 out]
              "Threshold" <- w1356
              n764 = node-c288() -> ()  [unwired: 1 in, 1 out]
            }
            "stop_TimedLoop" <- w897
            n765 = while {
              tunnel: w841 -> [w965]
              tunnel: w840 -> [w964]
              shift-right: [w959] -> _
              shift-left: 0 ("element") -> [w960]
              shift-right: [w955] -> _
              shift-left: w846 -> [w961]
              tunnel: [w958] -> w843
              tunnel: [w957] -> w842
              tunnel: w839 -> [w954]
              tunnel: w838 -> [w953]
              tunnel: [w952] -> w837
              tunnel: [w951] -> w836
              shift-right: [w949] -> _
              shift-left: FALSE -> [w950]
              stop <- w948 stop-if-true
              # "timed out?"
              n766 = RT FIFO Read(0:w965, 3:w964) -> (8:w958:refnum<k33>, 9:w962:u16, 10:w969:bool, 11:w966:errorcluster)  [unwired: 2 in, 1 out]
              n767 = Unbundle By Name(w966) -> ("code"=w970:i32)
              n768 = Not(x=w969) -> (.not. x?=w968:bool)
              n769 = Equal To 0?(x=w970) -> (x = 0?=w967:bool)
              n770 = And(x=w967, y=w968) -> (x .and. y?=w963:bool)
              n771 = Select(t=w966, s=w967, f=w964) -> (s? t:f=w957:errorcluster)
              n772 = case shown="True" w963 {
                tunnel: w962 -> [_ w1001]
                tunnel: w961 -> [w993 w1003]
                tunnel: w960 -> [w992 w1000]
                tunnel: [w993 w1002] -> w955
                tunnel: [w992 w996] -> w959
                tunnel: [_ w994] -> w956
                frame False {
                }
                frame True {
                  n773 = Replace Array Subset(array=w1003, new element=w1001, index=w1000) -> (w1002:u16[])
                  n774 = Increment(x=w1000) -> (x+1=w998:i32)
                  n775 = Less?(x=w1000, y=7 ("dimension size")) -> (x < y?=w995:bool)
                  n776 = Select(t=w998, s=w995, f=0) -> (s? t:f=w996:i32)
                  n777 = Not(x=w995) -> (.not. x?=w994:bool)
                }
              }
              n778 = case shown="True" w956 {
                tunnel: w955 -> [_ w982]
                tunnel: w954 -> [w973 w981]
                tunnel: w953 -> [w972 w980]
                tunnel: [w973 w978] -> w952
                tunnel: [w972 w977] -> w951
                tunnel: w950 -> [w971 w975]
                tunnel: [w971 w974] -> w949
                frame False {
                }
                frame True {
                  n779 = for {
                    N: 8 -> [_]
                    tunnel: w982 -> [w989] mode=indexing
                    tunnel: w981 -> [w991]
                    tunnel: w980 -> [w990]
                    shift-right: [w984] -> w976
                    shift-left: FALSE -> [w988]
                    tunnel: [w987] -> w978
                    tunnel: [w986] -> w977
                    n780 = shared-variable-write(w991, w990, w989) -> (w987:refnum<k21>, w986:errorcluster, w985:bool)  [unwired: 1 in]
                    n781 = Or(x=w988, y=w985) -> (x .or. y?=w984:bool)
                  }
                  n782 = Or(x=w975, y=w976) -> (x .or. y?=w974:bool)
                }
              }
              n783 = local read "stop_TimedLoop"() -> (w948:bool)
            }
            n784 = while {
              shift-right: [w1074] -> _
              shift-left: 0 -> [w1063]
              tunnel: w894 -> [w1081]
              tunnel: w886 -> [w1083]
              shift-right: [w1070] -> _
              shift-left: 0 -> [w1065]
              shift-right: [w1075] -> _
              shift-left: w833 -> [w1082]
              shift-right: [w1071] -> _
              shift-left: w861 -> [w1084]
              shift-right: [w1078] -> w883
              shift-left: w855 -> [w1091]
              shift-right: [w1079] -> w877
              shift-left: w854 -> [w1085]
              tunnel: w858 -> [w1068]
              tunnel: w862 -> [w1067]
              shift-right: [w1056] -> _
              shift-left: w828 -> [w1062]
              shift-right: [w1055] -> _
              shift-left: 0 -> [w1061]
              tunnel: w831 -> [w1059]
              tunnel: w830 -> [w1060]
              tunnel: [w1054] -> w825
              tunnel: [w1053] -> w824
              stop <- w1092 stop-if-true
              # "nColumns dataBlock"
              # "nColumns dataTrial"
              # "buffer_dataTrial"
              # "buffer_dataBlock"
              # "buffer_dataTrial"
              # "buffer_dataBlock"
              n785 = local read "stop_TimedLoop"() -> (w1092:bool)
              n786 = Not Equal To 0?(x=w1065) -> (x != 0?=w1066:bool)
              n787 = Not Equal To 0?(x=w1061) -> (x != 0?=w1052:bool)
              n788 = case shown="True" w1066 {
                tunnel: w1084 -> [w1244 w1247]
                tunnel: w1065 -> [w1245 w1249]
                tunnel: w1083 -> [_ w1258]
                tunnel: [w1245 w1246] -> w1072
                tunnel: [w1244 w1247] -> w1073
                frame False {
                }
                frame True {
                  n789 = Array Subset(array=w1247, length (row)=w1249) -> (w1260:u16[][])  [unwired: 3 in]
                  n790 = call "BRig_dataBlock_iBlock.vi"() -> ("output_iBlock"=w1255:i32)  [unwired: 11 in]
                  n791 = Index Array(array=w1247, index (row)=0, index (col)=w1255) -> (element=w1254:u16)
                  n792 = To Double Precision Float(number=w1260) -> (double precision float=w1259:dbl[][])
                  n793 = Not Equal?(x=u16 1, y=w1254) -> (x != y?=w1252:bool)
                  n794 = call-poly <vilib>:"Write To Spreadsheet File.vi"("delimiter (\\t)"="," ("delimiter (\\t)"), "append to file? (new file:F)"=w1252, "2D data"=w1259, "file path (dialog if empty)"=w1258) -> ("new file path (Not A Path if cancelled)"=w1251:path)  [unwired: 4 in]
                  n795 = call <vilib>:"Is Path and Not Empty.vi"("path"=w1251) -> ("Is Path and Not Empty?"=w1250:bool)  [unwired: 4 in]
                  n796 = Select(t=0, s=w1250, f=w1249) -> (s? t:f=w1246:i32)
                }
              }
              n797 = case shown="True" w1052 {
                tunnel: w1062 -> [w1096 w1105]
                tunnel: w1061 -> [w1095 w1098]
                tunnel: [w1095 w1104] -> w1057
                tunnel: [w1096 w1105] -> w1058
                tunnel: w1060 -> [w1094 w1113]
                tunnel: w1059 -> [w1093 w1112]
                tunnel: [w1094 w1103] -> w1054
                tunnel: [w1093 w1102] -> w1053
                frame False {
                }
                frame True {
                  n798 = Decrement(x=w1098) -> (x-1=w1097:i32)
                  n799 = Multiply(x=w1097, y=2 ("index")) -> (x*y=w1099:i32)
                  n800 = Increment(x=w1099) -> (x+1=w1100:i32)
                  n801 = Index Array(array=w1105, index #1=w1099, index #2=w1100) -> (element #1=w1111:u16, element #2=w1107:u16)
                  n802 = shared-variable-write(w1113, w1112, w1111) -> (w1108:refnum<k21>, w1109:errorcluster, w1110:bool)  [unwired: 1 in]
                  n803 = case shown="False" w1110 {
                    selector: w1110 -> [_ w1122]
                    tunnel: w1109 -> [w1119 w1120]
                    tunnel: w1108 -> [w1118 w1121]
                    tunnel: w1107 -> [w1117 _]
                    tunnel: [w1116 w1122] -> w1106
                    tunnel: [w1115 w1121] -> w1103
                    tunnel: [w1114 w1120] -> w1102
                    frame False {
                      n804 = shared-variable-write(w1118, w1119, w1117) -> (w1115:refnum<k21>, w1114:errorcluster, w1116:bool)  [unwired: 1 in]
                    }
                    frame True {
                    }
                  }
                  n805 = Select(t=w1098, s=w1106, f=w1097) -> (s? t:f=w1104:i32)
                }
              }
              n806 = RT FIFO Read(0:w1091, 3:w1085) -> (8:w1078:refnum<k33>, 9:w1069:u16[], 10:w1089:bool, 11:w1086:errorcluster)  [unwired: 2 in, 1 out]
              n807 = Unbundle By Name(w1086) -> ("code"=w1090:i32)
              n808 = Not(x=w1089) -> (.not. x?=w1088:bool)
              n809 = Equal To 0?(x=w1090) -> (x = 0?=w1087:bool)
              n810 = And(x=w1087, y=w1088) -> (x .and. y?=w1080:bool)
              n811 = Select(t=w1086, s=w1087, f=w1085) -> (s? t:f=w1079:errorcluster)
              n812 = Not Equal To 0?(x=w1063) -> (x != 0?=w1064:bool)
              n813 = case shown="True" w1064 {
                tunnel: w1082 -> [w1227 w1230]
                tunnel: w1063 -> [w1228 w1232]
                tunnel: w1081 -> [_ w1241]
                tunnel: [w1228 w1229] -> w1076
                tunnel: [w1227 w1230] -> w1077
                frame False {
                }
                frame True {
                  n814 = Array Subset(array=w1230, length (row)=w1232) -> (w1243:u16[][])  [unwired: 3 in]
                  n815 = call "BRig_dataTrial_nTrial.vi"() -> ("output_nTrial"=w1238:i32)  [unwired: 11 in]
                  n816 = Index Array(array=w1230, index (row)=0, index (col)=w1238) -> (element=w1237:u16)
                  n817 = To Double Precision Float(number=w1243) -> (double precision float=w1242:dbl[][])
                  n818 = Not Equal?(x=u16 1, y=w1237) -> (x != y?=w1235:bool)
                  n819 = call-poly <vilib>:"Write To Spreadsheet File.vi"("delimiter (\\t)"="," ("delimiter (\\t)"), "append to file? (new file:F)"=w1235, "2D data"=w1242, "file path (dialog if empty)"=w1241) -> ("new file path (Not A Path if cancelled)"=w1234:path)  [unwired: 4 in]
                  n820 = call <vilib>:"Is Path and Not Empty.vi"("path"=w1234) -> ("Is Path and Not Empty?"=w1233:bool)  [unwired: 4 in]
                  n821 = Select(t=0, s=w1233, f=w1232) -> (s? t:f=w1229:i32)
                }
              }
              n822 = case shown="True" w1080 {
                tunnel: w1077 -> [w1129 w1149]
                tunnel: w1076 -> [w1128 w1147]
                tunnel: [w1129 w1148] -> w1075
                tunnel: [w1128 w1146] -> w1074
                tunnel: w1073 -> [w1127 w1145]
                tunnel: w1072 -> [w1126 w1143]
                tunnel: [w1127 w1144] -> w1071
                tunnel: [w1126 w1142] -> w1070
                tunnel: w1069 -> [_ w1150]
                tunnel: w1068 -> [_ w1141]
                tunnel: w1067 -> [_ w1140]
                tunnel: w1058 -> [w1124 w1133]
                tunnel: w1057 -> [w1123 w1132]
                tunnel: [w1124 w1131] -> w1056
                tunnel: [w1123 w1130] -> w1055
                frame False {
                  n823 = Wait (ms)(milliseconds to wait=u32 10) -> ()  [unwired: 1 out]
                }
                frame True {
                  n824 = Index Array(array=w1150, index=0) -> (element=w1134:u16)
                  n825 = Equal?(x=w1134, y=u16 1) -> (x = y?=w1135:bool)
                  n826 = Equal?(x=w1134, y=u16 2) -> (x = y?=w1137:bool)
                  n827 = Or(x=w1135, y=w1137) -> (x .or. y?=w1136:bool)
                  n828 = case shown="False" w1136 {
                    tunnel: w1150 -> [w1158 w1206]
                    tunnel: w1149 -> [w1162 w1199]
                    tunnel: [w1162 w1198] -> w1148
                    tunnel: w1147 -> [w1161 w1197]
                    tunnel: [w1161 w1196] -> w1146
                    tunnel: w1145 -> [w1160 w1203]
                    tunnel: [w1160 w1201] -> w1144
                    tunnel: w1143 -> [w1159 w1202]
                    tunnel: [w1159 w1200] -> w1142
                    tunnel: w1141 -> [_ w1205]
                    tunnel: w1140 -> [_ w1204]
                    tunnel: w1135 -> [_ w1195]
                    tunnel: w1134 -> [w1163 _]
                    tunnel: w1133 -> [w1155 w1194]
                    tunnel: w1132 -> [w1156 w1193]
                    tunnel: [w1154 w1194] -> w1131
                    tunnel: [w1153 w1193] -> w1130
                    frame False {
                      n829 = Equal?(x=w1163, y=u16 3) -> (x = y?=w1152:bool)
                      n830 = case shown="True" w1152 {
                        tunnel: w1158 -> [_ w1170]
                        tunnel: w1156 -> [w1164 w1169]
                        tunnel: w1155 -> [w1165 w1168]
                        tunnel: [w1165 w1167] -> w1154
                        tunnel: [w1164 w1166] -> w1153
                        frame False {
                        }
                        frame True {
                          w1177 = 3 ("y")
                          n831 = Array Size(array=w1170) -> (size(s)=w1171:i32)
                          n832 = To Double Precision Float(number=w1171) -> (double precision float=w1172:dbl)
                          n833 = To Double Precision Float(number=w1177) -> (double precision float=w1176:dbl)
                          n834 = Divide(x=w1172, y=w1176) -> (x/y=w1173:dbl)
                          n835 = Round Toward -Infinity(1:w1173) -> (0:w1174:dbl)
                          n836 = To Long Integer(number=w1174) -> (32bit integer=w1175:i32)
                          n837 = for {
                            N: w1175 -> [_]
                            tunnel: w1177 -> [w1192]
                            tunnel: w1170 -> [w1189]
                            shift-right: [w1178] -> w1166
                            shift-left: w1169 -> [w1184]
                            shift-right: [w1179] -> w1167
                            shift-left: w1168 -> [w1186]
                            i -> [w1191]
                            n838 = Multiply(x=2 ("index"), y=w1184) -> (x*y=w1183:i32)
                            n839 = Multiply(x=w1191, y=w1192) -> (x*y=w1190:i32)
                            n840 = Increment(x=w1190) -> (x+1=w1188:i32)
                            n841 = Increment(x=w1188) -> (x+1=w1187:i32)
                            n842 = Increment(x=w1184) -> (x+1=w1178:i32)
                            n843 = Index Array(array=w1189, index #1=w1188, index #2=w1187) -> (element #1=w1181:u16, element #2=w1180:u16)
                            n844 = Increment(x=w1183) -> (x+1=w1182:i32)
                            n845 = Replace Array Subset(array=w1186, new element #1=w1181, index #1=w1183, new element #2=w1180, index #2=w1182) -> (w1179:u16[])
                          }
                        }
                      }
                    }
                    frame True {
                      n846 = case shown="True" w1195 {
                        tunnel: w1206 -> [w1214 w1226]
                        tunnel: w1205 -> [w1212 _]
                        tunnel: w1204 -> [_ w1221]
                        tunnel: w1203 -> [w1216 w1220]
                        tunnel: w1202 -> [w1215 w1222]
                        tunnel: [w1216 w1219] -> w1201
                        tunnel: [w1215 w1218] -> w1200
                        tunnel: w1199 -> [w1211 w1223]
                        tunnel: [w1209 w1223] -> w1198
                        tunnel: w1197 -> [w1208 w1217]
                        tunnel: [w1207 w1217] -> w1196
                        frame True {
                          n847 = Array Subset(array=w1214, index=1, length=w1212) -> (w1210:u16[])
                          n848 = Increment(x=w1208) -> (x+1=w1207:i32)
                          n849 = Replace Array Subset(array=w1211, new element=w1210, index (row)=w1208) -> (w1209:u16[][])  [unwired: 1 in]
                        }
                        frame False {
                          n850 = Array Subset(array=w1226, index=1, length=w1221) -> (w1224:u16[])
                          n851 = Increment(x=w1222) -> (x+1=w1218:i32)
                          n852 = Replace Array Subset(array=w1220, new element=w1224, index (row)=w1222) -> (w1219:u16[][])  [unwired: 1 in]
                        }
                      }
                    }
                  }
                }
              }
            }
            n853 = node-c288(w946) -> ()  [unwired: 1 out]
            n854 = RT FIFO Delete(0:w883, 2:TRUE ("force destroy? (F)"), 3:w877) -> ()  [unwired: 1 out]
            n855 = RT FIFO Delete(0:w843, 2:TRUE ("force destroy? (F)"), 3:w842) -> ()  [unwired: 1 out]
            n856 = flat-sequence {
              tunnel: w917 -> [w1262]
              tunnel: w916 -> [w1265]
              tunnel: w915 -> [w1264]
              tunnel: w914 -> [w1263]
              tunnel: w913 -> [w1267]
              tunnel: w911 -> [_]
              tunnel: w834 -> [w1269]
              tunnel: w881 -> [w1268]
              tunnel: [w1261] -> w892
              tunnel: w877 -> [_]
              tunnel: w910 -> [w1280]
              tunnel: w909 -> [w1279]
              tunnel: w908 -> [w1278]
              tunnel: [w1277] -> w907
              tunnel: [w1276] -> w906
              tunnel: [w1271] -> w902
              tunnel: w892 -> [w1270]
              frame #0 {
                # "Store"
                n857 = call "BRig_RT__Case_Exp__storeData__endExp__v5__p1.vi"("input_dataCurrent"=w1263, "input_dataLC"=w1268, "input_dataExp"=w1269, "input_dataExp_end"=w1264, "input_dataLC_end"=w1265) -> ("output_True"=w1266:bool)  [unwired: 10 in]
                n858 = call "BRig_RT__Case_Exp__storeData__endExp__v5__p2.vi"("input_dataCurrent"=w1263, "input_dataLick"=w1267, "input_True"=w1266, "input_dataMTrig"=w1262) -> ("output_True"=w1261:bool)  [unwired: 11 in]
              }
              frame #1 {
                # "Send"
                n859 = local read "Data Set Prefix"() -> (w1272:string)
                n860 = call "BRig_RT_comm_webdav_upload_all__v3.vi"("input_I_connected_webdav"=w1278, "input_fileName_prefix"=w1272, "input_hSession"=w1279, "input_error"=w1280, "input_True"=w1270) -> ("output_hSession"=w1276:T4, "error out"=w1277:errorcluster, "output_nFilenames"=w1273:i32, "output_arrFilenames"=w1274:string[], "output_uploaded"=w1275:bool[], "output_strCmd"=w1271:string)  [unwired: 5 in]
                n861 = call "BRig_RT_comm_webdav_upload_all_warnUser.vi"("input_n"=w1273, "input_arrFilenames"=w1274, "input_arrUploaded"=w1275) -> ()  [unwired: 9 in]
              }
            }
            n862 = flat-sequence {
              tunnel: w926 -> [w1281]
              tunnel: [w1281] -> w912
              frame #0 {
                w1282 = FALSE ("START")
                n863 = local write "START"(w1282) -> ()
                n864 = local write "STOP_endTrial"(w1282) -> ()
                n865 = local write "STOP_endBlock"(w1282) -> ()
              }
            }
            n866 = xnode "Read/Write Control"("FPGA VI Reference In"=w943, "error in"=w912, "Counts_Reset"=TRUE, "audioTrigger_L"=w929, "audioFreq_L_kHz"=w927, "audioAmp_L"=w928, "audioTrigger_R"=w929, "audioFreq_R_kHz"=w927, "audioAmp_R"=w928, "A3_SL"=w929, "A1_SR"=w929, "A6_Act"=w929) -> ("FPGA VI Reference Out"=w942:refnum<k20>, "error out"=w911:errorcluster)
            n867 = call "BRig_RT__Case_Exp__comm_tcp__data_other.vi"("input_strState"=w902, "input_strAccum"="" ("f"), "input_error"=w903, "input_hTCP"=w904, "input_I_connected_TCP"=w905) -> ("output_error"=w898:errorcluster, "output_hTCP"=w899:refnum<k5>, "output_I_connect_TCP"=w900:bool)  [unwired: 3 in, 1 out]
          }
        }
        n868 = local read "STOP_abort"() -> (w328:bool)
      }
    }
  }
  n869 = flat-sequence {
    tunnel: w96 -> [w2466]
    tunnel: w95 -> [w2468]
    tunnel: w89 -> [w2467]
    tunnel: [w2467] -> w101
    tunnel: [w2466] -> w100
    tunnel: [w2465] -> w99
    tunnel: w74 -> [w2464]
    tunnel: [w2464] -> w98
    tunnel: w75 -> [w2463]
    tunnel: [w2463] -> w97
    tunnel: w82 -> [w2461]
    tunnel: w81 -> [w2460]
    tunnel: w80 -> [w2459]
    tunnel: w76 -> [w2462]
    tunnel: [w2462] -> w94
    tunnel: w93 -> [_]
    tunnel: [w2461] -> w88
    tunnel: [w2460] -> w87
    tunnel: [w2459] -> w86
    tunnel: w101 -> [w2488]
    tunnel: w100 -> [w2487]
    tunnel: w99 -> [w2486]
    tunnel: [w2485] -> _
    tunnel: w98 -> [w2484]
    tunnel: w97 -> [w2483]
    tunnel: w94 -> [w2482]
    tunnel: w88 -> [w2481]
    tunnel: w87 -> [w2480]
    tunnel: w86 -> [w2479]
    frame #0 {
      # "Stop FPGA\nSend QUIT to Host"
      n870 = case shown="True" w2467 {
        tunnel: w2466 -> [_ w2477]
        tunnel: w2468 -> [w2474 w2476]
        tunnel: [w2474 w2475] -> w2465
        frame False {
        }
        frame True {
          n871 = xnode "Read/Write Control"("FPGA VI Reference In"=w2477, "error in"=w2476, "FPGA_Stop"=TRUE) -> ("error out"=w2475:errorcluster)  [unwired: 1 out]
        }
      }
      n872 = case shown="True" w2461 {
        tunnel: w2460 -> [_ w2473]
        tunnel: w2459 -> [_ w2472]
        frame False {
        }
        frame True {
          w2469 = "<S,Q><S,Q><S,Q><S,Q>" ("input_packet")
          n873 = call "BRig_RT_comm_tcp_write_RTwrite.vi"("input_error"=w2472, "input_packet"=w2469, "input_hTCP"=w2473) -> ("output_error"=w2471:errorcluster, "output_hTCP"=w2470:refnum<k5>)  [unwired: 5 in, 2 out]
          n874 = call "BRig_RT_comm_tcp_write_RTwrite.vi"("input_error"=w2471, "input_packet"=w2469, "input_hTCP"=w2470) -> ()  [unwired: 5 in, 4 out]
        }
      }
    }
    frame #1 {
      # "Disconnect FPGA\nDisconnect comm webdav"
      n875 = case shown="True" w2488 {
        tunnel: w2486 -> [w2493 w2496]
        tunnel: w2487 -> [_ w2495]
        tunnel: [w2493 w2494] -> w2485
        frame False {
        }
        frame True {
          n876 = xnode "Close FPGA VI Reference"("FPGA VI Reference In"=w2495, "error in"=w2496) -> ("error out"=w2497:errorcluster)
          n877 = call <vilib>:"Reset myRIO.vi"("error in (no error)"=w2497) -> ("error out"=w2494:errorcluster)  [unwired: 10 in]
        }
      }
      n878 = case shown="True" w2481 {
        tunnel: w2480 -> [_ w2490]
        tunnel: w2479 -> [_ w2489]
        frame False {
        }
        frame True {
          n879 = TCP Close Connection(connection ID=w2490, error in (no error)=w2489) -> ()  [unwired: 1 in, 2 out]
        }
      }
      n880 = case shown="True" w2484 {
        tunnel: w2483 -> [_ w2492]
        tunnel: w2482 -> [_ w2491]
        frame False {
        }
        frame True {
          n881 = call <vilib>:"Close Session.vi"("session handle"=w2492, "error in (no error)"=w2491) -> ()  [unwired: 13 in, 1 out]
        }
      }
    }
  }
  n882 = Flush Stream(8:w1, 11:w2) -> (0:w3:errorcluster, 3:w4:refnum<k21>)  [unwired: 2 in, 1 out]
  n883 = Flush Stream(8:w13, 11:w14) -> (0:w15:errorcluster, 3:w16:refnum<k21>)  [unwired: 2 in, 1 out]
  n884 = Destroy Stream Endpoint(8:w3, 11:w4) -> ()  [unwired: 1 out]
  n885 = Destroy Stream Endpoint(8:w15, 11:w16) -> ()  [unwired: 1 out]
